vi "Rb_HSRL_v1.0.vi"() -> ()   [LabVIEW 2012]
uses:
  C:/Users/H2ODial/Desktop/Shared Telescope WV DIAL Code/Libraries and VIs/PowerMeterCommands.dll
  Shared Telescope WV DIAL Code/Libraries and VIs/PowerMeterCommands.dll
  <vilib>/DAQmx/write.llb/DAQmx Write (Digital 1D Bool NChan 1Samp 1Line).vi
  <vilib>/DAQmx/miscellaneous.llb/DAQmx Fill In Error Info.vi
  <vilib>/Analysis/baseanly.llb/Mean (DBL).vi
  NCAR_DIAL_Labview/AMCS_Data.vi
  Libraries and VIs/Scalar_Data.vi
  <vilib>/Analysis/NI_AALBase.lvlib
  Libraries and VIs/Scalar_Data_2.vi
  Libraries and VIs/Scalar_Data_4.vi
  Libraries and VIs/Scalar_Data_3.vi
  Shared Telescope WV DIAL Code/bristol/CLDevIFace.dll
panel:
  out "FileHour":i32
  out "L_Count":i32=1074
  out "sigma_off_total":dbl[](array[numeric])=[1.743240222676567e-29, 1.7305064234520192e-29, 1.7178428488017876e-29, 1.705249234754588e-29, 1.692725317927625e-29, 1.6802708355255098e-29, 1.6678855253392072e-29, 1.6555691257449675e-29, 1.643321375703259e-29, 1.631142014757713e-29, 1.619030783034076e-29, 1.6069874212391396e-29, 1.5950116706597008e-29, 1.5831032731615155e-29, 1.5712619711882448e-29, 1.5594875077604192e-29, 1.5477796264743928e-29, 1.536138071501325e-29, 1.5245625875861102e-29, 1.5130529200463784e-29, 1.5016088147714616e-29, 1.4902300182213635e-29, 1.4789162774257317e-29, 1.4676673399828526e-29, 1.4564829540586228e-29, 1.4453628683855395e-29, 1.4343068322617087e-29, 1.423314595549802e-29, 1.412385908676087e-29, 1.401520522629413e-29, 1.3907181889602167e-29, 1.3799786597795178e-29, 1.3693016877579533e-29, 1.3586870261247614e-29, 1.3481344286668248e-29, 1.3376436497276693e-29, 1.3272144442065002e-29, 1.3168465675572225e-29, 1.306539775787476e-29, 1.2962938254576631e-29, 1.2861084736799932e-29, 1.275983478117514e-29, 1.2659185969831725e-29, 1.255913589038839e-29, 1.2459682135943853e-29, 1.2360822305067216e-29, 1.226255400178859e-29, 1.2164874835589805e-29, 1.2067782421394965e-29, 1.1971274379561291e-29, 1.1875348335869746e-29, 1.178000192151585e-29, 1.1685232773100587e-29, 1.159103853262107e-29, 1.1497416847461672e-29, 1.1404365370384833e-29, 1.1311881759522077e-29, 1.1219963678364997e-29, 1.1128608795756442e-29, 1.1037814785881385e-29, 1.0947579328258326e-29, 1.0857900107730373e-29, 1.0768774814456401e-29, 1.0680201143902449e-29, 1.059217679683288e-29, 1.050469947930196e-29, 1.0417766902645026e-29, 1.0331376783470095e-29, 1.0245526843649219e-29, 1.0160214810310171e-29, 1.0075438415827858e-29, 9.991195397816067e-30, 9.907483499119049e-30, 9.824300467803266e-30, 9.741644057149123e-30, 9.659512025642775e-30, 9.577902136968061e-30, 9.496812159998168e-30, 9.416239868787793e-30, 9.336183042565099e-30, 9.256639465723581e-30, 9.177606927814325e-30, 9.099083223538087e-30, 9.021066152737376e-30, 8.94355352038878e-30, 8.866543136595263e-30, 8.790032816578293e-30, 8.714020380670432e-30, 8.638503654307654e-30, 8.563480468021747e-30, 8.488948657432945e-30, 8.414906063242409e-30, 8.34135053122489e-30, 8.268279912221336e-30, 8.195692062131722e-30, 8.123584841907613e-30, 8.051956117545193e-30, 7.980803760078008e-30, 7.910125645569903e-30, 7.839919655108038e-30, 7.77018367479582e-30, 7.700915595746074e-30, 7.632113314074101e-30, 7.563774730890895e-30, 7.49589775229633e-30, 7.42848028937248e-30, 7.361520258176989e-30, 7.295015579736328e-30, 7.228964180039413e-30, 7.163363990030974e-30, 7.098212945605153e-30, 7.03350898759913e-30, 6.969250061786685e-30, 6.905434118872086e-30, 6.84205911448366e-30, 6.779123009167796e-30, 6.716623768382682e-30, 6.654559362492305e-30, 6.592927766760486e-30, 6.531726961344797e-30, 6.470954931290802e-30, 6.410609666526129e-30, 6.350689161854694e-30, 6.291191416951005e-30, 6.232114436354457e-30, 6.173456229463735e-30, 6.1152148105312555e-30, 6.05738819865764e-30, 5.999974417786303e-30, 5.942971496698029e-30, 5.88637746900568e-30, 5.830190373148922e-30, 5.774408252388966e-30, 5.71902915480344e-30, 5.664051133281335e-30, 5.609472245517892e-30, 5.555290554009665e-30, 5.501504126049601e-30, 5.448111033722145e-30, 5.395109353898468e-30, 5.342497168231712e-30, 5.290272563152322e-30, 5.238433629863349e-30, 5.186978464335997e-30, 5.135905167305021e-30, 5.085211844264311e-30, 5.0348966054625156e-30, 4.984957565898723e-30, 4.935392845318121e-30, 4.886200568207903e-30, 4.837378863793033e-30, 4.788925866032188e-30, 4.74083971361372e-30, 4.693118549951716e-30, 4.6457605231820746e-30, 4.598763786158649e-30, 4.552126496449484e-30, 4.5058468163330804e-30, 4.45992291279475e-30, 4.4143529575229735e-30, 4.369135126905908e-30, 4.3242676020278865e-30, 4.279748568665977e-30, 4.2355762172866776e-30, 4.191748743042563e-30, 4.148264345769089e-30, 4.1051212299814194e-30, 4.0623176048712705e-30, 4.019851684303927e-30, 3.97772168681519e-30, 3.935925835608487e-30, 3.894462358551995e-30, 3.853329488175855e-30, 3.812525461669358e-30, 3.772048520878381e-30, 3.7318969123026464e-30, 3.692068887093256e-30, 3.6525627010501435e-30, 3.613376614619627e-30, 3.574508892892104e-30, 3.535957805599667e-30, 3.497721627113887e-30, 3.459798636443609e-30, 3.422187117232841e-30, 3.384885357758682e-30, 3.3478916509293096e-30, 3.311204294282027e-30, 3.274821589981408e-30, 3.2387418448174616e-30, 3.2029633702038674e-30, 3.16748448217627e-30, 3.1323035013906723e-30, 3.097418753121829e-30, 3.0628285672617353e-30, 3.028531278318176e-30, 2.994525225413349e-30, 2.9608087522825017e-30, 2.92738020727268e-30, 2.8942379433414807e-30, 2.861380318055985e-30, 2.8288056935915537e-30, 2.7965124367308904e-30, 2.7644989188630092e-30, 2.7327635159823654e-30, 2.7013046086879812e-30, 2.6701205821826584e-30, 2.6392098262722643e-30, 2.60857073536503e-30, 2.5782017084709586e-30, 2.5481011492012757e-30, 2.518267465767932e-30, 2.48869907098315e-30, 2.459394382259084e-30, 2.4303518216074538e-30, 2.4015698156393544e-30, 2.373046795564983e-30, 2.3447811971935587e-30, 2.3167714609331835e-30, 2.2890160317908673e-30, 2.261513359372517e-30, 2.2342618978830647e-30, 2.207260106126574e-30, 2.180506447506479e-30, 2.1539993900258164e-30, 2.1277374062875614e-30, 2.1017189734949946e-30, 2.075942573452137e-30, 2.050406692564209e-30, 2.0251098218382186e-30, 2.0000504568835075e-30, 1.97522709791245e-30, 1.9506382497411197e-30, 1.9262824217900777e-30, 1.90215812808518e-30, 1.8782638872584395e-30, 1.8545982225489656e-30, 1.8311596618039416e-30, 1.8079467374796337e-30, 1.7849579866425135e-30, 1.7621919509703503e-30, 1.7396471767534394e-30, 1.7173222148958272e-30, 1.695215620916613e-30, 1.6733259549512735e-30, 1.6516517817530943e-30, 1.6301916706945917e-30, 1.608944195769015e-30, 1.587907935591907e-30, 1.5670814734026938e-30, 1.5464633970663293e-30, 1.5260522990750085e-30, 1.5058467765498978e-30, 1.4858454312429449e-30, 1.466046869538705e-30, 1.4464497024562426e-30, 1.4270525456510766e-30, 1.4078540194171561e-30, 1.3888527486888854e-30, 1.3700473630432205e-30, 1.3514364967017896e-30, 1.3330187885330481e-30, 1.3147928820545087e-30, 1.2967574254349875e-30, 1.2789110714969318e-30, 1.2612524777187339e-30, 1.2437803062371468e-30, 1.2264932238497042e-30, 1.209389902017198e-30, 1.1924690168662101e-30, 1.1757292491916402e-30, 1.159169284459339e-30, 1.1427878128087242e-30, 1.1265835290554763e-30, 1.110555132694241e-30, 1.0947013279014056e-30, 1.0790208235378844e-30, 1.063512333151953e-30]
  out "sigma_on_total":dbl[](array[numeric])=[2.4340017477146767e-23, 2.4274412818663494e-23, 2.420732288097601e-23, 2.4138763171607075e-23, 2.4068749611971555e-23, 2.3997298524358964e-23, 2.3924426624079916e-23, 2.3850151008686397e-23, 2.3774489143132373e-23, 2.3697458852913156e-23, 2.36190783110143e-23, 2.3539366026312405e-23, 2.3458340830704462e-23, 2.3376021868838044e-23, 2.3292428585503507e-23, 2.3207580713450583e-23, 2.3121498259428018e-23, 2.3034201496227212e-23, 2.2945710944104806e-23, 2.2856047362675843e-23, 2.2765231738320447e-23, 2.2673285267646947e-23, 2.2580229349833727e-23, 2.248608556893553e-23, 2.2390875685659293e-23, 2.2294621622467176e-23, 2.2197345450376258e-23, 2.2099069377470227e-23, 2.1999815736348355e-23, 2.1899606971079585e-23, 2.1798465624791464e-23, 2.169641432790326e-23, 2.1593475784788012e-23, 2.14896727633276e-23, 2.1385028081251008e-23, 2.1279564594830037e-23, 2.1173305187714593e-23, 2.1066272759361542e-23, 2.0958490211415564e-23, 2.084998043979143e-23, 2.0740766320851033e-23, 2.0630870703286357e-23, 2.0520316394136837e-23, 2.0409126151062488e-23, 2.029732266933444e-23, 2.0184928575611705e-23, 2.0071966414278353e-23, 1.995845864002376e-23, 1.9844427607378718e-23, 1.9729895562122156e-23, 1.9614884633458083e-23, 1.949941682266462e-23, 1.9383513996314403e-23, 1.9267197878653387e-23, 1.9150490042628342e-23, 1.903341190278002e-23, 1.8915984707328566e-23, 1.8798229531581053e-23, 1.868016727054153e-23, 1.8561818633359694e-23, 1.844320413541846e-23, 1.83243440938274e-23, 1.8205258619529394e-23, 1.8085967614344843e-23, 1.796649076411767e-23, 1.7846847532669082e-23, 1.772705716009478e-23, 1.7607138654671335e-23, 1.748711079164774e-23, 1.736699210720163e-23, 1.724680089518985e-23, 1.712655520363638e-23, 1.7006272832450093e-23, 1.6885971328406567e-23, 1.676566798384533e-23, 1.6645379834582855e-23, 1.6525123654654852e-23, 1.64049159581075e-23, 1.6284772994189594e-23, 1.6164710746660405e-23, 1.6044744932804177e-23, 1.592489100169575e-23, 1.5805164132216785e-23, 1.568557923455707e-23, 1.556615094674276e-23, 1.544689363604575e-23, 1.5327821398683183e-23, 1.5208948058333225e-23, 1.5090287167129152e-23, 1.4971852006339355e-23, 1.4853655585856495e-23, 1.473571064476312e-23, 1.4618029653368368e-23, 1.4500624811408796e-23, 1.4383508052135306e-23, 1.4266691041242847e-23, 1.4150185179015395e-23, 1.4034001601711465e-23, 1.3918151181804494e-23, 1.380264453258343e-23, 1.3687492006081647e-23, 1.3572703697882705e-23, 1.3458289448210642e-23, 1.334425884233711e-23, 1.323062121559879e-23, 1.3117385653560717e-23, 1.3004560994740862e-23, 1.2892155833393701e-23, 1.2780178521172943e-23, 1.2668637170454652e-23, 1.2557539657303056e-23, 1.2446893622178752e-23, 1.233670647459471e-23, 1.2226985395093895e-23, 1.2117737338433009e-23, 1.2008969034936782e-23, 1.1900686995645521e-23, 1.1792897514105055e-23, 1.1685606668968417e-23, 1.1578820327003693e-23, 1.1472544147196505e-23, 1.1366783583055892e-23, 1.1261543884626321e-23, 1.1156830104040547e-23, 1.105264709614388e-23, 1.0948999523006647e-23, 1.0845891856006974e-23, 1.0743328380652776e-23, 1.0641313197997005e-23, 1.053985022811714e-23, 1.0438943213901274e-23, 1.0338595723501814e-23, 1.0238811153778875e-23, 1.0139592733083218e-23, 1.004094352498993e-23, 9.942866430738372e-24, 9.845364192310422e-24, 9.748439395492984e-24, 9.652094473529007e-24, 9.556331709814775e-24, 9.46115323999935e-24, 9.366561056469104e-24, 9.272557009807764e-24, 9.179142813204785e-24, 9.086320043893727e-24, 8.99409014719721e-24, 8.902454438513804e-24, 8.811414107270266e-24, 8.7209702177534e-24, 8.631123714110481e-24, 8.541875421413822e-24, 8.453226049192974e-24, 8.365176194357096e-24, 8.277726342238635e-24, 8.190876871321929e-24, 8.104628054224402e-24, 8.018980061019835e-24, 7.933932961475672e-24, 7.849486727271008e-24, 7.76564123493127e-24, 7.682396268209798e-24, 7.59975151947134e-24, 7.517706593480449e-24, 7.436261008471844e-24, 7.355414199356734e-24, 7.275165518527386e-24, 7.1955142399073e-24, 7.116459559687598e-24, 7.038000598677644e-24, 6.960136404824994e-24, 6.882865955014892e-24, 6.806188156632044e-24, 6.730101850609514e-24, 6.65460581162548e-24, 6.579698751718169e-24, 6.505379321481059e-24, 6.4316461112652594e-24, 6.358497654002827e-24, 6.285932426130069e-24, 6.213948849912267e-24, 6.142545294327772e-24, 6.071720077707449e-24, 6.001471468939084e-24, 5.9317976881000545e-24, 5.862696910102476e-24, 5.7941672637438124e-24, 5.726206835260677e-24, 5.658813668292153e-24, 5.591985766579753e-24, 5.525721094088758e-24, 5.460017577095787e-24, 5.394873105681451e-24, 5.330285534503123e-24, 5.266252684077375e-24, 5.202772342694521e-24, 5.139842266622448e-24, 5.077460182290799e-24, 5.0156237866223426e-24, 4.954330748813029e-24, 4.893578710949848e-24, 4.8333652890974455e-24, 4.773688074662277e-24, 4.714544635557992e-24, 4.655932516447053e-24, 4.597849240182404e-24, 4.540292309191013e-24, 4.483259205518585e-24, 4.42674739232282e-24, 4.370754314606057e-24, 4.315277399935558e-24, 4.2603140594233714e-24, 4.205861688673324e-24, 4.151917668300883e-24, 4.098479364843186e-24, 4.045544131381291e-24, 3.993109308279057e-24, 3.941172224403115e-24, 3.8897301970479374e-24, 3.838780532877164e-24, 3.788320529066769e-24, 3.738347472966815e-24, 3.6888586436966916e-24, 3.639851312259568e-24, 3.59132274213381e-24, 3.543270189847801e-24, 3.495690905760268e-24, 3.448582134258885e-24, 3.401941114510703e-24, 3.355765080859501e-24, 3.310051263532474e-24, 3.2647968887967694e-24, 3.219999179434413e-24, 3.175655355707198e-24, 3.1317626351721278e-24, 3.0883182332206364e-24, 3.045319363885891e-24, 3.002763239842466e-24, 2.9606470728961763e-24, 2.9189680744537877e-24, 2.8777234556990287e-24, 2.8369104281330918e-24, 2.7965262038221122e-24, 2.756567995816512e-24, 2.7170330182075216e-24, 2.677918486705564e-24, 2.6392216190184846e-24, 2.6009396347182876e-24, 2.5630697559473515e-24, 2.52560920743859e-24, 2.4885552169425194e-24, 2.451905015320653e-24, 2.415655836797415e-24, 2.3798049195052113e-24, 2.3443495052514497e-24, 2.3092868400499548e-24, 2.274614174185544e-24, 2.24032876263913e-24, 2.2064278649970267e-24, 2.1729087457232614e-24, 2.139768674486092e-24, 2.107004926331989e-24, 2.0746147815906223e-24, 2.0425955263802693e-24, 2.0109444525036206e-24, 1.9796588577379595e-24, 1.9487360460458536e-24, 1.9181733275318523e-24, 1.887968018650247e-24, 1.858117442578046e-24, 1.8286189289240917e-24, 1.799469814155742e-24, 1.7706674416008516e-24, 1.742209161621556e-24, 1.7140923316697854e-24, 1.6863143164506015e-24, 1.658872488023585e-24, 1.6317642257456694e-24]
  out "background start":u32=254
  in  "Tab Control 2":enum32{"WV ND narrow", "WV ND wide"}(tab)=enum."WV ND wide"
  out "Water Vapor Number Density":dbl[][](graph)=[[nan, nan, nan, nan, nan, nan, nan, nan, nan, nan, nan, nan, nan, nan, nan, nan, nan, nan, nan, nan, nan, nan, nan, nan, nan, nan, nan, nan, nan, nan, nan, nan, nan, nan, nan, nan, nan, nan, nan, nan, nan, nan, nan, nan, nan, nan, nan, nan, nan, nan, nan, nan, nan, nan, nan, nan, nan, nan, nan, nan, nan, nan, nan, nan, nan, nan, nan, nan, nan, nan, nan, nan, nan, nan, nan, nan, nan, nan, nan, nan, nan, nan, nan, nan, nan, nan, nan, nan, nan, nan, nan, nan, nan, nan, nan, nan, nan, nan, nan, nan, nan, nan, nan, nan, nan, nan, nan, nan, nan, nan, nan, nan, nan, nan, nan, nan, nan, nan, nan, nan, nan, nan, nan, nan, nan, nan, nan, nan, nan, nan, nan, nan, nan, nan, nan, nan, nan, nan, nan, nan, nan, nan, nan, nan, nan, nan, nan, nan, nan, nan, nan, nan, nan, nan, nan, nan, nan, nan, nan, nan, nan, nan, nan, nan, nan, nan, nan, nan, nan, nan, nan, nan, nan, nan, nan, nan, nan, nan, nan, nan, nan, nan, nan, nan, nan, nan, nan, nan, nan, nan, nan, nan, nan, nan, nan, nan, nan, nan, nan, nan, nan, nan, nan, nan, nan, nan, nan, nan, nan, nan, nan, nan, nan, nan, nan, nan, nan, nan, nan, nan, nan, nan, nan, nan, nan, nan, nan, nan, nan, nan, nan, nan, nan, nan, nan, nan, nan, nan, nan, nan, nan, nan, nan, nan, nan, nan, nan, nan, nan, nan, nan, nan, nan, nan, nan, nan, nan, nan, nan, nan, nan, nan, nan, nan, nan, nan, nan, nan, nan, nan, nan, nan, nan, nan, nan, nan, 0.0, 0.0, 0.0, 0.0]]
  out "Water Vapor Number Density 2":dbl[][](graph)=[[-4.895620784344141, -1.6968761345752499, -1.6565574205993407, -0.7910986719149671, 0.45141531234214655, 0.26569889383172274, 0.252782855220571, 0.5170092395121896, 0.6376366522322393, 0.5993479288564648, 0.6058560998386514, 0.684546234269247, 0.6235793613938562, 0.5332655312275792, 0.5321964157932958, 0.4070943470032037, 0.22619083292346856, 0.25267455894454416, 0.08444579003837588, -0.13682052767692168, -0.09862987130915078, -0.017768894386159955, 0.05643569551164931, -0.08094018405996439, -0.19480945286341145, -0.06075864848776602, 0.06572189033635885, 0.039671145716655434, -0.09019678979226083, -0.25137434776459894, -0.3103489478521125, -0.08024943893293456, 0.06423439301048192, 0.13797237185068356, 0.09652097666493928, -0.27218358000621307, -0.185543414642533, 0.1438017744018525, 0.08765450079199422, -0.03345732408225611, 0.00604196903795461, 0.08267162189631926, 0.08321350242218584, -0.012409724836985615, 0.09179545659027583, 0.6459182960375515, 2.2714138304504465, 4.472080283472494, 6.069123607220832, 6.990920567565342, 7.36854640140037, 7.533827768908647, 7.78681047271232, 8.16977657612961, 8.33947543641484, 8.20492227081218, 7.344734807648823, 5.975728267693901, 4.780051696796776, 3.7740123495138187, 2.9280932285169685, 2.0539593404341003, 1.0507395625011602, 0.24983625755292468, -0.03087360168049576, -0.09871712906759823, -0.5243136500273711, -1.1240686267268338, -1.2357380560289242, -1.4422719214455215, -2.433215702684351, -3.945832400189159, -5.949204291924275, -8.114157844867002, -9.494648146574068, -10.507339423422904, -10.700994135914522, -10.9541924360514, -11.159957626803134, -10.310413019639286, -8.273713586301556, -4.9233609203087365, -1.3825921417412714, 1.9712668900617927, 3.378743922387925, 4.088541358207288, 4.007098488107816, 4.103753213551659, 4.2340431790887845, 4.002951543204611, 3.686717068344896, 2.676317251371432, 1.8649247581896786, 1.0769258052139539, 0.994629537649367, 0.9943831824592358, 1.1926416452348065, 1.5853553556197177, 2.2148625502201704, 3.108204242971333, 4.52975221279031, 6.563140206581805, 9.134431370789654, 10.09902536825411, 7.280234451114133, 10.0523524768224, 11.397964614531503, -9.731550990663491, -17.06321734883455, -11.458184267120643, -9.0017850283161, -13.74567942179605, -16.166537362978502, -18.718196579771735, -9.35381042912264, -12.348971539301585, -12.154938420119997, 5.238619214813352, 9.192709199582309, 14.003999057719604, -0.06779931634937152, 35.617669964692475, 0.04457992374851296, -8.90741561387052, -3.9461882542526, 14.504294890545367, -0.8727026085664153, -0.35102394306834434, 3.597665203572956, -8.777831693534882, -2.954362505813555, -31.9195126702593, -3.8409008890464578, 5.435252259671796, 4.418087258470408, -20.27746959744448, -10.613666063696122, 1.8615584996987187, -7.892452743589819, -16.226094846188996, -2.383169027908074, 16.92726357878285, 5.456643076920959, 14.024204963031833, -11.157368068562498, 4.340391398015347, 3.9438279618064525, 21.09263715399934, 7.680640751435989, -20.993550633072697, -8.585857017075819, -23.52761555750025, -7.7605319523907905, -17.998320270316242, -16.180858157616544, -12.33853742715028, -14.667064184492856, -49.95610957313421, -49.44749566095738, 10.699739375836488, 23.683479637440108, 31.061894932072992, -21.207052348393276, 10.140128391398383, -19.895810174476523, -15.108621152086325, 4.704826625608483, 27.735652107472575, 39.49510870780125, 20.618532855965775, -1.6111370074131892, -12.831734806604826, 15.629932803094974, -14.611823636038348, 29.640524053991733, 5.015161743310881, -15.51797368973543, -40.44577289799667, -0.39722724524646463, -0.9239222044621952, -20.535732365469173, -65.2480323448027, 26.487995182823845, 19.394999803340337, 20.191997873478407, -2.0265210169772954, 24.853618849595346, 42.52208295164487, 12.786859480359054, 4.75017526225865, 17.835930493267455, 52.68824174794205, 34.72243662831497, 6.3260469161335555, -7.486867031209662, 10.759083285233261, -66.51368343207345, -9.431641653132534, -18.76468287635854, -15.650517009171523, -20.26681276234243, -28.565738365359984, -30.121388986694676, -11.448382080381739, -7.859271932595647, 39.94633068089728, 56.860646041958226, 4.524084628014805, 54.8901924570308, 16.546300340318517, 20.97522561665681, 0.05393176717682176, -15.507692065561, -1.4043208940216665, -28.371460993902787, -29.792326994117683, -15.657302207635121, 0.7422373766833459, -20.485527759325585, -8.147758064164341, 18.82463653057326, 28.412517069974978, 8.44635419576539, -41.650375728538094, -5.872699418390108, 1.8094667524442931, 1.5468215804437708, 41.021758843667016, -23.195386516298573, 112.29420310200375, -16.587822198800488, 2.3654789897656885, -23.460726710726124, 91.52185335985529, 22.81580178981554, 27.176228351401313, -5.556802132037837, -63.630574940001445, 17.09067007327093, -40.44093778205592, -14.862030911568922, -43.05400894140326, -66.35104817070908, -65.39879656619192, 1.787225500718848, -42.55071677898285, -1.0319246177540415, 25.14429634118871, -1.541432028680571, -11.550238337108132, 11.139244631605925, 40.46635926020925, 127.44307434312368, -10.216664862682935, 11.539137763811313, 53.24251481088911, 71.08979732730369, 9.04286335401417, -73.54684338479775, -128.0577139180142, -86.77985430271906, -75.66005818218412, -37.36514333604306, 5.847510175807278, 19.206208021208408, -129.3901968796948, -67.23722677793343, -51.592749749275896, 98.36383603903877, 82.4204245579684, 78.16287004109239, 71.76344715659785, -14.203962783305958, 19.040423726184862, -15.217180976533145, 88.48290659710524, 0.0, 0.0, 0.0, 0.0]] caption="Water Vapor Number Density"
  out "RingBuffer offline near":dbl[][](array[numeric])
  out "RingBuffer aerosol near":dbl[][](array[numeric])
  in  "?":T1(tab)=enum."Raw Counts combined"
  out "NRB":dbl[][](graph) caption="Water Vapor Number Density"
  out "NRB 2":dbl[][](graph)=[[0.0001380506377637834, 0.00037231338536795606, 0.0008267018556340546, 0.0016491182628392146, 0.0030984002727663757, 0.0054670319322802745, 0.008975049813494944, 0.013862611097666086, 0.020640714712243713, 0.030032261963369757, 0.041790885354449886, 0.05646823982524779, 0.07405765547049918, 0.09445230634842686, 0.11873844907566593, 0.14619202991112218, 0.176128716495472, 0.2065930967214025, 0.23772953608021488, 0.2712999788026663, 0.303183374769058, 0.33461849194542187, 0.36556675325880467, 0.3928286709332662, 0.4196893863731421, 0.4471637143514717, 0.47287194470451144, 0.4890446444671604, 0.5073163767400038, 0.527833117627229, 0.5384928838328282, 0.5504358197236068, 0.5590875545865447, 0.5635018660373124, 0.5701363166467346, 0.5747236095368302, 0.5814440483526132, 0.5919810946272498, 0.5989836077128905, 0.6020509020058386, 0.6120157766394789, 0.6121904103347232, 0.6014357977759414, 0.6025641696641967, 0.6063884095863453, 0.6028169859903434, 0.5986429081300412, 0.602926751521262, 0.6045234286166641, 0.6020772298885957, 0.6093012321904592, 0.6071420602133842, 0.6000004559925828, 0.6074015253593915, 0.6308874815821919, 1.447719815623411, 5.0092251256615326, 10.608207780798377, 12.51719597789648, 9.217607568444715, 8.012447829214926, 15.43698184887009, 26.6065389573323, 30.108057890606787, 25.881596466733146, 22.37376849180048, 20.71552585543168, 17.29780957584456, 13.067263761054791, 9.970369103635118, 8.373569316919895, 8.097534835118013, 8.865992103907578, 12.770957329400636, 18.09781429592472, 17.53337121539854, 10.90234029608704, 5.0392553254119274, 2.373505404868523, 1.0991203310287527, 0.45466930792063653, 0.28635282734262657, 0.2684584174682796, 0.27254175669170166, 0.2642432011850105, 0.27155612117614053, 0.3573074050799282, 0.5675591029962431, 0.9568718981502712, 1.8781004463984938, 3.832184351648157, 7.296157287404594, 12.992486225144889, 19.850044811959783, 23.876263508247536, 22.89971699362709, 18.57735815186402, 13.384467836450757, 9.941618607703871, 9.52963656189712, 9.878467461835443, 7.9906667301038645, 4.637172445889551, 2.3432986610499698, 1.878226967282488, 2.3880704072998435, 3.002081888496057, 3.3688062310053652, 3.1265041118362116, 2.369963919278849, 1.4049354414439597, 0.5981477861656775, 0.2201236171481549, 0.10053280018296205, 0.1049539926912024, 0.13605859526889652, 0.14285523134540867, 0.10850858158417578, 0.11616513852327509, 0.14725243241889766, 0.09034956192428265, 0.05961502498241574, 0.08744308907061056, 0.12774569879993047, 0.10342822758481597, 0.10781611837641128, 0.10691828988405683, 0.09844828534015804, 0.13126962561795, 0.10477355228922058, 0.08314270506167556, 0.11068192501635618, 0.1469623872315277, 0.08836483775676496, 0.10655458852918881, 0.15225529874509575, 0.08430787264863451, 0.07009979544767103, 0.08181048165478563, 0.06279693670038371, 0.09328596080458845, 0.09038165610259435, 0.08327020474676582, 0.025684897874086683, 0.0009707833337049407, 0.10225629353341592, 0.1005694755351202, 0.14729024890638545, 0.12365825337171389, 0.025079453252945572, 0.028677777816976682, 0.027515990565747148, 0.054454687532889845, 0.04453495073347162, 0.017382194343326905, -0.04252219295217604, -0.07058050401235756, -0.02456764397335006, -0.028497208807347345, 0.015346829492512202, 0.04298797788120953, 0.01623362898624638, 0.08563204153282877, 0.004064284667093428, -0.10133064618333942, 0.05253453070798904, 0.06514225667556629, 0.042499199608995515, 0.09968168750325075, 0.004918514915909139, -0.00032358694526253486, 0.06289222078475586, 0.059342770479511635, 0.13657348927840832, 0.1770073767458159, 0.07264829002326911, 0.08483375293471081, 0.21365900428087206, 0.04152199871116299, 0.0222051701557016, 0.15278405108610074, 0.1415202788910293, 0.14467720700616699, 0.1294668069955981, 0.09953241260822868, 0.05077385822206056, 0.11437335389791674, 0.0174792549892461, -0.12170754523984625, -0.024506540953794162, -0.006320084684789309, -0.03276198538429077, 0.004207338523473438, 0.013227107986545533, 0.06523808909079482, -0.024979323976464695, -0.04263554157486385, 0.07698508208616586, 0.0006951280918226639, -0.09660263950948868, -0.03937413525317987, 0.06805955659081427, 0.05222342809633812, -0.12035517959868296, -0.1708478846518318, 0.0023642220353940827, 0.14259926575817566, 0.08083030570322937, -0.127577324988055, -0.16119409412364716, 0.06364108456905275, 0.3386672374669003, 0.2622252302230505, 0.07857050698230215, 0.12340568076001972, 0.05734592250065322, 0.08977349820396631, 0.22616670263325436, 0.07953961680339071, -0.18706894477447125, -0.2018189311229299, -0.08047192233842872, 0.07250896970261306, 0.12342245188602205, 0.13225442113834784, 0.12368717459399005, 0.09676342875464072, 0.008847199978845019, -0.06111354456473662, 0.049880628408371486, 0.08951323251928896, 0.034320613803925794, -0.04514061816559589, -0.01470972019166381, 0.005184082507240442, 0.025418931716203685, 0.0733253763222838, 0.08853584410979902, 0.15903378151183248, 0.22466106785463236, 0.11627032735247014, 0.02672784970245174, 0.10243485082245009, 0.007292657881859975, -0.020133574716629028, 0.11652624886483087, 0.05810881426073248, 0.03511053047002674, 0.13003259048413732, 0.05118148463654222, 0.13814021686570216, 0.15620654066824666, -0.10085146919722136, -0.10903579404468894, 0.02347325591345995, 0.11868986701645191, 0.19775337697257164, 0.2786752450542533, 0.24564109985016588, 0.12565244407857296, 0.03303914164600584, 0.08306213435353355, -0.005384461142077131, 0.00853717219386779, 0.10239382246508076, -0.11215691172352353, -0.12932346222779006, -0.12686812690414423, -0.22859894560534677, -0.26090034021168024, -0.2817521949784425, -0.06575148455597245, 0.19185794565702205, 0.29998635760771497, 0.06048668116730433, -0.09822080237649826, -0.12528467918807926, 0.0, 0.0, 0.0]] caption="Water Vapor Number Density"
  out "raw counts":dbl[][](graph) caption="Water Vapor Number Density"
  out "raw counts near":dbl[][](graph)=[[155.92000000000002, 92.92, 94.92, 74.92, 108.92, 117.92, 192.92000000000002, 173.92000000000002, 224.92000000000002, 239.92000000000002, 293.92, 374.92, 383.92, 427.92, 461.92, 541.92, 520.92, 526.92, 632.92, 656.92, 621.92, 635.92, 638.92, 660.92, 601.92, 587.92, 584.92, 592.92, 532.92, 566.92, 510.92, 531.92, 507.92, 460.92, 445.92, 423.92, 421.92, 367.92, 395.92, 372.92, 322.92, 356.92, 319.92, 280.92, 302.92, 259.92, 269.92, 242.92000000000002, 283.92, 255.92000000000002, 230.92000000000002, 198.92000000000002, 184.92000000000002, 194.92000000000002, 212.92000000000002, 198.92000000000002, 351.92, 1825.92, 2550.92, 1728.92, 1368.92, 3407.92, 6903.92, 11887.92, 13882.92, 13623.92, 13034.92, 9068.92, 5196.92, 4147.92, 2973.92, 1874.92, 1142.92, 1749.92, 5473.92, 8307.92, 6691.92, 3420.92, 1268.92, 430.92, 101.92, 24.92, 25.92, 2.9200000000000017, 8.920000000000002, 12.920000000000002, 15.920000000000002, 68.92, 102.92, 98.92, 72.92, 61.92, 121.92, 223.92000000000002, 518.92, 774.92, 840.92, 877.92, 844.92, 591.92, 303.92, 266.92, 194.92000000000002, 165.92000000000002, 141.92000000000002, 111.92, 112.92, 124.92, 206.92000000000002, 202.92000000000002, 149.92000000000002, 24.92, 14.920000000000002, 15.920000000000002, 2.9200000000000017, -6.079999999999998, -13.079999999999998, 0.9200000000000017, -19.08, 11.920000000000002, -16.08, 10.920000000000002, -0.0799999999999983, 7.920000000000002, 10.920000000000002, 11.920000000000002, -4.079999999999998, 26.92, -6.079999999999998, 12.920000000000002, 13.920000000000002, -7.079999999999998, 7.920000000000002, 9.920000000000002, 15.920000000000002, -3.0799999999999983, 1.9200000000000017, -4.079999999999998, 14.920000000000002, 2.9200000000000017, -4.079999999999998, -7.079999999999998, 2.9200000000000017, 6.920000000000002, 7.920000000000002, 2.9200000000000017, -2.0799999999999983, 1.9200000000000017, 15.920000000000002, -3.0799999999999983, -9.079999999999998, 11.920000000000002, 7.920000000000002, -12.079999999999998, 5.920000000000002, 3.9200000000000017, -7.079999999999998, -0.0799999999999983, -24.08, -5.079999999999998, 4.920000000000002, -6.079999999999998, 3.9200000000000017, -14.079999999999998, -1.0799999999999983, -6.079999999999998, -7.079999999999998, 3.9200000000000017, 5.920000000000002, 6.920000000000002, 12.920000000000002, 15.920000000000002, -0.0799999999999983, -0.0799999999999983, -0.0799999999999983, -7.079999999999998, -0.0799999999999983, 2.9200000000000017, -22.08, -1.0799999999999983, 4.920000000000002, 1.9200000000000017, -10.079999999999998, -8.079999999999998, 7.920000000000002, 17.92, 1.9200000000000017, -2.0799999999999983, -1.0799999999999983, -7.079999999999998, 3.9200000000000017, -4.079999999999998, 0.9200000000000017, -2.0799999999999983, -10.079999999999998, 0.9200000000000017, 4.920000000000002, 9.920000000000002, -21.08, 19.92, -12.079999999999998, 1.9200000000000017, -8.079999999999998, -7.079999999999998, 29.92, -4.079999999999998, -2.0799999999999983, -0.0799999999999983, -6.079999999999998, -1.0799999999999983, -8.079999999999998, -4.079999999999998, -6.079999999999998, 1.9200000000000017, 6.920000000000002, 12.920000000000002, 2.9200000000000017, 8.920000000000002, -0.0799999999999983, 8.920000000000002, -12.079999999999998, -11.079999999999998, -1.0799999999999983, 4.920000000000002, -1.0799999999999983, 12.920000000000002, -3.0799999999999983, 17.92, -4.079999999999998, -12.079999999999998, 0.9200000000000017, -18.08, 4.920000000000002, 19.92, 11.920000000000002, -14.079999999999998, -3.0799999999999983, 2.9200000000000017, -4.079999999999998, 8.920000000000002, 12.920000000000002, -0.0799999999999983, -6.079999999999998, -15.079999999999998, -4.079999999999998, 3.9200000000000017, 8.920000000000002, -2.0799999999999983, -6.079999999999998, -6.079999999999998, -0.0799999999999983, -3.0799999999999983, 0.9200000000000017, 5.920000000000002, -17.08, 16.92, 8.920000000000002, -7.079999999999998, -17.08, -3.0799999999999983, -3.0799999999999983, 1.9200000000000017, -4.079999999999998, -12.079999999999998, -3.0799999999999983, -5.079999999999998, 7.920000000000002, 1.9200000000000017, 5.920000000000002, 10.920000000000002, 6.920000000000002, -2.0799999999999983, 9.920000000000002, -22.08, -3.0799999999999983, 12.920000000000002, -3.0799999999999983, 15.920000000000002, 1.9200000000000017, 0.0]] caption="Water Vapor Number Density"
  out "HSRL combined Smoothed":dbl[](array[numeric])=[122.52406779661018, 82.63423728813558, 81.54949152542372, 91.49864406779659, 110.00711864406779, 134.76983050847457, 162.51559322033893, 192.14271186440672, 225.99016949152536, 266.2613559322033, 306.11728813559307, 347.45627118644063, 388.1596610169492, 426.73593220338995, 467.17661016949165, 505.3969491525425, 539.2274576271188, 564.0664406779663, 582.4732203389833, 599.8376271186443, 607.9732203389831, 611.3800000000001, 611.1088135593222, 603.1342372881356, 593.8969491525424, 585.0749152542376, 573.7783050847459, 551.8630508474578, 533.7528813559325, 518.9901694915256, 495.9477966101696, 475.82915254237304, 454.5325423728815, 431.6427118644069, 412.18508474576277, 392.7952542372882, 376.24440677966106, 363.2020338983051, 348.93084745762707, 333.4393220338982, 322.6511864406778, 307.5918644067795, 288.3376271186439, 275.92237288135584, 265.4901694915253, 252.60033898305076, 240.31220338983042, 232.066440677966, 223.29525423728808, 213.60033898305082, 207.77830508474574, 199.1681355932203, 189.48169491525417, 184.78677966101685, 185.01559322033887, 408.8545762711863, 1355.8630508474578, 2744.3969491525413, 3120.5240677966085, 2236.863050847457, 1886.142711864407, 3475.625762711865, 5703.541016949153, 6228.642711864408, 5231.007118644069, 4413.651186440678, 3978.659661016948, 3243.346101694914, 2394.930847457627, 1783.6850847457629, 1459.659661016949, 1373.4901694915252, 1461.9477966101695, 2040.447796610169, 2798.8884745762707, 2643.8037288135592, 1613.964745762712, 731.8037288135594, 336.9986440677966, 152.3884745762711, 61.53254237288135, 37.8206779661017, 34.60881355932203, 34.30372881355932, 32.48169491525423, 32.60881355932203, 41.922372881355926, 65.07491525423728, 107.22745762711862, 205.6596610169491, 409.84610169491526, 761.4477966101695, 1321.3969491525422, 1966.5833898305082, 2309.9562711864405, 2171.820677966102, 1731.464745762712, 1226.7698305084746, 895.108813559322, 841.2783050847459, 854.8037288135595, 678.8461016949154, 387.1766101694916, 192.1850847457627, 151.16813559322026, 188.54101694915238, 232.5325423728812, 256.08338983050834, 233.3630508474575, 173.7698305084745, 101.21898305084744, 42.34610169491525, 15.3122033898305, 6.871525423728807, 7.049491525423722, 8.98169491525423, 9.26983050847457, 6.922372881355925, 7.286779661016943, 9.083389830508468, 5.48169491525423, 3.557966101694908, 5.134237288135585, 7.379999999999992, 5.879999999999992, 6.032542372881348, 5.888474576271179, 5.33762711864406, 7.0071186440677895, 5.5071186440677895, 4.303728813559315, 5.642711864406772, 7.379999999999992, 4.371525423728806, 5.193559322033892, 7.312203389830502, 3.9901694915254167, 3.269830508474569, 3.7613559322033825, 2.8461016949152467, 4.168135593220331, 3.98169491525423, 3.617288135593213, 1.10033898305084, 0.041016949152534954, 4.261355932203382, 4.134237288135585, 5.973220338983044, 4.947796610169485, 0.9901694915254163, 1.117288135593213, 1.0579661016949078, 2.0664406779660944, 1.6681355932203314, 0.6427118644067722, -1.5522033898305159, -2.5437288135593294, -0.8742372881356006, -1.0013559322033974, 0.5325423728813486, 1.4732203389830434, 0.5494915254237214, 2.8630508474576195, 0.13423728813558577, -3.3064406779661093, 1.693559322033891, 2.074915254237281, 1.3376271186440605, 3.10033898305084, 0.1511864406779586, -0.009830508474583777, 1.888474576271179, 1.7613559322033823, 4.0071186440677895, 5.134237288135585, 2.083389830508467, 2.4054237288135516, 5.990169491525416, 1.1511864406779586, 0.6088135593220265, 4.142711864406772, 3.7952542372881277, 3.8376271186440603, 3.3969491525423656, 2.5833898305084677, 1.303728813559315, 2.905423728813552, 0.43932203389829794, -3.0267796610169566, -0.6030508474576346, -0.1538983050847531, -0.7894915254237362, 0.10033898305084002, 0.31220338983050105, 1.5240677966101621, -0.5776271186440753, -0.975932203389838, 1.7444067796610097, 0.015593220338975589, -2.145423728813567, -0.8657627118644142, 1.4816949152542298, 1.1257627118643994, -2.5691525423728887, -3.6115254237288212, 0.04949152542372137, 2.9562711864406706, 1.659661016949145, -2.5945762711864484, -3.2471186440678044, 1.269830508474569, 6.693559322033892, 5.134237288135586, 1.524067796610162, 2.371525423728806, 1.0918644067796537, 1.693559322033891, 4.227457627118637, 1.4732203389830434, -3.433559322033906, -3.670847457627126, -1.4505084745762786, 1.2952542372881282, 2.1850847457627043, 2.3206779661016874, 2.1511864406779586, 1.6681355932203317, 0.15118644067795883, -1.035254237288143, 0.8376271186440604, 1.4901694915254162, 0.5664406779660943, -0.7386440677966176, -0.23864406779661762, 0.08338983050846716, 0.40542372881355193, 1.159661016949145, 1.388474576271179, 2.4732203389830434, 3.464745762711857, 1.778305084745755, 0.4054237288135519, 1.541016949152535, 0.10881355932202652, -0.29796610169492266, 1.7105084745762638, 0.8461016949152468, 0.5071186440677892, 1.8630508474576197, 0.7274576271186366, 1.9477966101694841, 2.1850847457627047, -1.39966101694916, -1.5013559322033971, 0.3206779661016875, 1.6088135593220265, 2.659661016949145, 3.7189830508474504, 3.252881355932196, 1.6511864406779586, 0.4308474576271112, 1.0749152542372808, -0.0691525423728887, 0.10881355932202652, 1.2952542372881282, -1.4081355932203465, -1.611525423728821, -1.5691525423728887, -2.8064406779661093, -3.1793220338983126, -3.4081355932203463, -0.7894915254237364, 2.2867796610169417, 3.549491525423721, 0.7105084745762635, -1.145423728813567, -1.4505084745762789]
  out "HSRL combined":dbl[](array[numeric])=[119.4261281337048, 78.36345403899722, 76.88852367688021, 84.97626740947078, 99.26874651810589, 120.4929805013928, 145.6754317548747, 173.4052367688022, 205.19910863509745, 240.32306406685228, 275.8216713091921, 311.40941504178255, 347.9275208913647, 384.22835654596076, 420.13782729804996, 452.82724233983276, 483.6238997214483, 508.8954874651808, 525.5751532033423, 540.406629526462, 549.05844011142, 552.4135933147627, 551.1127576601666, 545.0152646239549, 537.4498050139271, 527.0709749303617, 514.3425626740944, 497.5375487465179, 481.84534818941484, 466.1030083565458, 447.07236768802215, 428.8453481894149, 409.98880222841206, 392.01526462395526, 374.77431754874635, 358.59465181058476, 342.9748746518104, 325.6447910863508, 309.66568245125325, 296.1141504178271, 283.4860167130918, 271.5946518105849, 260.49437325905285, 249.32445682451242, 239.1183286908077, 228.75481894150408, 217.58072423398323, 209.111364902507, 200.30077994428973, 192.29242339832865, 191.79799442896933, 212.02779944289688, 329.6336490250693, 665.0988300835652, 1321.1266852367696, 2589.597437325907, 4572.029192200557, 6343.986016713094, 6717.097437325907, 5722.538941504177, 4317.65454038997, 3405.1211142061265, 3110.9122005571026, 3012.2005013927574, 2982.5528690807814, 2950.566796657383, 2719.9442339832876, 2279.3954874651827, 1801.5250139275772, 1446.0890807799442, 1301.6099721448472, 1291.0194428969364, 1265.1628969359335, 1249.6433983286913, 1205.8105292479113, 969.1475766016715, 595.8704178272978, 291.88852367687997, 131.91637883008357, 62.34116991643454, 37.90941504178271, 33.119721448467956, 31.722785515320325, 30.622506963788283, 31.557047353760417, 34.85231197771584, 39.364846796657346, 47.45676880222838, 65.65036211699166, 120.88016713091926, 295.68378830083566, 716.1030083565456, 1338.9498050139273, 1910.671253481894, 2205.417771587743, 2176.7297493036212, 1962.703286908078, 1754.2548189415038, 1632.6656824512534, 1575.9108077994429, 1543.0486908077992, 1459.7032869080774, 1281.72557103064, 1063.7896378830078, 856.0445125348186, 663.7269637883005, 505.5208356545959, 389.2659610027854, 286.6447910863509, 181.88295264623946, 91.19075208913647, 34.18796657381618, 10.810529247910864, 3.3857381615598845, 1.1684679665738122, 2.0041225626740906, 3.5570473537604412, 2.150362116991639, 1.8940947075208867, 2.3801671309192156, 3.1030083565459567, 3.3550974930362076, 3.3954874651810543, 4.8049582172701895, 3.1698607242339785, 2.068189415041778, 2.5319777158774324, 2.336991643454035, 1.7743175487465142, 0.5236211699164305, 2.4191643454038956, 2.9665181058495773, 2.118328690807795, 1.314707520891361, 1.4372701949860678, 1.534763231197767, 1.0960445682451214, 2.196323119777155, 1.9818384401114166, 1.4052367688022245, 1.8453481894150376, 2.3328133704735334, 0.9804456824512497, 0.6977158774373221, 1.526406685236765, 0.6628969359331439, -0.7535376044568286, 1.2687465181058455, 3.428913649025066, 2.2645682451253446, 0.7784958217270156, -1.069693593314767, -1.6811142061281377, -1.4527019498607283, -0.622618384401118, -0.059944289693596886, -0.4457381615598923, 2.394094707520887, 2.497158774373255, 0.9177715877437286, 0.16846796657381213, -0.6992200557103102, 0.4637325905292442, 0.2199999999999962, 0.01387186629526077, 0.09465181058495437, 0.23810584958216896, 1.410807799442893, 0.06261838440111012, -1.6407242339832906, -0.04323119777159168, -0.24100278551532428, 1.068189415041779, 2.583509749303617, 1.5305849582172661, 1.3564902506963752, 2.39270194986072, 3.626685236768798, 0.5751532033426143, -0.8064623955431796, -0.10729805013927951, 0.19632311977715505, -0.10033426183844385, -0.03626740947075591, 1.2882451253481855, 0.7353203342618347, 0.5960445682451216, 0.005515320334258111, -2.018161559888583, -2.7521448467966607, -0.2953203342618421, -0.14490250696379203, -1.027910863509753, 0.4456267409470713, 0.6350417827298012, 0.49437325905292095, -0.5696935933147671, -1.1031197771587782, -0.45409470752089515, -1.633760445682455, -2.3830640668523713, -1.231253481894154, 0.002729805013923614, -0.4527019498607281, -0.7437883008356583, 0.21164345403899346, 0.39130919220055344, 0.19214484679665364, -0.3844568245125387, -1.100334261838444, -0.49727019498607616, 1.4080222841225587, 0.814707520891361, 0.2743175487465143, 1.7631754874651773, 1.1141504178272943, -0.6852924791086389, 0.558440111420609, 1.2757103064066815, -0.3538161559888617, -0.2591086350974969, -0.3273537604456863, 0.14061281337046944, 0.6823955431754833, -0.9387743732590567, 0.6141504178272943, 2.398272980501389, -0.6922562674094745, -1.5181615598885834, 0.04033426183843612, 0.24506963788300454, 1.4456267409470716, 0.311922005571027, -1.749359331476327, -1.1825069637883048, 0.655933147632308, 1.343955431754871, 0.8606685236768763, 0.47487465181058125, -0.49587743732590894, -0.9373816155988897, -1.5223398328690845, -0.707576601671313, 0.8286350974930324, 1.7784958217270157, 0.7812813370473501, -0.28417827298050513, -0.22428969359331863, 0.07236768802228039, 0.5236211699164306, 1.313314763231194, 1.5180501392757622, -0.4638440111420651, -2.3955988857938757, -2.4763788300835694, -0.6866852367688063, 1.654540389972141, 2.40245125348189, 1.8161002785515277, 0.46651810584957815, -1.0543732590529287, -1.3524233983286944, -1.6685793871866332, -0.8468523676880263, 0.21442896935932743, 0.2812813370473497, -0.19782729805014335, 0.29520891364902135, 0.8578830083565422, 0.9595543175487425, 0.39270194986071993, -0.1574373259052966, 0.44701949860723855, 0.5417270194986035, 0.7868523676880181, 1.3411699164345363, 0.07793871866294888]
  out "Off-Line Bin Readings 2":dbl[](array[numeric])=[240.0, 177.0, 179.0, 159.0, 193.0, 202.0, 277.0, 258.0, 309.0, 324.0, 378.0, 459.0, 468.0, 512.0, 546.0, 626.0, 605.0, 611.0, 717.0, 741.0, 706.0, 720.0, 723.0, 745.0, 686.0, 672.0, 669.0, 677.0, 617.0, 651.0, 595.0, 616.0, 592.0, 545.0, 530.0, 508.0, 506.0, 452.0, 480.0, 457.0, 407.0, 441.0, 404.0, 365.0, 387.0, 344.0, 354.0, 327.0, 368.0, 340.0, 315.0, 283.0, 269.0, 279.0, 297.0, 283.0, 436.0, 1910.0, 2635.0, 1813.0, 1453.0, 3492.0, 6988.0, 11972.0, 13967.0, 13708.0, 13119.0, 9153.0, 5281.0, 4232.0, 3058.0, 1959.0, 1227.0, 1834.0, 5558.0, 8392.0, 6776.0, 3505.0, 1353.0, 515.0, 186.0, 109.0, 110.0, 87.0, 93.0, 97.0, 100.0, 153.0, 187.0, 183.0, 157.0, 146.0, 206.0, 308.0, 603.0, 859.0, 925.0, 962.0, 929.0, 676.0, 388.0, 351.0, 279.0, 250.0, 226.0, 196.0, 197.0, 209.0, 291.0, 287.0, 234.0, 109.0, 99.0, 100.0, 87.0, 78.0, 71.0, 85.0, 65.0, 96.0, 68.0, 95.0, 84.0, 92.0, 95.0, 96.0, 80.0, 111.0, 78.0, 97.0, 98.0, 77.0, 92.0, 94.0, 100.0, 81.0, 86.0, 80.0, 99.0, 87.0, 80.0, 77.0, 87.0, 91.0, 92.0, 87.0, 82.0, 86.0, 100.0, 81.0, 75.0, 96.0, 92.0, 72.0, 90.0, 88.0, 77.0, 84.0, 60.0, 79.0, 89.0, 78.0, 88.0, 70.0, 83.0, 78.0, 77.0, 88.0, 90.0, 91.0, 97.0, 100.0, 84.0, 84.0, 84.0, 77.0, 84.0, 87.0, 62.0, 83.0, 89.0, 86.0, 74.0, 76.0, 92.0, 102.0, 86.0, 82.0, 83.0, 77.0, 88.0, 80.0, 85.0, 82.0, 74.0, 85.0, 89.0, 94.0, 63.0, 104.0, 72.0, 86.0, 76.0, 77.0, 114.0, 80.0, 82.0, 84.0, 78.0, 83.0, 76.0, 80.0, 78.0, 86.0, 91.0, 97.0, 87.0, 93.0, 84.0, 93.0, 72.0, 73.0, 83.0, 89.0, 83.0, 97.0, 81.0, 102.0, 80.0, 72.0, 85.0, 66.0, 89.0, 104.0, 96.0, 70.0, 81.0, 87.0, 80.0, 93.0, 97.0, 84.0, 78.0, 69.0, 80.0, 88.0, 93.0, 82.0, 78.0, 78.0, 84.0, 81.0, 85.0, 90.0, 67.0, 101.0, 93.0, 77.0, 67.0, 81.0, 81.0, 86.0, 80.0, 72.0, 81.0, 79.0, 92.0, 86.0, 90.0, 95.0, 91.0, 82.0, 94.0, 62.0, 81.0, 97.0, 81.0, 100.0, 86.0]
  out "HSRL molecular Smoothed":dbl[](array[numeric])=[78.46596100278555, 68.14005571030643, 72.21108635097495, 83.59827298050143, 105.12612813370474, 125.53420612813368, 149.33086350974924, 177.23894150417823, 206.57598885793874, 236.7319777158774, 265.3475766016713, 293.978495821727, 320.6762674094707, 345.6330919220055, 370.6303064066852, 392.4144289693593, 411.0899164345402, 428.6929805013925, 439.8057938718661, 447.37682451253454, 456.7849025069634, 461.61916434540353, 461.58852367687984, 455.98963788300796, 448.4325348189412, 443.3754317548744, 434.7960445682449, 420.23754874651786, 405.5523119777157, 392.6511977715877, 378.5230640668523, 367.26122562674084, 354.22779944289687, 337.4840668523676, 322.4589972144846, 305.99103064066844, 293.2737604456824, 282.7236211699163, 267.93532033426175, 254.76679665738158, 243.93532033426175, 234.15816155988847, 226.48545961002782, 215.28908077994424, 203.44506963788297, 194.70272980501392, 185.77097493036212, 177.0021727019498, 168.97013927576592, 166.00774373259043, 160.57320334261829, 151.0829526462395, 147.1720891364902, 155.58852367688016, 192.09688022284118, 289.0467409470752, 459.51610027855133, 603.4576044568242, 593.0592757660164, 463.82250696378804, 324.29743732590515, 228.1233426183843, 170.14284122562668, 130.47571030640668, 114.35454038997219, 115.76540389972146, 121.30440111420614, 121.80857938718667, 117.01749303621173, 106.97013927576603, 96.46456824512538, 87.49938718662958, 79.13169916434543, 73.25286908077996, 64.88378830083568, 56.12334261838441, 49.80300835654596, 42.01192200557104, 37.28350974930362, 33.74729805013928, 28.73058495821728, 29.472924791086356, 27.439498607242346, 26.48128133704736, 26.453426183844016, 25.649805013927587, 25.40328690807801, 23.46874651810586, 27.059275766016732, 42.58713091922009, 103.71108635097495, 248.80161559888575, 461.3698607242338, 644.4186072423395, 702.5439554317545, 646.2528690807795, 552.2459052924787, 478.4102506963784, 446.46178272980455, 439.5453481894146, 435.98963788300796, 408.8712534818939, 342.1985515320334, 257.24311977715877, 173.15676880222838, 105.39075208913647, 57.76122562674095, 29.06763231197772, 13.050919220055716, 7.009136490250704, 6.075988857938726, 1.34061281337048, 0.31554317548747146, 4.5035654596100345, 5.063454038997222, 2.511922005571037, 2.1191643454039064, 2.0244568245125416, 1.7403342618384467, 2.936713091922012, 1.2417270194986136, -1.3850139275765954, 1.0355988857938785, 2.5355988857938785, 2.5355988857938794, 0.24033426183844742, -1.5061838440111353, 0.006350974930369013, 1.4562116991643521, 2.3461838440111498, 1.7751532033426258, -0.12456824512534104, -0.7332033426183768, -0.6914206128133635, -0.605069637883002, 0.7222284122562738, 0.9534261838440174, -1.0340389972144783, -2.7359888579387124, -2.361337047353754, -0.6955988857938656, 2.1888022284122632, 1.5996657381615669, 0.29325905292479737, 2.009136490250704, 3.004958217270203, 0.9200000000000066, -0.06746518105848953, 2.195766016713099, -0.5646796657381548, -1.3111977715877372, 0.5634540389972211, 1.5342061281337116, 0.0453481894150487, 0.2876880222841294, 2.8615041782729875, 1.4436768802228475, 2.7807242339832943, 4.174874651810592, 2.1915877437325966, 1.8155431754874714, 1.7013370473537677, 2.411643454039005, 2.946462395543182, 1.9757103064066914, 1.138662952646246, 0.06206128133705363, -0.06607242339832242, -1.0772144846796596, -1.4198328690807738, -3.3223398328690745, -2.9783286908077935, -3.447688022284117, -1.901727019498601, 2.8893593314763297, 1.8085793871866358, -0.9072980501392696, -0.8752646239554256, 1.800222841225633, 3.0258495821727083, 0.35732590529248554, -1.2373816155988793, -1.2387743732590466, 1.1303064066852442, 2.634484679665746, 1.1553760445682517, 1.68044568245126, 0.4840668523676943, 0.7194428969359394, 2.089916434540397, 0.18880222841226346, 1.0077437325905363, 1.4757103064066928, 0.35454038997215204, -0.4713649025069573, -0.5437883008356478, 0.38378830083566146, -1.1022841225626678, 0.01331476323120484, 0.7723676880222912, -2.666350974930355, -3.035431754874645, 0.42139275766017326, 0.7319777158774434, -2.1705292479108573, -0.7053481894150346, 1.1581615598885866, 1.4074651810585024, 0.13866295264624595, -1.3557660167130854, -1.0382172701949794, 0.27793871866295894, 2.1177715877437397, 0.3350417827298129, 0.16373259052925482, -1.1914206128133635, 0.5063509749303694, 3.1525905292479175, 1.2667966573816218, -0.4588300835654533, -2.4713649025069575, -0.4267966573816093, 0.8044011142061347, -0.8223398328690735, 0.3712534818941574, 1.0718105849582236, 0.736155988857945, 0.7667966573816218, 1.018885793871873, 0.42557103064067525, -2.502005571030634, -1.781949860724227, 1.4158217270195053, -0.31119777158773765, -1.6259610027855091, -0.006183844011135781, -1.0047910863509686, -0.837660167130913, 0.9408913649025132, -0.0702506963788232, -2.5047910863509677, -0.5382172701949788, 3.0634540389972216, 2.37961002785516, 1.1219498607242417, -0.06607242339832148, -0.3864066852367626, 1.15119777158775, 1.683231197771594, 1.1985515320334326, 3.1038440111420678, 3.19019498607243, 1.8851810584958286, 2.683231197771595, 1.9172144846796726, -0.1329247910863447, 1.6177715877437393, 2.752869080779951, -0.42958217270194365, 1.3336490250696444, 1.541169916434547, -0.47832869080779306, -0.5967130919219993, -0.6705292479108562, -1.4936490250696297, -3.013147632311971, -2.5396100278551472, -3.1524233983286845, -0.8028412256267345, 2.268189415041789, -0.3627298050139214, -2.3891922005570967, 1.314150417827304, 2.0843454038997278, 0.40885793871866927, 1.5049582172702012, -0.11342618384400482]
  out "On-Line Bin Readings 2":dbl[](array[numeric])=[236.0, 223.0, 194.0, 231.0, 273.0, 260.0, 270.0, 320.0, 326.0, 336.0, 403.0, 441.0, 422.0, 441.0, 475.0, 485.0, 513.0, 546.0, 536.0, 507.0, 605.0, 555.0, 555.0, 572.0, 572.0, 570.0, 504.0, 562.0, 515.0, 508.0, 483.0, 464.0, 449.0, 459.0, 481.0, 410.0, 433.0, 395.0, 414.0, 408.0, 404.0, 398.0, 349.0, 368.0, 315.0, 355.0, 356.0, 311.0, 324.0, 340.0, 310.0, 265.0, 314.0, 284.0, 295.0, 285.0, 283.0, 303.0, 300.0, 242.0, 269.0, 318.0, 312.0, 417.0, 345.0, 378.0, 324.0, 276.0, 258.0, 250.0, 219.0, 198.0, 179.0, 220.0, 274.0, 278.0, 219.0, 225.0, 191.0, 160.0, 195.0, 163.0, 159.0, 157.0, 170.0, 187.0, 164.0, 171.0, 184.0, 168.0, 164.0, 171.0, 180.0, 186.0, 196.0, 173.0, 196.0, 155.0, 179.0, 154.0, 166.0, 190.0, 178.0, 145.0, 177.0, 186.0, 177.0, 168.0, 168.0, 168.0, 165.0, 146.0, 164.0, 170.0, 162.0, 150.0, 150.0, 185.0, 173.0, 164.0, 183.0, 179.0, 165.0, 175.0, 181.0, 168.0, 162.0, 173.0, 156.0, 155.0, 172.0, 160.0, 159.0, 175.0, 142.0, 181.0, 171.0, 182.0, 177.0, 162.0, 177.0, 169.0, 170.0, 190.0, 155.0, 160.0, 158.0, 167.0, 174.0, 173.0, 172.0, 168.0, 155.0, 151.0, 170.0, 169.0, 176.0, 180.0, 170.0, 180.0, 158.0, 153.0, 190.0, 180.0, 167.0, 170.0, 151.0, 161.0, 164.0, 163.0, 166.0, 155.0, 163.0, 186.0, 163.0, 172.0, 170.0, 180.0, 173.0, 155.0, 155.0, 164.0, 179.0, 178.0, 161.0, 149.0, 169.0, 159.0, 146.0, 143.0, 185.0, 166.0, 186.0, 165.0, 176.0, 146.0, 178.0, 161.0, 189.0, 168.0, 152.0, 158.0, 166.0, 189.0, 157.0, 160.0, 170.0, 159.0, 157.0, 178.0, 159.0, 154.0, 172.0, 162.0, 165.0, 161.0, 154.0, 168.0, 175.0, 181.0, 169.0, 162.0, 156.0, 180.0, 161.0, 169.0, 178.0, 150.0, 165.0, 157.0, 161.0, 159.0, 155.0, 157.0, 172.0, 171.0, 158.0, 189.0, 176.0, 184.0, 186.0, 181.0, 174.0, 158.0, 164.0, 166.0, 160.0, 163.0, 162.0, 160.0, 190.0, 180.0, 187.0, 177.0, 176.0, 183.0, 134.0, 187.0, 185.0, 174.0, 146.0, 166.0, 164.0, 165.0, 154.0, 181.0, 168.0, 188.0, 155.0, 185.0, 156.0, 185.0, 145.0, 170.0, 156.0, 177.0, 168.0, 173.0, 148.0]
  in  "stop":bool
  in  "Reset Average":bool=TRUE
  in  "Save Data?":bool=TRUE
  in  "Collect Data?":bool=TRUE
  in  "ILX Address":i32=6 min=0 step=1
  in  "Lambda On DBR Current":dbl=171.13999999999868
  in  "Lambda Off DBR Current":dbl=172.9499999999997
  in  "Tab Control":T2(tab)=enum."NRB"
  out "Water Vapor Number Density  2":cluster{"Y":dbl[], "Y":dbl[]}[](graph)=[{"Y"=[nan, nan, nan, nan, nan, nan, nan, nan, nan, nan, nan, nan, nan, nan, nan, nan, nan, nan, nan, nan, nan, nan, nan, nan, nan, nan, nan, nan, nan, nan, nan, nan, nan, nan, nan, nan, nan, nan, nan, nan, nan, nan, nan, nan, nan, nan, nan, nan, nan, nan, nan, nan, nan, nan, nan, nan, nan, nan, nan, nan, nan, nan, nan, nan, nan, nan, nan, nan, nan, nan, nan, nan, nan, nan, nan, nan, nan, nan, nan, nan, nan, nan, nan, nan, nan, nan, nan, nan, nan, nan, nan, nan, nan, nan, nan, nan, nan, nan, nan, nan, nan, nan, nan, nan, nan, nan, nan, nan, nan, nan, nan, nan, nan, nan, nan, nan, nan, nan, nan, nan, nan, nan, nan, nan, nan, nan, nan, nan, nan, nan, nan, nan, nan, nan, nan, nan, nan, nan, nan, nan, nan, nan, nan, nan, nan, nan, nan, nan, nan, nan, nan, nan, nan, nan, nan, nan, nan, nan, nan, nan, nan, nan, nan, nan, nan, nan, nan, nan, nan, nan, nan, nan, nan, nan, nan, nan, nan, nan, nan, nan, nan, nan, nan, nan, nan, nan, nan, nan, nan, nan, nan, nan, nan, nan, nan, nan, nan, nan, nan, nan, nan, nan, nan, nan, nan, nan, nan, nan, nan, nan, nan, nan, nan, nan, nan, nan, nan, nan, nan, nan, nan, nan, nan, nan, nan, nan, nan, nan, nan, nan, nan, nan, nan, nan, nan, nan, nan, nan, nan, nan, nan, nan, nan, nan, nan, nan, nan, nan, nan, nan, nan, nan, nan, nan, nan, nan, nan, nan, nan, nan, nan, nan, nan, nan, nan, nan, nan, nan, nan, nan, nan, nan, nan, nan, nan, nan], "Y"=[0.075, 0.15, 0.22499999999999998, 0.3, 0.375, 0.45, 0.5249999999999999, 0.6, 0.6749999999999999, 0.7499999999999999, 0.825, 0.8999999999999999, 0.9749999999999999, 1.05, 1.125, 1.2, 1.275, 1.3499999999999999, 1.4249999999999998, 1.5, 1.575, 1.65, 1.7249999999999999, 1.7999999999999998, 1.8749999999999998, 1.95, 2.025, 2.1, 2.1750000000000003, 2.25, 2.325, 2.4, 2.475, 2.5500000000000003, 2.625, 2.7, 2.775, 2.85, 2.9250000000000003, 3.0, 3.075, 3.15, 3.225, 3.3000000000000003, 3.375, 3.45, 3.525, 3.6, 3.675, 3.75, 3.825, 3.9, 3.975, 4.05, 4.125, 4.2, 4.275, 4.35, 4.425, 4.5, 4.575, 4.65, 4.725, 4.8, 4.875, 4.95, 5.025, 5.1, 5.175, 5.25, 5.325, 5.4, 5.475, 5.55, 5.625, 5.7, 5.775, 5.85, 5.925, 6.0, 6.075, 6.15, 6.225, 6.3, 6.375, 6.45, 6.525, 6.6, 6.675, 6.75, 6.825, 6.9, 6.975, 7.05, 7.125, 7.2, 7.2749999999999995, 7.35, 7.425, 7.5, 7.575, 7.6499999999999995, 7.725, 7.8, 7.875, 7.95, 8.024999999999999, 8.1, 8.174999999999999, 8.249999999999998, 8.325, 8.399999999999999, 8.475, 8.549999999999999, 8.624999999999998, 8.7, 8.774999999999999, 8.85, 8.924999999999999, 8.999999999999998, 9.075, 9.149999999999999, 9.225, 9.299999999999999, 9.374999999999998, 9.45, 9.524999999999999, 9.6, 9.674999999999999, 9.749999999999998, 9.825, 9.899999999999999, 9.975, 10.049999999999999, 10.124999999999998, 10.2, 10.274999999999999, 10.35, 10.424999999999999, 10.499999999999998, 10.575, 10.649999999999999, 10.725, 10.799999999999999, 10.874999999999998, 10.95, 11.024999999999999, 11.1, 11.174999999999999, 11.249999999999998, 11.325, 11.399999999999999, 11.475, 11.549999999999999, 11.624999999999998, 11.7, 11.774999999999999, 11.85, 11.924999999999999, 11.999999999999998, 12.075, 12.149999999999999, 12.225, 12.299999999999999, 12.374999999999998, 12.45, 12.524999999999999, 12.6, 12.674999999999999, 12.749999999999998, 12.825, 12.899999999999999, 12.975, 13.049999999999999, 13.124999999999998, 13.2, 13.274999999999999, 13.35, 13.424999999999999, 13.499999999999998, 13.575, 13.649999999999999, 13.725, 13.799999999999999, 13.874999999999998, 13.95, 14.024999999999999, 14.1, 14.174999999999999, 14.249999999999998, 14.325, 14.399999999999999, 14.474999999999998, 14.549999999999999, 14.624999999999998, 14.7, 14.774999999999999, 14.849999999999998, 14.924999999999999, 14.999999999999998, 15.075, 15.149999999999999, 15.224999999999998, 15.299999999999999, 15.374999999999998, 15.45, 15.524999999999999, 15.599999999999998, 15.674999999999999, 15.749999999999998, 15.825, 15.899999999999999, 15.974999999999998, 16.05, 16.125, 16.2, 16.275, 16.349999999999998, 16.424999999999997, 16.5, 16.575, 16.65, 16.724999999999998, 16.799999999999997, 16.875, 16.95, 17.025, 17.099999999999998, 17.174999999999997, 17.25, 17.325, 17.4, 17.474999999999998, 17.549999999999997, 17.625, 17.7, 17.775, 17.849999999999998, 17.924999999999997, 18.0, 18.075, 18.15, 18.224999999999998, 18.299999999999997, 18.375, 18.45, 18.525, 18.599999999999998, 18.674999999999997, 18.75, 18.825, 18.9, 18.974999999999998, 19.049999999999997, 19.125, 19.2, 19.275, 19.349999999999998, 19.424999999999997, 19.5, 19.575, 19.65, 19.724999999999998, 19.799999999999997, 19.875, 19.95, 20.025, 20.099999999999998, 20.174999999999997, 20.25, 20.325, 20.4, 20.474999999999998, 20.549999999999997, 20.625, 20.7, 20.775, 20.849999999999998, 20.924999999999997, 21.0]}, ...(2 in all)]
  out "Absolute Humidity":cluster{"Y":dbl[], "Y":dbl[]}[](graph)=[{"Y"=[nan, nan, nan, nan, nan, nan, nan, nan, nan, nan, nan, nan, nan, nan, nan, nan, nan, nan, nan, nan, nan, nan, nan, nan, nan, nan, nan, nan, nan, nan, nan, nan, nan, nan, nan, nan, nan, nan, nan, nan, nan, nan, nan, nan, nan, nan, nan, nan, nan, nan, nan, nan, nan, nan, nan, nan, nan, nan, nan, nan, nan, nan, nan, nan, nan, nan, nan, nan, nan, nan, nan, nan, nan, nan, nan, nan, nan, nan, nan, nan, nan, nan, nan, nan, nan, nan, nan, nan, nan, nan, nan, nan, nan, nan, nan, nan, nan, nan, nan, nan, nan, nan, nan, nan, nan, nan, nan, nan, nan, nan, nan, nan, nan, nan, nan, nan, nan, nan, nan, nan, nan, nan, nan, nan, nan, nan, nan, nan, nan, nan, nan, nan, nan, nan, nan, nan, nan, nan, nan, nan, nan, nan, nan, nan, nan, nan, nan, nan, nan, nan, nan, nan, nan, nan, nan, nan, nan, nan, nan, nan, nan, nan, nan, nan, nan, nan, nan, nan, nan, nan, nan, nan, nan, nan, nan, nan, nan, nan, nan, nan, nan, nan, nan, nan, nan, nan, nan, nan, nan, nan, nan, nan, nan, nan, nan, nan, nan, nan, nan, nan, nan, nan, nan, nan, nan, nan, nan, nan, nan, nan, nan, nan, nan, nan, nan, nan, nan, nan, nan, nan, nan, nan, nan, nan, nan, nan, nan, nan, nan, nan, nan, nan, nan, nan, nan, nan, nan, nan, nan, nan, nan, nan, nan, nan, nan, nan, nan, nan, nan, nan, nan, nan, nan, nan, nan, nan, nan, nan, nan, nan, nan, nan, nan, nan, nan, nan, nan, nan, nan, nan, nan, nan, nan, nan, nan, nan], "Y"=[0.075, 0.15, 0.22499999999999998, 0.3, 0.375, 0.45, 0.5249999999999999, 0.6, 0.6749999999999999, 0.7499999999999999, 0.825, 0.8999999999999999, 0.9749999999999999, 1.05, 1.125, 1.2, 1.275, 1.3499999999999999, 1.4249999999999998, 1.5, 1.575, 1.65, 1.7249999999999999, 1.7999999999999998, 1.8749999999999998, 1.95, 2.025, 2.1, 2.1750000000000003, 2.25, 2.325, 2.4, 2.475, 2.5500000000000003, 2.625, 2.7, 2.775, 2.85, 2.9250000000000003, 3.0, 3.075, 3.15, 3.225, 3.3000000000000003, 3.375, 3.45, 3.525, 3.6, 3.675, 3.75, 3.825, 3.9, 3.975, 4.05, 4.125, 4.2, 4.275, 4.35, 4.425, 4.5, 4.575, 4.65, 4.725, 4.8, 4.875, 4.95, 5.025, 5.1, 5.175, 5.25, 5.325, 5.4, 5.475, 5.55, 5.625, 5.7, 5.775, 5.85, 5.925, 6.0, 6.075, 6.15, 6.225, 6.3, 6.375, 6.45, 6.525, 6.6, 6.675, 6.75, 6.825, 6.9, 6.975, 7.05, 7.125, 7.2, 7.2749999999999995, 7.35, 7.425, 7.5, 7.575, 7.6499999999999995, 7.725, 7.8, 7.875, 7.95, 8.024999999999999, 8.1, 8.174999999999999, 8.249999999999998, 8.325, 8.399999999999999, 8.475, 8.549999999999999, 8.624999999999998, 8.7, 8.774999999999999, 8.85, 8.924999999999999, 8.999999999999998, 9.075, 9.149999999999999, 9.225, 9.299999999999999, 9.374999999999998, 9.45, 9.524999999999999, 9.6, 9.674999999999999, 9.749999999999998, 9.825, 9.899999999999999, 9.975, 10.049999999999999, 10.124999999999998, 10.2, 10.274999999999999, 10.35, 10.424999999999999, 10.499999999999998, 10.575, 10.649999999999999, 10.725, 10.799999999999999, 10.874999999999998, 10.95, 11.024999999999999, 11.1, 11.174999999999999, 11.249999999999998, 11.325, 11.399999999999999, 11.475, 11.549999999999999, 11.624999999999998, 11.7, 11.774999999999999, 11.85, 11.924999999999999, 11.999999999999998, 12.075, 12.149999999999999, 12.225, 12.299999999999999, 12.374999999999998, 12.45, 12.524999999999999, 12.6, 12.674999999999999, 12.749999999999998, 12.825, 12.899999999999999, 12.975, 13.049999999999999, 13.124999999999998, 13.2, 13.274999999999999, 13.35, 13.424999999999999, 13.499999999999998, 13.575, 13.649999999999999, 13.725, 13.799999999999999, 13.874999999999998, 13.95, 14.024999999999999, 14.1, 14.174999999999999, 14.249999999999998, 14.325, 14.399999999999999, 14.474999999999998, 14.549999999999999, 14.624999999999998, 14.7, 14.774999999999999, 14.849999999999998, 14.924999999999999, 14.999999999999998, 15.075, 15.149999999999999, 15.224999999999998, 15.299999999999999, 15.374999999999998, 15.45, 15.524999999999999, 15.599999999999998, 15.674999999999999, 15.749999999999998, 15.825, 15.899999999999999, 15.974999999999998, 16.05, 16.125, 16.2, 16.275, 16.349999999999998, 16.424999999999997, 16.5, 16.575, 16.65, 16.724999999999998, 16.799999999999997, 16.875, 16.95, 17.025, 17.099999999999998, 17.174999999999997, 17.25, 17.325, 17.4, 17.474999999999998, 17.549999999999997, 17.625, 17.7, 17.775, 17.849999999999998, 17.924999999999997, 18.0, 18.075, 18.15, 18.224999999999998, 18.299999999999997, 18.375, 18.45, 18.525, 18.599999999999998, 18.674999999999997, 18.75, 18.825, 18.9, 18.974999999999998, 19.049999999999997, 19.125, 19.2, 19.275, 19.349999999999998, 19.424999999999997, 19.5, 19.575, 19.65, 19.724999999999998, 19.799999999999997, 19.875, 19.95, 20.025, 20.099999999999998, 20.174999999999997, 20.25, 20.325, 20.4, 20.474999999999998, 20.549999999999997, 20.625, 20.7, 20.775, 20.849999999999998, 20.924999999999997, 21.0]}, ...(2 in all)]
  out "NRB plot":cluster{"Y":dbl[], "Y":dbl[]}[](graph)=[{"Y"=[0.0, 0.0, 0.0, 0.0, 0.0, 0.0, 0.0, 0.0, 0.0, 0.0, 0.0, 0.0, 0.0, 0.0, 0.0, 0.0, 0.0, 0.0, 0.0, 0.0, 0.0, 0.0, 0.0, 0.0, 0.0, 0.0, 0.0, 0.0, 0.0, 0.0, 0.0, 0.0, 0.0, 0.0, 0.0, 0.0, 0.0, 0.0, 0.0, 0.0, 0.0, 0.0, 0.0, 0.0, 0.0, 0.0, 0.0, 0.0, 0.0, 0.0, 0.0, 0.0, 0.0, 0.0, 0.0, 0.0, 0.0, 0.0, 0.0, 0.0, 0.0, 0.0, 0.0, 0.0, 0.0, 0.0, 0.0, 0.0, 0.0, 0.0, 0.0, 0.0, 0.0, 0.0, 0.0, 0.0, 0.0, 0.0, 0.0, 0.0, 0.0, 0.0, 0.0, 0.0, 0.0, 0.0, 0.0, 0.0, 0.0, 0.0, 0.0, 0.0, 0.0, 0.0, 0.0, 0.0, 0.0, 0.0, 0.0, 0.0, 0.0, 0.0, 0.0, 0.0, 0.0, 0.0, 0.0, 0.0, 0.0, 0.0, 0.0, 0.0, 0.0, 0.0, 0.0, 0.0, 0.0, 0.0, 0.0, 0.0, 0.0, 0.0, 0.0, 0.0, 0.0, 0.0, 0.0, 0.0, 0.0, 0.0, 0.0, 0.0, 0.0, 0.0, 0.0, 0.0, 0.0, 0.0, 0.0, 0.0, 0.0, 0.0, 0.0, 0.0, 0.0, 0.0, 0.0, 0.0, 0.0, 0.0, 0.0, 0.0, 0.0, 0.0, 0.0, 0.0, 0.0, 0.0, 0.0, 0.0, 0.0, 0.0, 0.0, 0.0, 0.0, 0.0, 0.0, 0.0, 0.0, 0.0, 0.0, 0.0, 0.0, 0.0, 0.0, 0.0, 0.0, 0.0, 0.0, 0.0, 0.0, 0.0, 0.0, 0.0, 0.0, 0.0, 0.0, 0.0, 0.0, 0.0, 0.0, 0.0, 0.0, 0.0, 0.0, 0.0, 0.0, 0.0, 0.0, 0.0, 0.0, 0.0, 0.0, 0.0, 0.0, 0.0, 0.0, 0.0, 0.0, 0.0, 0.0, 0.0, 0.0, 0.0, 0.0, 0.0, 0.0, 0.0, 0.0, 0.0, 0.0, 0.0, 0.0, 0.0, 0.0, 0.0, 0.0, 0.0, 0.0, 0.0, 0.0, 0.0, 0.0, 0.0, 0.0, 0.0, 0.0, 0.0, 0.0, 0.0, 0.0, 0.0, 0.0, 0.0, 0.0, 0.0, 0.0, 0.0, 0.0, 0.0, 0.0, 0.0, 0.0, 0.0, 0.0, 0.0, 0.0, 0.0, 0.0, 0.0, 0.0, 0.0, 0.0, 0.0, 0.0, 0.0, 0.0, 0.0, 0.0, 0.0, 0.0, 0.0, 0.0, 0.0, 0.0, 0.0, 0.0], "Y"=[0.075, 0.15, 0.22499999999999998, 0.3, 0.375, 0.45, 0.5249999999999999, 0.6, 0.6749999999999999, 0.7499999999999999, 0.825, 0.8999999999999999, 0.9749999999999999, 1.05, 1.125, 1.2, 1.275, 1.3499999999999999, 1.4249999999999998, 1.5, 1.575, 1.65, 1.7249999999999999, 1.7999999999999998, 1.8749999999999998, 1.95, 2.025, 2.1, 2.1750000000000003, 2.25, 2.325, 2.4, 2.475, 2.5500000000000003, 2.625, 2.7, 2.775, 2.85, 2.9250000000000003, 3.0, 3.075, 3.15, 3.225, 3.3000000000000003, 3.375, 3.45, 3.525, 3.6, 3.675, 3.75, 3.825, 3.9, 3.975, 4.05, 4.125, 4.2, 4.275, 4.35, 4.425, 4.5, 4.575, 4.65, 4.725, 4.8, 4.875, 4.95, 5.025, 5.1, 5.175, 5.25, 5.325, 5.4, 5.475, 5.55, 5.625, 5.7, 5.775, 5.85, 5.925, 6.0, 6.075, 6.15, 6.225, 6.3, 6.375, 6.45, 6.525, 6.6, 6.675, 6.75, 6.825, 6.9, 6.975, 7.05, 7.125, 7.2, 7.2749999999999995, 7.35, 7.425, 7.5, 7.575, 7.6499999999999995, 7.725, 7.8, 7.875, 7.95, 8.024999999999999, 8.1, 8.174999999999999, 8.249999999999998, 8.325, 8.399999999999999, 8.475, 8.549999999999999, 8.624999999999998, 8.7, 8.774999999999999, 8.85, 8.924999999999999, 8.999999999999998, 9.075, 9.149999999999999, 9.225, 9.299999999999999, 9.374999999999998, 9.45, 9.524999999999999, 9.6, 9.674999999999999, 9.749999999999998, 9.825, 9.899999999999999, 9.975, 10.049999999999999, 10.124999999999998, 10.2, 10.274999999999999, 10.35, 10.424999999999999, 10.499999999999998, 10.575, 10.649999999999999, 10.725, 10.799999999999999, 10.874999999999998, 10.95, 11.024999999999999, 11.1, 11.174999999999999, 11.249999999999998, 11.325, 11.399999999999999, 11.475, 11.549999999999999, 11.624999999999998, 11.7, 11.774999999999999, 11.85, 11.924999999999999, 11.999999999999998, 12.075, 12.149999999999999, 12.225, 12.299999999999999, 12.374999999999998, 12.45, 12.524999999999999, 12.6, 12.674999999999999, 12.749999999999998, 12.825, 12.899999999999999, 12.975, 13.049999999999999, 13.124999999999998, 13.2, 13.274999999999999, 13.35, 13.424999999999999, 13.499999999999998, 13.575, 13.649999999999999, 13.725, 13.799999999999999, 13.874999999999998, 13.95, 14.024999999999999, 14.1, 14.174999999999999, 14.249999999999998, 14.325, 14.399999999999999, 14.474999999999998, 14.549999999999999, 14.624999999999998, 14.7, 14.774999999999999, 14.849999999999998, 14.924999999999999, 14.999999999999998, 15.075, 15.149999999999999, 15.224999999999998, 15.299999999999999, 15.374999999999998, 15.45, 15.524999999999999, 15.599999999999998, 15.674999999999999, 15.749999999999998, 15.825, 15.899999999999999, 15.974999999999998, 16.05, 16.125, 16.2, 16.275, 16.349999999999998, 16.424999999999997, 16.5, 16.575, 16.65, 16.724999999999998, 16.799999999999997, 16.875, 16.95, 17.025, 17.099999999999998, 17.174999999999997, 17.25, 17.325, 17.4, 17.474999999999998, 17.549999999999997, 17.625, 17.7, 17.775, 17.849999999999998, 17.924999999999997, 18.0, 18.075, 18.15, 18.224999999999998, 18.299999999999997, 18.375, 18.45, 18.525, 18.599999999999998, 18.674999999999997, 18.75, 18.825, 18.9, 18.974999999999998, 19.049999999999997, 19.125, 19.2, 19.275, 19.349999999999998, 19.424999999999997, 19.5, 19.575, 19.65, 19.724999999999998, 19.799999999999997, 19.875, 19.95, 20.025, 20.099999999999998, 20.174999999999997, 20.25, 20.325, 20.4, 20.474999999999998, 20.549999999999997, 20.625, 20.7, 20.775, 20.849999999999998, 20.924999999999997, 21.0]}, ...(2 in all)]
  in  "background length":i32=25
  out "Correction":cluster{"Y":dbl[], "Y":dbl[]}[](graph)=[{"Y"=[1.0, 1.0, 1.0, 1.0, 1.0, 1.0, 1.0, 1.0, 1.0, 1.0, 1.0, 1.0, 1.0, 1.0, 1.0, 1.0, 1.0, 1.0, 1.0, 1.0, 1.0, 1.0, 1.0, 1.0, 1.0, 1.0, 1.0, 1.0, 1.0, 1.0, 1.0, 1.0, 1.0, 1.0, 1.0, 1.0, 1.0, 1.0, 1.0, 1.0, 1.0, 1.0, 1.0, 1.0, 1.0, 1.0, 1.0, 1.0, 1.0, 1.0, 1.0, 1.0, 1.0, 1.0, 1.0, 1.0, 1.0, 1.0, 1.0, 1.0, 1.0, 1.0, 1.0, 1.0, 1.0, 1.0, 1.0, 1.0, 1.0, 1.0, 1.0, 1.0, 1.0, 1.0, 1.0, 1.0, 1.0, 1.0, 1.0, 1.0, 1.0, 1.0, 1.0, 1.0, 1.0, 1.0, 1.0, 1.0, 1.0, 1.0, 1.0, 1.0, 1.0, 1.0, 1.0, 1.0, 1.0, 1.0, 1.0, 1.0, 1.0, 1.0, 1.0, 1.0, 1.0, 1.0, 1.0, 1.0, 1.0, 1.0, 1.0, 1.0, 1.0, 1.0, 1.0, 1.0, 1.0, 1.0, 1.0, 1.0, 1.0, 1.0, 1.0, 1.0, 1.0, 1.0, 1.0, 1.0, 1.0, 1.0, 1.0, 1.0, 1.0, 1.0, 1.0, 1.0, 1.0, 1.0, 1.0, 1.0, 1.0, 1.0, 1.0, 1.0, 1.0, 1.0, 1.0, 1.0, 1.0, 1.0, 1.0, 1.0, 1.0, 1.0, 1.0, 1.0, 1.0, 1.0, 1.0, 1.0, 1.0, 1.0, 1.0, 1.0, 1.0, 1.0, 1.0, 1.0, 1.0, 1.0, 1.0, 1.0, 1.0, 1.0, 1.0, 1.0, 1.0, 1.0, 1.0, 1.0, 1.0, 1.0, 1.0, 1.0, 1.0, 1.0, 1.0, 1.0, 1.0, 1.0, 1.0, 1.0, 1.0, 1.0, 1.0, 1.0, 1.0, 1.0, 1.0, 1.0, 1.0, 1.0, 1.0, 1.0, 1.0, 1.0, 1.0, 1.0, 1.0, 1.0, 1.0, 1.0, 1.0, 1.0, 1.0, 1.0, 1.0, 1.0, 1.0, 1.0, 1.0, 1.0, 1.0, 1.0, 1.0, 1.0, 1.0, 1.0, 1.0, 1.0, 1.0, 1.0, 1.0, 1.0, 1.0, 1.0, 1.0, 1.0, 1.0, 1.0, 1.0, 1.0, 1.0, 1.0, 1.0, 1.0, 1.0, 1.0, 1.0, 1.0, 1.0, 1.0, 1.0, 1.0, 1.0, 1.0, 1.0, 1.0, 1.0, 1.0, 1.0, 1.0, 1.0, 1.0, 1.0, 1.0, 1.0, 1.0, 1.0, 1.0, 1.0, 1.0, 1.0, 1.0, 1.0, 1.0, 1.0], "Y"=[0.075, 0.15, 0.22499999999999998, 0.3, 0.375, 0.45, 0.5249999999999999, 0.6, 0.6749999999999999, 0.7499999999999999, 0.825, 0.8999999999999999, 0.9749999999999999, 1.05, 1.125, 1.2, 1.275, 1.3499999999999999, 1.4249999999999998, 1.5, 1.575, 1.65, 1.7249999999999999, 1.7999999999999998, 1.8749999999999998, 1.95, 2.025, 2.1, 2.1750000000000003, 2.25, 2.325, 2.4, 2.475, 2.5500000000000003, 2.625, 2.7, 2.775, 2.85, 2.9250000000000003, 3.0, 3.075, 3.15, 3.225, 3.3000000000000003, 3.375, 3.45, 3.525, 3.6, 3.675, 3.75, 3.825, 3.9, 3.975, 4.05, 4.125, 4.2, 4.275, 4.35, 4.425, 4.5, 4.575, 4.65, 4.725, 4.8, 4.875, 4.95, 5.025, 5.1, 5.175, 5.25, 5.325, 5.4, 5.475, 5.55, 5.625, 5.7, 5.775, 5.85, 5.925, 6.0, 6.075, 6.15, 6.225, 6.3, 6.375, 6.45, 6.525, 6.6, 6.675, 6.75, 6.825, 6.9, 6.975, 7.05, 7.125, 7.2, 7.2749999999999995, 7.35, 7.425, 7.5, 7.575, 7.6499999999999995, 7.725, 7.8, 7.875, 7.95, 8.024999999999999, 8.1, 8.174999999999999, 8.249999999999998, 8.325, 8.399999999999999, 8.475, 8.549999999999999, 8.624999999999998, 8.7, 8.774999999999999, 8.85, 8.924999999999999, 8.999999999999998, 9.075, 9.149999999999999, 9.225, 9.299999999999999, 9.374999999999998, 9.45, 9.524999999999999, 9.6, 9.674999999999999, 9.749999999999998, 9.825, 9.899999999999999, 9.975, 10.049999999999999, 10.124999999999998, 10.2, 10.274999999999999, 10.35, 10.424999999999999, 10.499999999999998, 10.575, 10.649999999999999, 10.725, 10.799999999999999, 10.874999999999998, 10.95, 11.024999999999999, 11.1, 11.174999999999999, 11.249999999999998, 11.325, 11.399999999999999, 11.475, 11.549999999999999, 11.624999999999998, 11.7, 11.774999999999999, 11.85, 11.924999999999999, 11.999999999999998, 12.075, 12.149999999999999, 12.225, 12.299999999999999, 12.374999999999998, 12.45, 12.524999999999999, 12.6, 12.674999999999999, 12.749999999999998, 12.825, 12.899999999999999, 12.975, 13.049999999999999, 13.124999999999998, 13.2, 13.274999999999999, 13.35, 13.424999999999999, 13.499999999999998, 13.575, 13.649999999999999, 13.725, 13.799999999999999, 13.874999999999998, 13.95, 14.024999999999999, 14.1, 14.174999999999999, 14.249999999999998, 14.325, 14.399999999999999, 14.474999999999998, 14.549999999999999, 14.624999999999998, 14.7, 14.774999999999999, 14.849999999999998, 14.924999999999999, 14.999999999999998, 15.075, 15.149999999999999, 15.224999999999998, 15.299999999999999, 15.374999999999998, 15.45, 15.524999999999999, 15.599999999999998, 15.674999999999999, 15.749999999999998, 15.825, 15.899999999999999, 15.974999999999998, 16.05, 16.125, 16.2, 16.275, 16.349999999999998, 16.424999999999997, 16.5, 16.575, 16.65, 16.724999999999998, 16.799999999999997, 16.875, 16.95, 17.025, 17.099999999999998, 17.174999999999997, 17.25, 17.325, 17.4, 17.474999999999998, 17.549999999999997, 17.625, 17.7, 17.775, 17.849999999999998, 17.924999999999997, 18.0, 18.075, 18.15, 18.224999999999998, 18.299999999999997, 18.375, 18.45, 18.525, 18.599999999999998, 18.674999999999997, 18.75, 18.825, 18.9, 18.974999999999998, 19.049999999999997, 19.125, 19.2, 19.275, 19.349999999999998, 19.424999999999997, 19.5, 19.575, 19.65, 19.724999999999998, 19.799999999999997, 19.875, 19.95, 20.025, 20.099999999999998, 20.174999999999997, 20.25, 20.325, 20.4, 20.474999999999998, 20.549999999999997, 20.625, 20.7, 20.775, 20.849999999999998, 20.924999999999997, 21.0]}, ...(2 in all)]
  in  "dead time":dbl=3.7e-08
  out "Optical Depth":cluster{"Y":dbl[], "Y":dbl[]}[](graph)=[{"Y"=[nan, nan, nan, nan, nan, nan, nan, nan, nan, nan, nan, nan, nan, nan, nan, nan, nan, nan, nan, nan, nan, nan, nan, nan, nan, nan, nan, nan, nan, nan, nan, nan, nan, nan, nan, nan, nan, nan, nan, nan, nan, nan, nan, nan, nan, nan, nan, nan, nan, nan, nan, nan, nan, nan, nan, nan, nan, nan, nan, nan, nan, nan, nan, nan, nan, nan, nan, nan, nan, nan, nan, nan, nan, nan, nan, nan, nan, nan, nan, nan, nan, nan, nan, nan, nan, nan, nan, nan, nan, nan, nan, nan, nan, nan, nan, nan, nan, nan, nan, nan, nan, nan, nan, nan, nan, nan, nan, nan, nan, nan, nan, nan, nan, nan, nan, nan, nan, nan, nan, nan, nan, nan, nan, nan, nan, nan, nan, nan, nan, nan, nan, nan, nan, nan, nan, nan, nan, nan, nan, nan, nan, nan, nan, nan, nan, nan, nan, nan, nan, nan, nan, nan, nan, nan, nan, nan, nan, nan, nan, nan, nan, nan, nan, nan, nan, nan, nan, nan, nan, nan, nan, nan, nan, nan, nan, nan, nan, nan, nan, nan, nan, nan, nan, nan, nan, nan, nan, nan, nan, nan, nan, nan, nan, nan, nan, nan, nan, nan, nan, nan, nan, nan, nan, nan, nan, nan, nan, nan, nan, nan, nan, nan, nan, nan, nan, nan, nan, nan, nan, nan, nan, nan, nan, nan, nan, nan, nan, nan, nan, nan, nan, nan, nan, nan, nan, nan, nan, nan, nan, nan, nan, nan, nan, nan, nan, nan, nan, nan, nan, nan, nan, nan, nan, nan, nan, nan, nan, nan, nan, nan, nan, nan, nan, nan, nan, nan, nan, nan, nan, nan, nan, nan, nan, nan, nan, nan, nan], "Y"=[0.075, 0.15, 0.22499999999999998, 0.3, 0.375, 0.45, 0.5249999999999999, 0.6, 0.6749999999999999, 0.7499999999999999, 0.825, 0.8999999999999999, 0.9749999999999999, 1.05, 1.125, 1.2, 1.275, 1.3499999999999999, 1.4249999999999998, 1.5, 1.575, 1.65, 1.7249999999999999, 1.7999999999999998, 1.8749999999999998, 1.95, 2.025, 2.1, 2.1750000000000003, 2.25, 2.325, 2.4, 2.475, 2.5500000000000003, 2.625, 2.7, 2.775, 2.85, 2.9250000000000003, 3.0, 3.075, 3.15, 3.225, 3.3000000000000003, 3.375, 3.45, 3.525, 3.6, 3.675, 3.75, 3.825, 3.9, 3.975, 4.05, 4.125, 4.2, 4.275, 4.35, 4.425, 4.5, 4.575, 4.65, 4.725, 4.8, 4.875, 4.95, 5.025, 5.1, 5.175, 5.25, 5.325, 5.4, 5.475, 5.55, 5.625, 5.7, 5.775, 5.85, 5.925, 6.0, 6.075, 6.15, 6.225, 6.3, 6.375, 6.45, 6.525, 6.6, 6.675, 6.75, 6.825, 6.9, 6.975, 7.05, 7.125, 7.2, 7.2749999999999995, 7.35, 7.425, 7.5, 7.575, 7.6499999999999995, 7.725, 7.8, 7.875, 7.95, 8.024999999999999, 8.1, 8.174999999999999, 8.249999999999998, 8.325, 8.399999999999999, 8.475, 8.549999999999999, 8.624999999999998, 8.7, 8.774999999999999, 8.85, 8.924999999999999, 8.999999999999998, 9.075, 9.149999999999999, 9.225, 9.299999999999999, 9.374999999999998, 9.45, 9.524999999999999, 9.6, 9.674999999999999, 9.749999999999998, 9.825, 9.899999999999999, 9.975, 10.049999999999999, 10.124999999999998, 10.2, 10.274999999999999, 10.35, 10.424999999999999, 10.499999999999998, 10.575, 10.649999999999999, 10.725, 10.799999999999999, 10.874999999999998, 10.95, 11.024999999999999, 11.1, 11.174999999999999, 11.249999999999998, 11.325, 11.399999999999999, 11.475, 11.549999999999999, 11.624999999999998, 11.7, 11.774999999999999, 11.85, 11.924999999999999, 11.999999999999998, 12.075, 12.149999999999999, 12.225, 12.299999999999999, 12.374999999999998, 12.45, 12.524999999999999, 12.6, 12.674999999999999, 12.749999999999998, 12.825, 12.899999999999999, 12.975, 13.049999999999999, 13.124999999999998, 13.2, 13.274999999999999, 13.35, 13.424999999999999, 13.499999999999998, 13.575, 13.649999999999999, 13.725, 13.799999999999999, 13.874999999999998, 13.95, 14.024999999999999, 14.1, 14.174999999999999, 14.249999999999998, 14.325, 14.399999999999999, 14.474999999999998, 14.549999999999999, 14.624999999999998, 14.7, 14.774999999999999, 14.849999999999998, 14.924999999999999, 14.999999999999998, 15.075, 15.149999999999999, 15.224999999999998, 15.299999999999999, 15.374999999999998, 15.45, 15.524999999999999, 15.599999999999998, 15.674999999999999, 15.749999999999998, 15.825, 15.899999999999999, 15.974999999999998, 16.05, 16.125, 16.2, 16.275, 16.349999999999998, 16.424999999999997, 16.5, 16.575, 16.65, 16.724999999999998, 16.799999999999997, 16.875, 16.95, 17.025, 17.099999999999998, 17.174999999999997, 17.25, 17.325, 17.4, 17.474999999999998, 17.549999999999997, 17.625, 17.7, 17.775, 17.849999999999998, 17.924999999999997, 18.0, 18.075, 18.15, 18.224999999999998, 18.299999999999997, 18.375, 18.45, 18.525, 18.599999999999998, 18.674999999999997, 18.75, 18.825, 18.9, 18.974999999999998, 19.049999999999997, 19.125, 19.2, 19.275, 19.349999999999998, 19.424999999999997, 19.5, 19.575, 19.65, 19.724999999999998, 19.799999999999997, 19.875, 19.95, 20.025, 20.099999999999998, 20.174999999999997, 20.25, 20.325, 20.4, 20.474999999999998, 20.549999999999997, 20.625, 20.7, 20.775, 20.849999999999998, 20.924999999999997, 21.0]}] caption="XY Graph"
  out "RingBuffer offline far":dbl[][](array[numeric])
  out "RingBuffer aerosol far":dbl[][](array[numeric])
  in  "Weather":T3(tab)=enum."Pulse Energy (Micro Joule)"
  out "Temperature (C)":dbl(graph)=17.615079365079367
  out "Pressure (mb)":dbl(graph)=834.8901098901099
  out "Relative Humdity (%)":dbl(graph)=11.878815628815628
  out "Pulse Energy (Micro Joule)":T4(graph)={"Online Pulse Energy"=0.01106949857142857, "Pulse Energy Offline"=0.011023625714285713}
  out "?":cluster{"mean":dbl, "mean":dbl}(graph)={"mean"=0.0, "mean"=16816.0}
  out "Index":i32=1075
  out "Aerosol Smoothed":dbl[](array[numeric])
  out "Off-Line  Bin Readings":dbl[](array[numeric])
  out "Off-Line Smoothed":dbl[](array[numeric])
  out "On-Line  Smoothed":dbl[](array[numeric])
  out "On-Line Bin Readings":dbl[](array[numeric])
  out "Range Corrected Altitude Array":dbl[](array[numeric])=[5625.0, 22500.0, 50625.0, 90000.0, 140625.0, 202500.0, 275625.0, 360000.0, 455625.0, 562500.0, 680625.0, 810000.0, 950625.0, 1102500.0, 1265625.0, 1440000.0, 1625625.0, 1822500.0, 2030625.0, 2250000.0, 2480625.0, 2722500.0, 2975625.0, 3240000.0, 3515625.0, 3802500.0, 4100625.0, 4410000.0, 4730625.0, 5062500.0, 5405625.0, 5760000.0, 6125625.0, 6502500.0, 6890625.0, 7290000.0, 7700625.0, 8122500.0, 8555625.0, 9000000.0, 9455625.0, 9922500.0, 10400625.0, 10890000.0, 11390625.0, 11902500.0, 12425625.0, 12960000.0, 13505625.0, 14062500.0, 14630625.0, 15210000.0, 15800625.0, 16402500.0, 17015625.0, 17640000.0, 18275625.0, 18922500.0, 19580625.0, 20250000.0, 20930625.0, 21622500.0, 22325625.0, 23040000.0, 23765625.0, 24502500.0, 25250625.0, 26010000.0, 26780625.0, 27562500.0, 28355625.0, 29160000.0, 29975625.0, 30802500.0, 31640625.0, 32490000.0, 33350625.0, 34222500.0, 35105625.0, 36000000.0, 36905625.0, 37822500.0, 38750625.0, 39690000.0, 40640625.0, 41602500.0, 42575625.0, 43560000.0, 44555625.0, 45562500.0, 46580625.0, 47610000.0, 48650625.0, 49702500.0, 50765625.0, 51840000.0, 52925625.0, 54022500.0, 55130625.0, 56250000.0, 57380625.0, 58522500.0, 59675625.0, 60840000.0, 62015625.0, 63202500.0, 64400625.0, 65610000.0, 66830625.0, 68062500.0, 69305625.0, 70560000.0, 71825625.0, 73102500.0, 74390625.0, 75690000.0, 77000625.0, 78322500.0, 79655625.0, 81000000.0, 82355625.0, 83722500.0, 85100625.0, 86490000.0, 87890625.0, 89302500.0, 90725625.0, 92160000.0, 93605625.0, 95062500.0, 96530625.0, 98010000.0, 99500625.0, 101002500.0, 102515625.0, 104040000.0, 105575625.0, 107122500.0, 108680625.0, 110250000.0, 111830625.0, 113422500.0, 115025625.0, 116640000.0, 118265625.0, 119902500.0, 121550625.0, 123210000.0, 124880625.0, 126562500.0, 128255625.0, 129960000.0, 131675625.0, 133402500.0, 135140625.0, 136890000.0, 138650625.0, 140422500.0, 142205625.0, 144000000.0, 145805625.0, 147622500.0, 149450625.0, 151290000.0, 153140625.0, 155002500.0, 156875625.0, 158760000.0, 160655625.0, 162562500.0, 164480625.0, 166410000.0, 168350625.0, 170302500.0, 172265625.0, 174240000.0, 176225625.0, 178222500.0, 180230625.0, 182250000.0, 184280625.0, 186322500.0, 188375625.0, 190440000.0, 192515625.0, 194602500.0, 196700625.0, 198810000.0, 200930625.0, 203062500.0, 205205625.0, 207360000.0, 209525625.0, 211702500.0, 213890625.0, 216090000.0, 218300625.0, 220522500.0, 222755625.0, 225000000.0, 227255625.0, 229522500.0, 231800625.0, 234090000.0, 236390625.0, 238702500.0, 241025625.0, 243360000.0, 245705625.0, 248062500.0, 250430625.0, 252810000.0, 255200625.0, 257602500.0, 260015625.0, 262440000.0, 264875625.0, 267322500.0, 269780625.0, 272250000.0, 274730625.0, 277222500.0, 279725625.0, 282240000.0, 284765625.0, 287302500.0, 289850625.0, 292410000.0, 294980625.0, 297562500.0, 300155625.0, 302760000.0, 305375625.0, 308002500.0, 310640625.0, 313290000.0, 315950625.0, 318622500.0, 321305625.0, 324000000.0, 326705625.0, 329422500.0, 332150625.0, 334890000.0, 337640625.0, 340402500.0, 343175625.0, 345960000.0, 348755625.0, 351562500.0, 354380625.0, 357210000.0, 360050625.0, 362902500.0, 365765625.0, 368640000.0, 371525625.0, 374422500.0, 377330625.0, 380250000.0, 383180625.0, 386122500.0, 389075625.0, 392040000.0, 395015625.0, 398002500.0, 401000625.0, 404010000.0, 407030625.0, 410062500.0, 413105625.0, 416160000.0, 419225625.0, 422302500.0, 425390625.0, 428490000.0, 431600625.0, 434722500.0, 437855625.0, 441000000.0]
  out "Altitude Array (km)":dbl[](array[numeric])=[0.075, 0.15, 0.22499999999999998, 0.3, 0.375, 0.45, 0.5249999999999999, 0.6, 0.6749999999999999, 0.7499999999999999, 0.825, 0.8999999999999999, 0.9749999999999999, 1.05, 1.125, 1.2, 1.275, 1.3499999999999999, 1.4249999999999998, 1.5, 1.575, 1.65, 1.7249999999999999, 1.7999999999999998, 1.8749999999999998, 1.95, 2.025, 2.1, 2.1750000000000003, 2.25, 2.325, 2.4, 2.475, 2.5500000000000003, 2.625, 2.7, 2.775, 2.85, 2.9250000000000003, 3.0, 3.075, 3.15, 3.225, 3.3000000000000003, 3.375, 3.45, 3.525, 3.6, 3.675, 3.75, 3.825, 3.9, 3.975, 4.05, 4.125, 4.2, 4.275, 4.35, 4.425, 4.5, 4.575, 4.65, 4.725, 4.8, 4.875, 4.95, 5.025, 5.1, 5.175, 5.25, 5.325, 5.4, 5.475, 5.55, 5.625, 5.7, 5.775, 5.85, 5.925, 6.0, 6.075, 6.15, 6.225, 6.3, 6.375, 6.45, 6.525, 6.6, 6.675, 6.75, 6.825, 6.9, 6.975, 7.05, 7.125, 7.2, 7.2749999999999995, 7.35, 7.425, 7.5, 7.575, 7.6499999999999995, 7.725, 7.8, 7.875, 7.95, 8.024999999999999, 8.1, 8.174999999999999, 8.249999999999998, 8.325, 8.399999999999999, 8.475, 8.549999999999999, 8.624999999999998, 8.7, 8.774999999999999, 8.85, 8.924999999999999, 8.999999999999998, 9.075, 9.149999999999999, 9.225, 9.299999999999999, 9.374999999999998, 9.45, 9.524999999999999, 9.6, 9.674999999999999, 9.749999999999998, 9.825, 9.899999999999999, 9.975, 10.049999999999999, 10.124999999999998, 10.2, 10.274999999999999, 10.35, 10.424999999999999, 10.499999999999998, 10.575, 10.649999999999999, 10.725, 10.799999999999999, 10.874999999999998, 10.95, 11.024999999999999, 11.1, 11.174999999999999, 11.249999999999998, 11.325, 11.399999999999999, 11.475, 11.549999999999999, 11.624999999999998, 11.7, 11.774999999999999, 11.85, 11.924999999999999, 11.999999999999998, 12.075, 12.149999999999999, 12.225, 12.299999999999999, 12.374999999999998, 12.45, 12.524999999999999, 12.6, 12.674999999999999, 12.749999999999998, 12.825, 12.899999999999999, 12.975, 13.049999999999999, 13.124999999999998, 13.2, 13.274999999999999, 13.35, 13.424999999999999, 13.499999999999998, 13.575, 13.649999999999999, 13.725, 13.799999999999999, 13.874999999999998, 13.95, 14.024999999999999, 14.1, 14.174999999999999, 14.249999999999998, 14.325, 14.399999999999999, 14.474999999999998, 14.549999999999999, 14.624999999999998, 14.7, 14.774999999999999, 14.849999999999998, 14.924999999999999, 14.999999999999998, 15.075, 15.149999999999999, 15.224999999999998, 15.299999999999999, 15.374999999999998, 15.45, 15.524999999999999, 15.599999999999998, 15.674999999999999, 15.749999999999998, 15.825, 15.899999999999999, 15.974999999999998, 16.05, 16.125, 16.2, 16.275, 16.349999999999998, 16.424999999999997, 16.5, 16.575, 16.65, 16.724999999999998, 16.799999999999997, 16.875, 16.95, 17.025, 17.099999999999998, 17.174999999999997, 17.25, 17.325, 17.4, 17.474999999999998, 17.549999999999997, 17.625, 17.7, 17.775, 17.849999999999998, 17.924999999999997, 18.0, 18.075, 18.15, 18.224999999999998, 18.299999999999997, 18.375, 18.45, 18.525, 18.599999999999998, 18.674999999999997, 18.75, 18.825, 18.9, 18.974999999999998, 19.049999999999997, 19.125, 19.2, 19.275, 19.349999999999998, 19.424999999999997, 19.5, 19.575, 19.65, 19.724999999999998, 19.799999999999997, 19.875, 19.95, 20.025, 20.099999999999998, 20.174999999999997, 20.25, 20.325, 20.4, 20.474999999999998, 20.549999999999997, 20.625, 20.7, 20.775, 20.849999999999998, 20.924999999999997, 21.0]
  out "Offline Pulse Energy":dbl=0.011085018571428573
  out "Online Pulse Energy":dbl=0.01106949857142857
  in  "Instrument Control":T5(tab)=enum."Wavemeter"
  out "Readings":T6={"OnLineTEC"=14.1882877, "OnLineLD"=0.1605625, "OffLineTEC"=22.7611942, "OffLineLD"=0.00014843751, "EtalonTEC"=28.849308, "TSOA-TEC"=19.0036869, "Pro8000"=TRUE, "OnLine TEC"=TRUE, "OnLine LD"=TRUE, "OffLine TEC"=FALSE, "OffLine LD"=FALSE, "Etalon TEC"=TRUE, "TSOA TEC"=TRUE} {"OffLineLD" format="%.4g"; "OnLineLD" format="%.4g"; "TSOA-TEC" format="%.3g"; "EtalonTEC" format="%.3g"; "OffLineTEC" format="%.3g"; "OnLineTEC" format="%.3g"}
  in  "Settings":T7={"Module"=enum."On Line TEC", "OnLineTEC"=14.186249999999566, "OnLineLD"=0.16, "OffLineTEC"=29.780200000000985, "OffLineLD"=0.173, "EtalonTEC"=28.8, "TSOA-TEC"=19.0} {"OffLineLD" min=0.0 max=0.175 step=0.001 format="%.3p"; "OnLineLD" min=0.0 max=0.175 step=0.001 format="%.3p"; "TSOA-TEC" format="%.2g"; "EtalonTEC" format="%.2g"; "OffLineTEC" min=0.0 max=30.0 step=0.1 format="%.3g"; "OnLineTEC" min=0.0 max=30.0 step=0.1 format="%.3g"}
  in  "Device In":refnum<visa-resource-name>="Pro8000"
  in  "Pulse B Polarity":enum32{"Low", "High"}(ring)=enum."High"
  in  "Pulse A Delay(ns)":u32=1040 min=80 max=327600
  in  "Pulse B Delay(ns)":u32=170000 min=80 max=327600 step=1
  in  "Accumulation Delay(ns)":u32=10 min=10 max=1270 step=1
  in  "Sync Pulse Polarity":enum32{"Low", "High"}(ring)=enum."High"
  in  "Pulse A Polarity":enum32{"Low", "High"}(ring)=enum."High"
  in  "Number of Bins":u32=280 min=2 max=4095 step=1
  in  "Number of Accumulates":u32=10000 min=1 max=32767 step=1
  in  "Time Resolution Per Bin(ns)":u32=500 min=5 max=1063 step=1
  out "AMCS_Profile":i32=8
  in  "Lambda On Set (nm)":dbl=780.24612 format="%.5f"
  out "Lambda On Read (nm)":dbl=780.2461242779644 format="%.5f"
  out "Lambda Off Read (nm)":dbl=780.2461341945711 format="%.5f"
  in  "Lambda Off Set (nm)":dbl=780.24612 format="%#.5f"
  in  "Bristol In":i32=5
  out "Bristol Out":i32
  out "WL_Difference":dbl=4.27796442181716e-06 format="%#_3e"
  out "WL Difference off":dbl=1.4194571122061461e-05 format="%#_3e"
  out "Wavelength Lock Online":bool=TRUE
  out "Wavelength Lock Offline":bool=TRUE
  in  "calculate absorption cross sections":bool
  in  "Online_Tol":dbl=5e-05 format="%#_15g"
  in  "Cancel online":bool
  in  "Offline_Tol":dbl=0.001 format="%#_15g"
  in  "Cancel Offline":bool
  in  "y":dbl=0.00025 format="%#_6p"
  in  "Smoothing Range":dbl=150.0
  in  "Total DIAL Integration Time (Minutes)":i32=3
  in  "Data Reads (number of loops)":i32=1
  in  "Total Aerosol Integration Time (Minutes)":dbl=0.5
  in  "Scalar Wait Time":u32
  out "Smoothed Bins":dbl=2.0
  in  "NewportIn":string
  in  "logging":bool
  out "Newport Device Key":string="1918-R 15120"
  in  "SampleSize":i32=2
  out "NewportRef":refnum<k24>
  in  "Switch Comm Port":refnum<visa-resource-name>="COM3"
  out "FF_On_Ref":refnum<file>
  out "FF_On_Ptr":i64=2459600 format="%.2p"
  out "FF_Off_Ref":refnum<file>
  out "FF_Off_Ptr":i64=2459600 format="%.2p"
  out "NF_On_Ref":refnum<file>
  out "NF_On_Ptr":i64=2459600 format="%.2p"
  out "NF_Off_Ref":refnum<file>
  out "NF_Off_Ptr":i64=2459600 format="%.2p"
  out "DataOpen":bool=TRUE
  out "File Path_Far Field (out)":string="C:\\Users\\H2ODial\\Desktop\\SharedTeleWVData\\170222FF\\00"
  out "File Path_Near Field (out)":string="C:\\Users\\H2ODial\\Desktop\\SharedTeleWVData\\170222NF\\00"
  in  "Data File DIR (in)":string="C:\\Users\\H2ODial\\Desktop\\SharedTeleWVData\\"
  out "TRHP":T8={"Temp C"=17.615079365079367, "RelH %"=11.878815628815628, "Press hPa"=834.8901098901099, "AbH g/m^3"=1.2820512820512822}
  in  "WS visa":refnum<visa-resource-name>="LuftWS"
  in  "WS_On/Off":bool=TRUE
  in  "bins":u32=280 min=2 max=4095 step=1
  out "y offset":u32=10
  in  "ns scale":u32=500
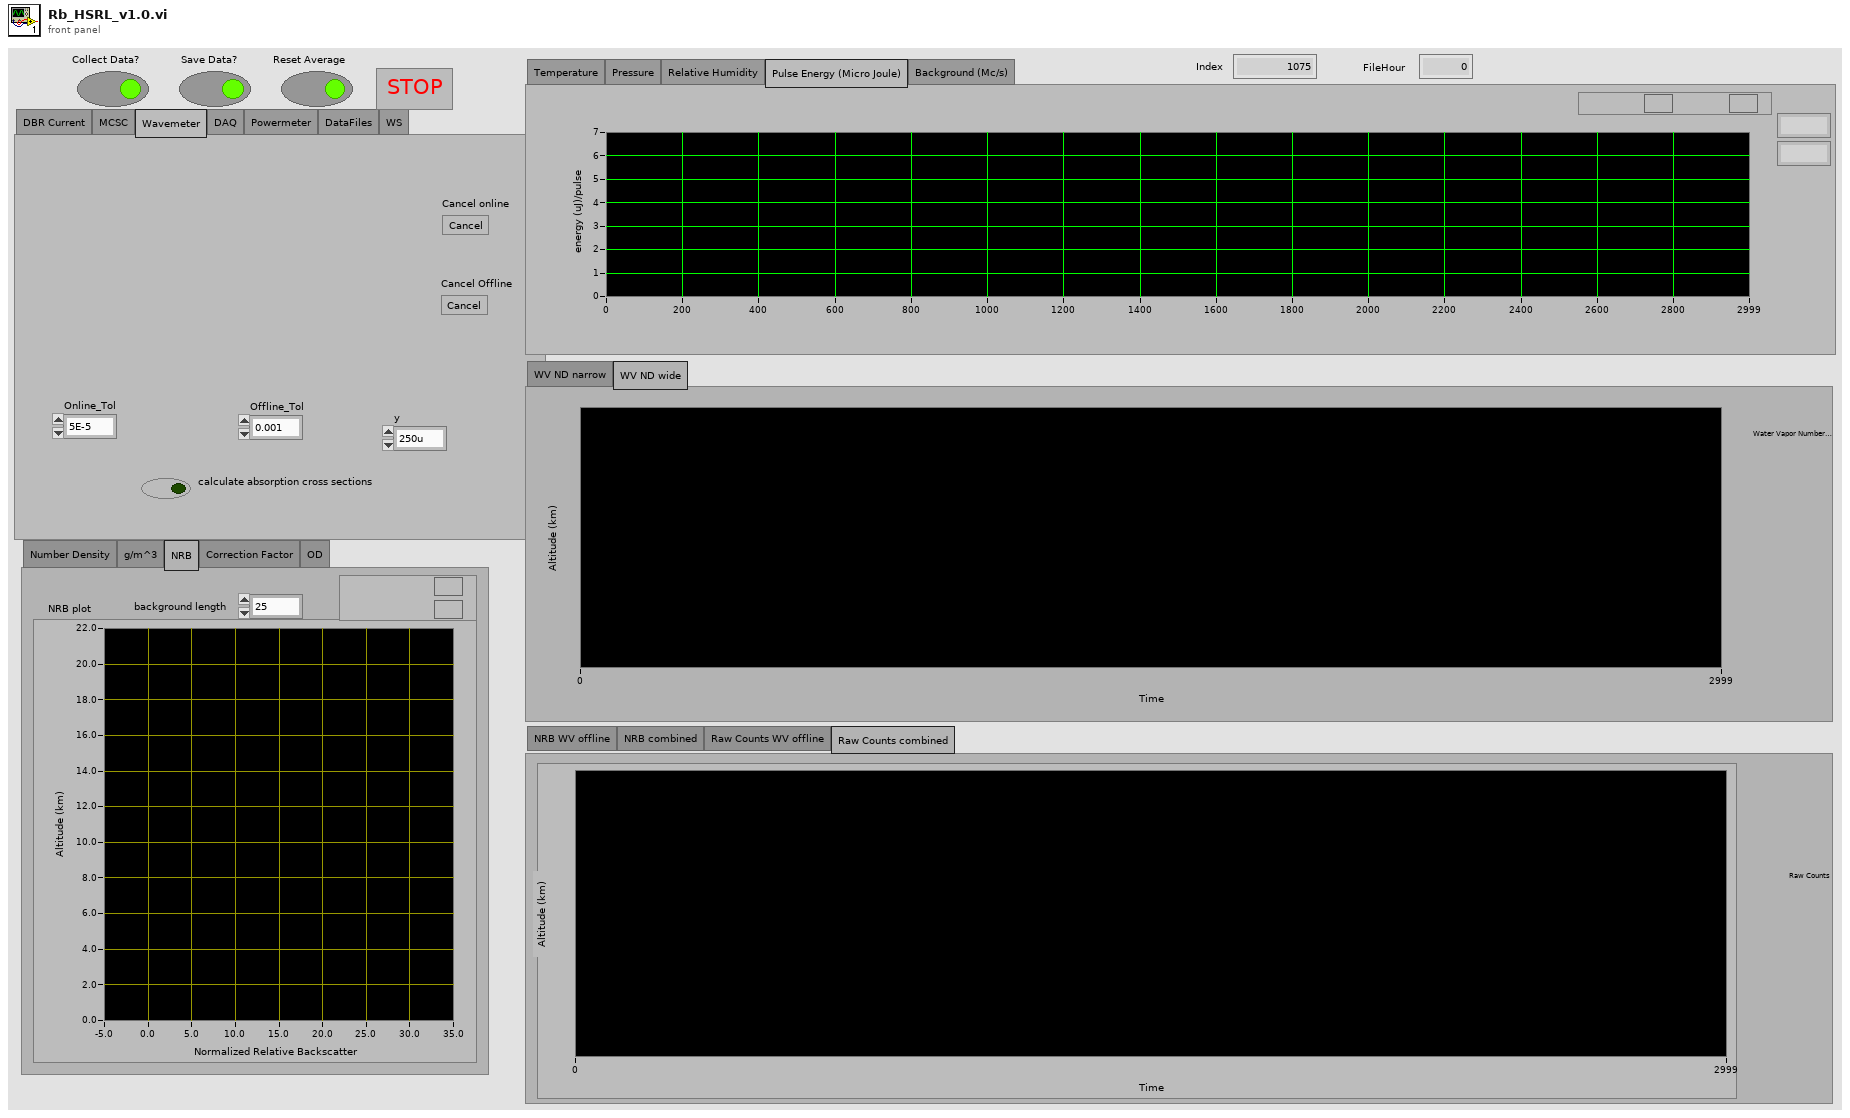
[diagram p1: front panel]
types:
  T1 = enum32{"NRB WV offline", "NRB combined", "Raw Counts WV offline", "Raw Counts combined"}
  T2 = enum32{"Number Density", "g/m^3", "NRB", "Correction Factor", "OD"}
  T3 = enum32{"Temperature", "Pressure", "Relative Humidity", "Pulse Energy (Micro Joule)", "Background (Mc/s)"}
  T4 = cluster{"Online Pulse Energy":dbl, "Pulse Energy Offline":dbl}
  T5 = enum32{"DBR Current", "MCSC", "Wavemeter", "DAQ", "Powermeter", "DataFiles", "WS"}
  T6 = cluster{"OnLineTEC":dbl, "OnLineLD":dbl, "OffLineTEC":dbl, "OffLineLD":dbl, "EtalonTEC":dbl, "TSOA-TEC":dbl, "Pro8000":bool, "OnLine TEC":bool, "OnLine LD":bool, "OffLine TEC":bool, "OffLine LD":bool, "Etalon TEC":bool, "TSOA TEC":bool}
  T7 = cluster{"Module":enum16{"On Line TEC", "On Line LD", "Off Line TEC", "Off Line LD", "Etalon TEC", "TSOA TEC"}, "OnLineTEC":dbl, "OnLineLD":dbl, "OffLineTEC":dbl, "OffLineLD":dbl, "EtalonTEC":dbl, "TSOA-TEC":dbl}
  T8 = cluster{"Temp C":dbl, "RelH %":dbl, "Press hPa":dbl, "AbH g/m^3":dbl}
  T9 = enum16{"Open_TL", "Close_TL", "Verify_ID", "TEC_Sensor", "SET", "READ", "ON", "OFF", "Set_Limits", "Read_Limits", "Enable_Status", "Read_Status"}
  T10 = enum16{"Initialize ILX", "Set ON T", "Set Off T", "Set ON I", "Set Off I", "Set On Lim", "Set Off Lim", "Read ILX", "TEC ON/OFF", "LASER ON/OFF", "Status?", "ILX OFF"}
  T11 = enum16{"open", "replace", "create", "open or create", "replace or create", "replace or create with confirmation"}
  T12 = enum16{"On Line TEC", "On Line LD", "Off Line TEC", "Off Line LD", "Etalon TEC", "TSOA TEC"}
  T13 = cluster{"Temp":dbl, "RelH":dbl, "Press":dbl, "AbH":dbl}
  T14 = typedef "LVDateTimeRec.ctl" = cluster{"fractional second":dbl, "second":i32, "minute":i32, "hour":i32, "day of month":i32, "month":i32, "year":i32, "day of week":i32, "day of year":i32, "DST":i32}
  T15 = cluster{"Online Pulse Energy":dbl, "Offline Pulse Energy":dbl}
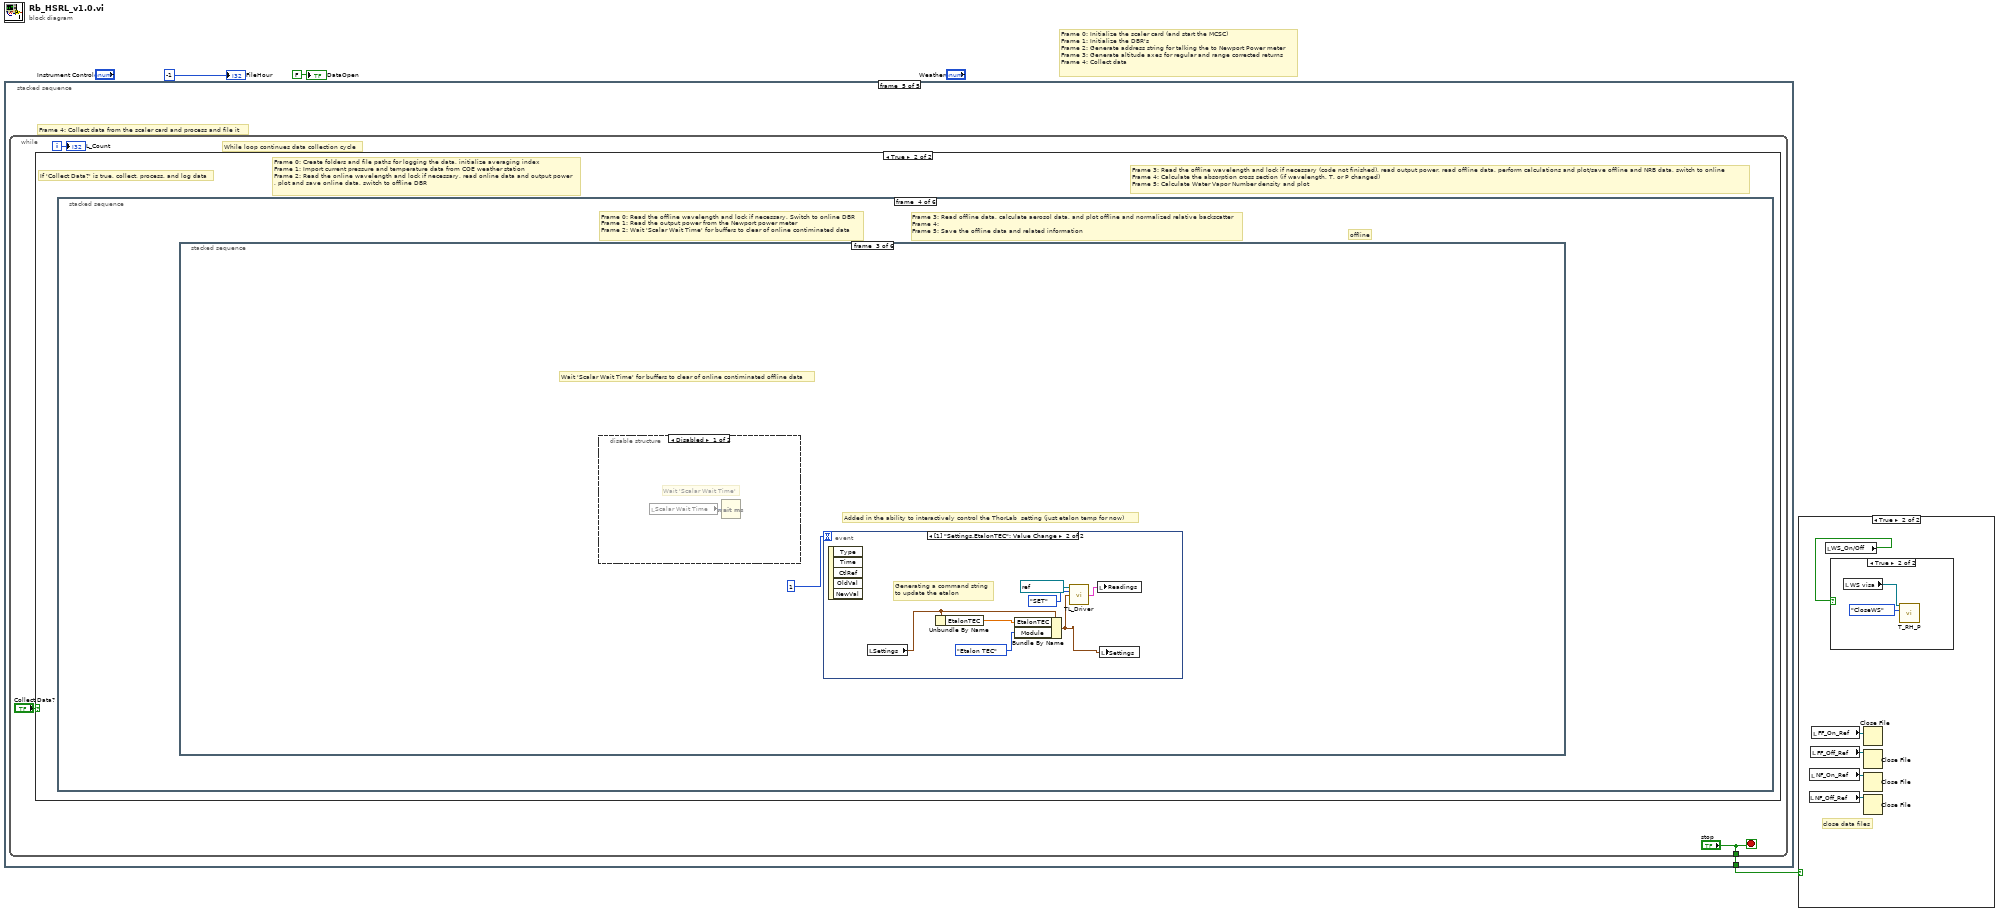
[diagram p0: block diagram]
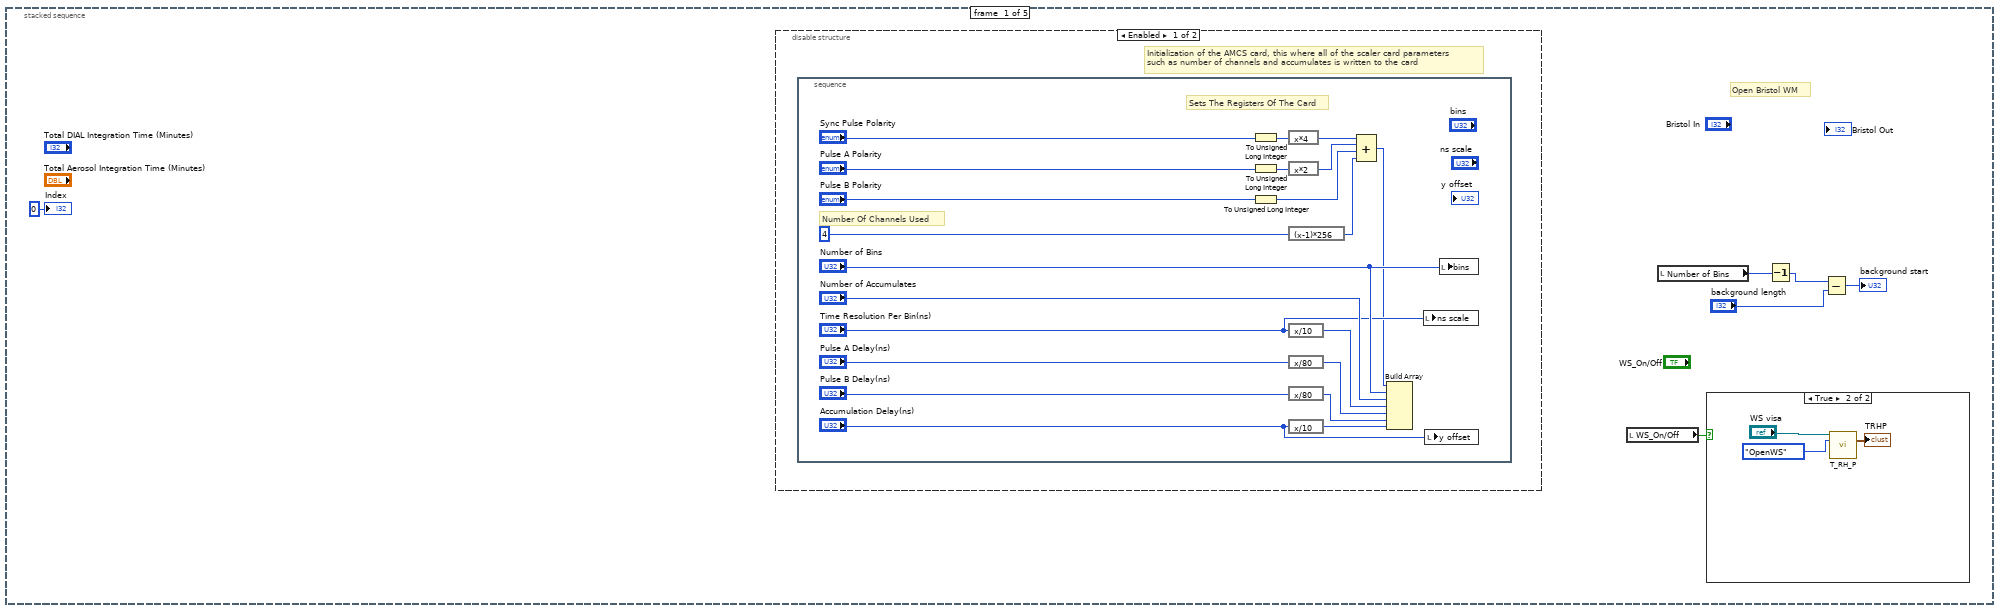
[diagram p4: hidden frame]
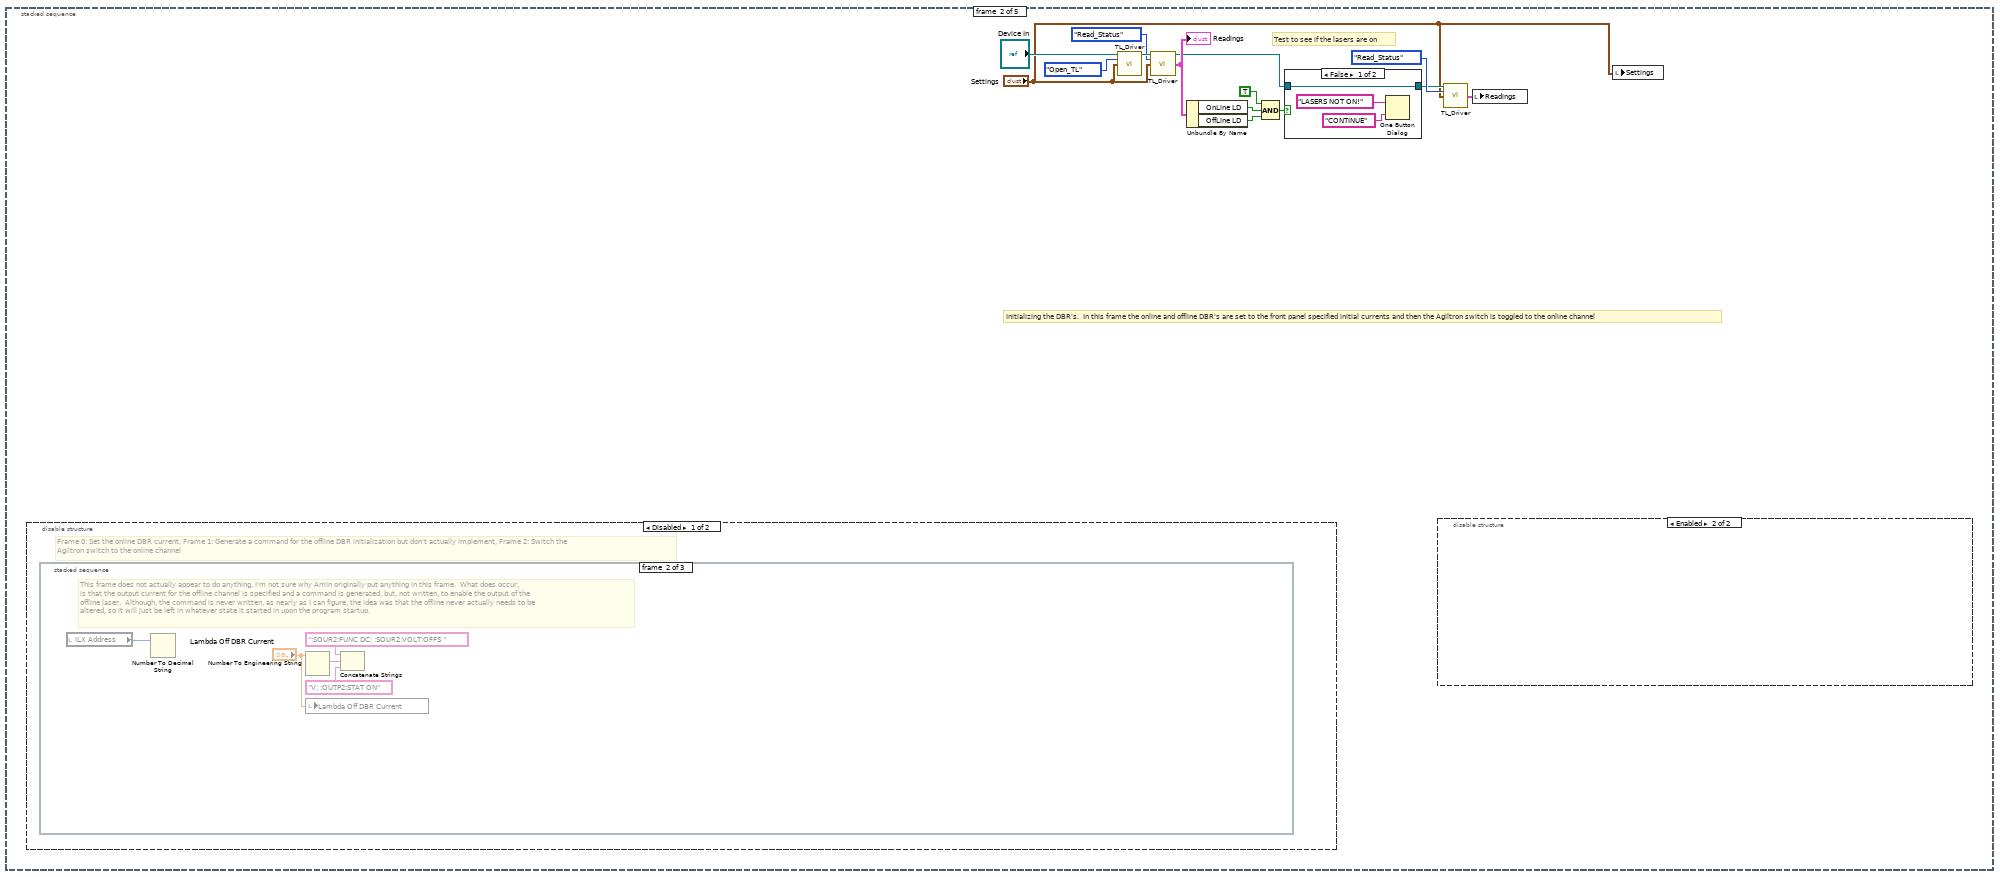
[diagram p7: hidden frame]
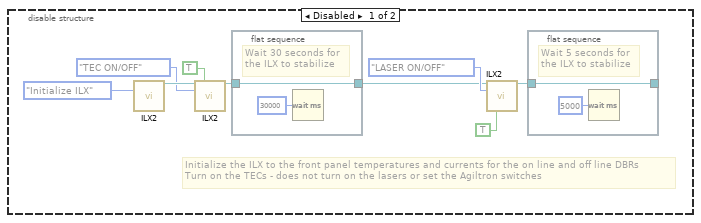
[diagram p9: hidden frame]
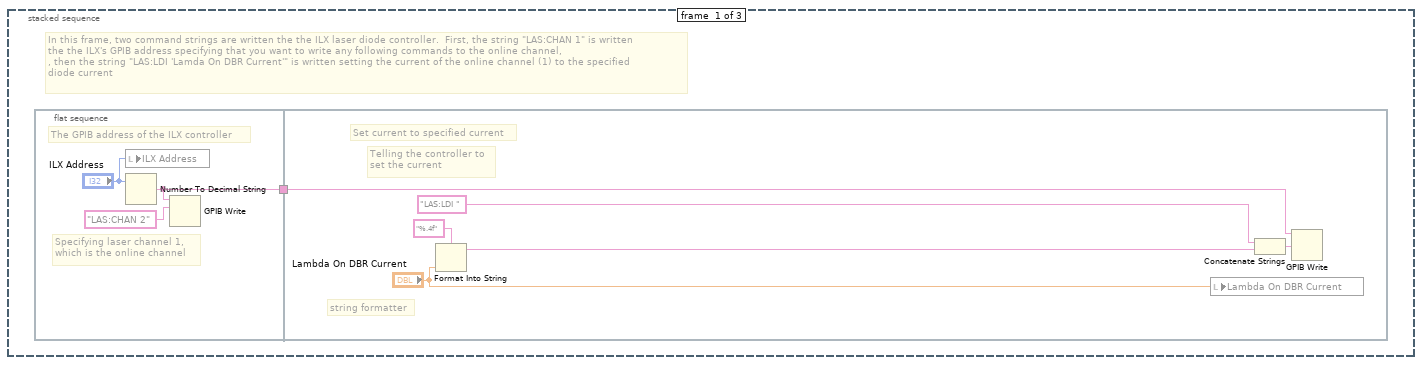
[diagram p10: hidden frame]
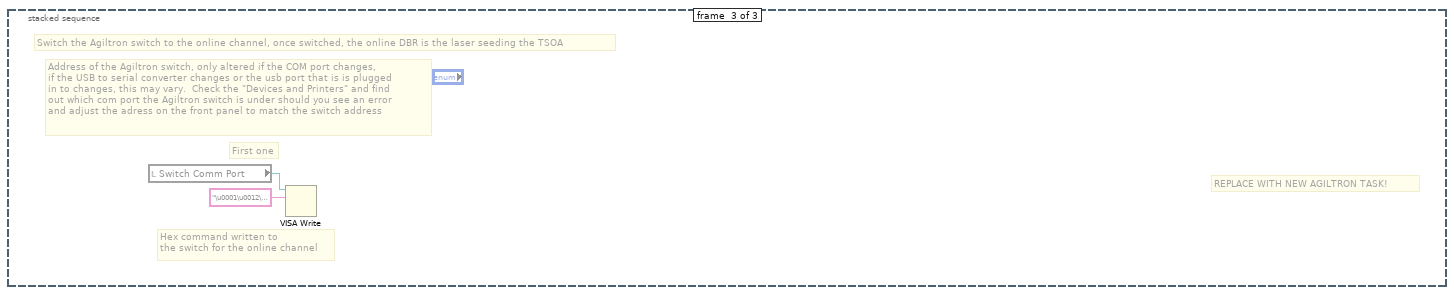
[diagram p11: hidden frame]
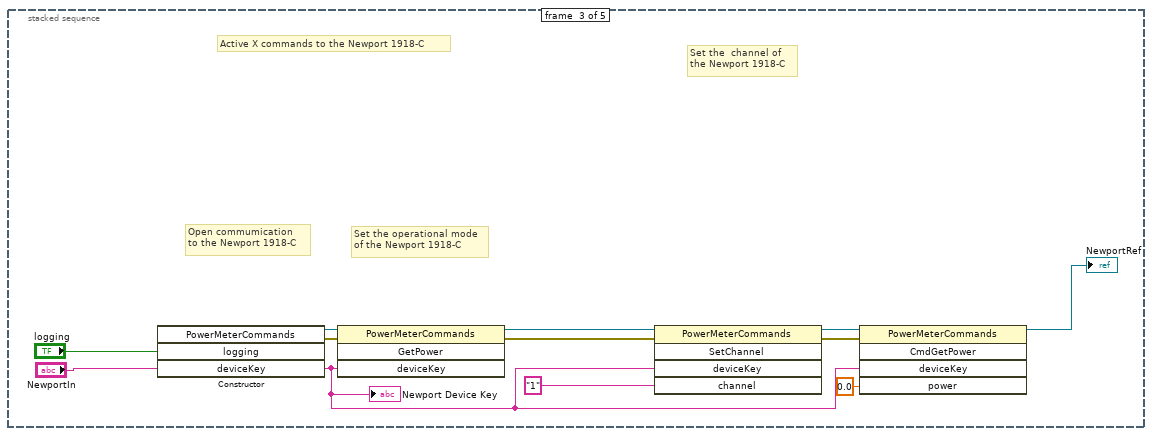
[diagram p13: hidden frame]
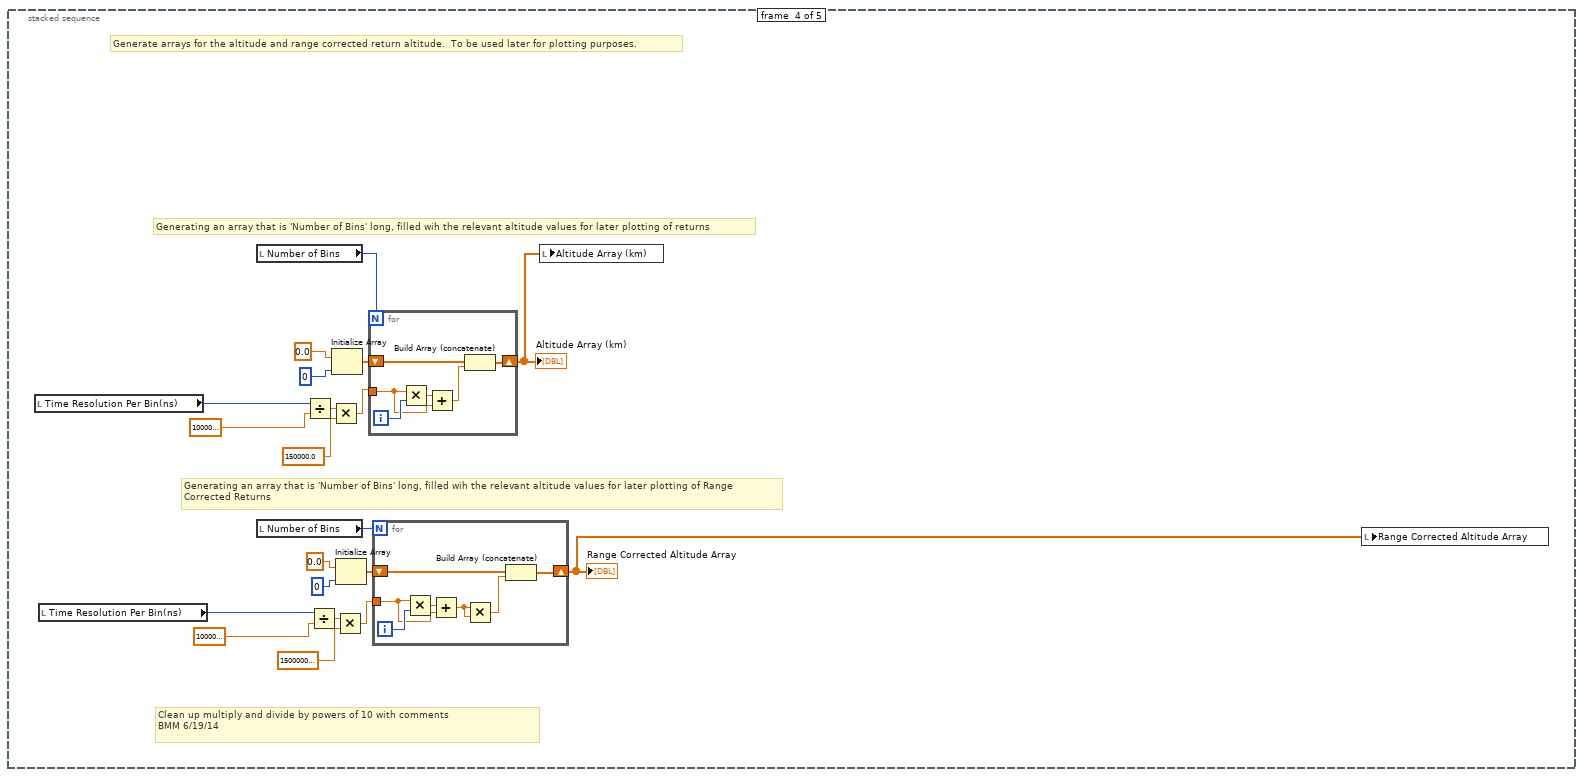
[diagram p14: hidden frame]
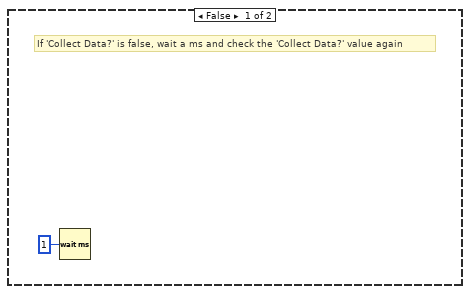
[diagram p15: hidden frame]
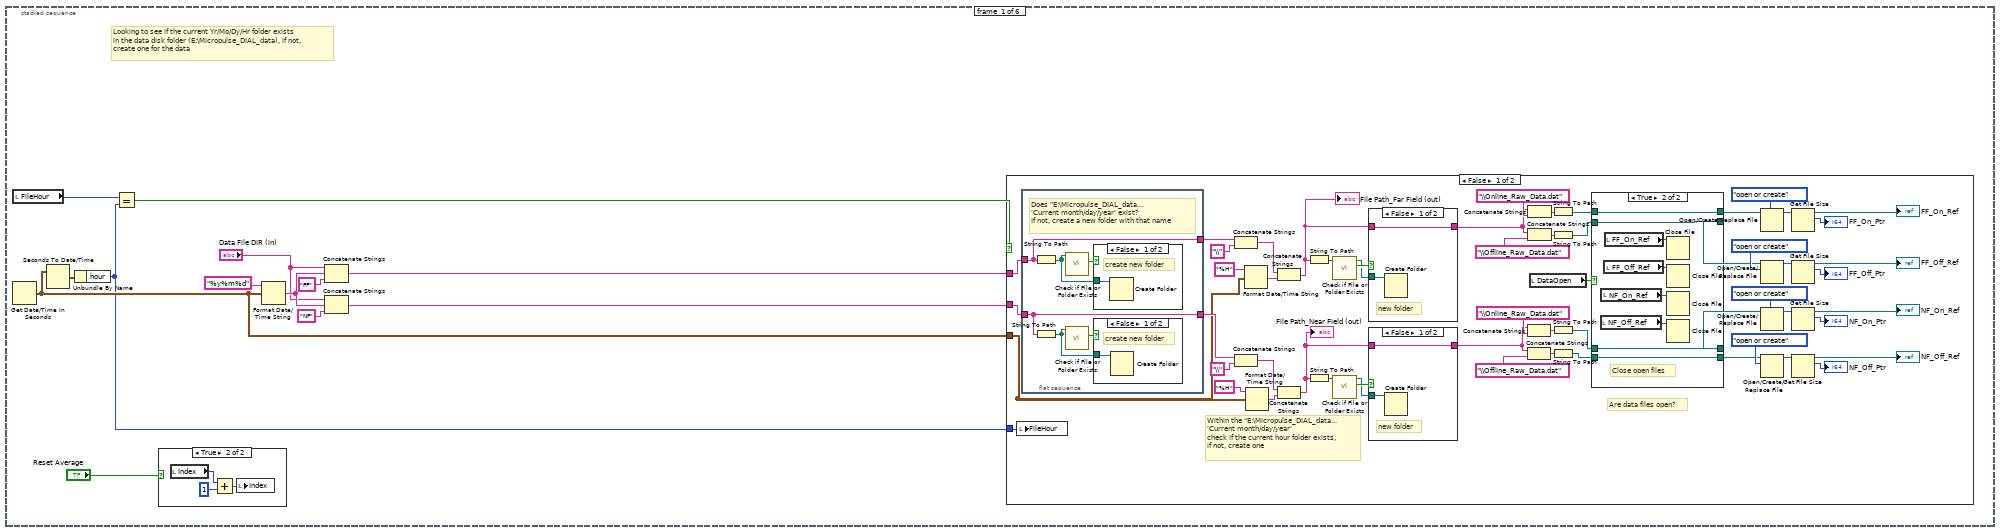
[diagram p16: hidden frame]
diagram:
  # "Frame 0: Initialize the scaler card (and start the MCSC)\nFrame 1: Initialize the DBR's\nFrame 2: Generate address string for talking the to Newport Power meter\nFrame 3: Generate altitude axes for regular and range corrected returns\nFrame 4: Collect data"
  n1 = stacked-sequence {
    tunnel: [_ _ _ _ w127] -> w3
    frame #0 {
      # "Open Bristol WM"
      n2 = disable-structure shown="Enabled" {
        frame Enabled {
          # "Initialization of the AMCS card, this where all of the scaler card parameters\nsuch as number of channels and accumulates is written to the card"
          n3 = stacked-sequence {
            frame #0 {
              # "Sets The Registers Of The Card"
              # "Number Of Channels Used"
              n4 = To Unsigned Long Integer(number="Sync Pulse Polarity") -> (unsigned 32bit integer=w13:u32)
              n5 = To Unsigned Long Integer(number="Pulse A Polarity") -> (unsigned 32bit integer=w17:u32)
              n6 = To Unsigned Long Integer(number="Pulse B Polarity") -> (unsigned 32bit integer=w15:u32)
              n7 = expression code="x*4"(w13) -> (w22:u32)
              n8 = expression code="x*2"(w17) -> (w21:u32)
              n9 = expression code="(x-1)*256"(u32 4 ("Number of Channels Used")) -> (w20:u32)
              n10 = expression code="x/10"("Time Resolution Per Bin(ns)") -> (w24:u32)
              n11 = expression code="x/80"("Pulse A Delay(ns)") -> (w31:u32)
              n12 = expression code="x/80"("Pulse B Delay(ns)") -> (w33:u32)
              n13 = expression code="x/10"("Accumulation Delay(ns)") -> (w32:u32)
              n14 = Compound Arithmetic op=ADD(w22, w21, w15, w20) -> (w19:u32)
              n15 = Build Array(w19, "Number of Bins", "Number of Accumulates", w24, w31, w33, w32) -> ()  [unwired: 1 out]
              n16 = local write "ns scale"("Time Resolution Per Bin(ns)") -> ()
              n17 = local write "y offset"("Accumulation Delay(ns)") -> ()
              n18 = local write "bins"("Number of Bins") -> ()
            }
          }
        }
        frame Disabled {
        }
      }
      n19 = local read "WS_On/Off"() -> (w4:bool)
      n20 = local read "Number of Bins"() -> (w8:u32)
      n21 = case shown="True" w4 {
        frame False {
        }
        frame True {
          n22 = call "T_RH_P.vi"("VISA in"="WS visa", "WS_Commands"=enum16{"OpenWS", "ReadTRHP", "CloseWS"}."OpenWS") -> ("TRHP"=→"TRHP":T13)  [unwired: 11 in, 2 out]
        }
      }
      n23 = Decrement(x=w8) -> (x-1=w7:u32)
      n24 = Subtract(x=w7, y="background length") -> (x-y=→"background start":u32)
      "Index" <- 0 ("Index")
    }
    frame #1 {
      # "Test to see if the lasers are on"
      # "Initializing the DBR's.  In this frame the online and offline DBR's are set to the front panel specified initial currents and then the Agiltron switch is toggled to the online channel"
      n25 = disable-structure shown="Disabled" {
        frame Disabled {
          # "Frame 0: Set the online DBR current, Frame 1: Generate a command for the offline DBR initialization but don't actually implement, Frame 2: Switch the \nAgiltron switch to the online channel"
          n26 = stacked-sequence {
            frame #0 {
              # "In this frame, two command strings are written the the ILX laser diode controller.  First, the string \"LAS:CHAN 1\" is written\nthe the ILX's GPIB address specifying that you want to write any following commands to the online channel,\n, then the string \"LAS:LDI 'Lamda On DBR Current'\" is written setting the current of the online channel (1) to the specified \ndiode current"
              n27 = flat-sequence {
                tunnel: [w67] -> w65
                tunnel: w65 -> [w69]
                frame #0 {
                  # "The GPIB address of the ILX controller"
                  # "Specifying laser channel 1,\nwhich is the online channel"
                  n28 = local write "ILX Address"("ILX Address") -> ()
                  n29 = Number To Decimal String(number="ILX Address") -> (decimal integer string=w67:string)  [unwired: 1 in]
                  n30 = GPIB Write(0:w67, 1:"LAS:CHAN 2") -> ()  [unwired: 3 in, 2 out]
                }
                frame #1 {
                  # "Telling the controller to\nset the current"
                  # "string formatter"
                  # "Set current to specified current"
                  n31 = Format Into String(format string="%.4f" ("Format String"), "Lambda On DBR Current") -> (resulting string=w72:string)  [unwired: 2 in, 1 out]
                  n32 = local write "Lambda On DBR Current"("Lambda On DBR Current") -> ()
                  n33 = Concatenate Strings("LAS:LDI ", w72) -> (w73:string)
                  n34 = GPIB Write(0:w69, 1:w73) -> ()  [unwired: 3 in, 2 out]
                }
              }
            }
            frame #1 {
              # "This frame does not actually appear to do anything, I'm not sure why Amin originally put anything in this frame.  What does occur, \nis that the output current for the offline channel is specified and a command is generated, but, not written, to enable the output of the\noffline laser.  Although, the command is never written, as nearly as I can figure, the idea was that the offline never actually needs to be \naltered, so it will just be left in whatever state it started in upon the program startup."
              n35 = local read "ILX Address"() -> (w75:i32)
              n36 = Number To Decimal String(number=w75) -> ()  [unwired: 1 in, 1 out]
              n37 = Number To Engineering String(4:"Lambda Off DBR Current") -> (0:w79:string)  [unwired: 3 in]
              n38 = local write "Lambda Off DBR Current"("Lambda Off DBR Current") -> ()
              n39 = Concatenate Strings(":SOUR2:FUNC DC; :SOUR2:VOLT:OFFS ", w79, "V; :OUTP2:STAT ON") -> ()  [unwired: 1 out]
            }
            frame #2 {
              # "REPLACE WITH NEW AGILTRON TASK!"
              # "First one"
              # "Address of the Agiltron switch, only altered if the COM port changes,\nif the USB to serial converter changes or the usb port that is is plugged\nin to changes, this may vary.  Check the \"Devices and Printers\" and find \nout which com port the Agiltron switch is under should you see an error \nand adjust the adress on the front panel to match the switch address"
              # "Hex command written to \nthe switch for the online channel"
              # "Switch the Agiltron switch to the online channel, once switched, the online DBR is the laser seeding the TSOA"
              n40 = local read "Switch Comm Port"() -> (w80:refnum<visa-resource-name>)
              n41 = VISA Write(VISA resource name=w80, write buffer="\u0001\u0012\u0000\u0002") -> ()  [unwired: 1 in, 3 out]
            }
          }
        }
        frame Enabled {
        }
      }
      n42 = call "TL_Driver.vi"("Device In"="Device In", "Commands"=T9."Open_TL", "Settings"="Settings") -> ("Device Out"=w45:refnum<visa-resource-name>)  [unwired: 9 in, 3 out]
      n43 = call "TL_Driver.vi"("Device In"=w45, "Commands"=T9."Read_Status", "Settings"="Settings") -> ("Device Out"=w42:refnum<visa-resource-name>, "Readings"=w43:T6)  [unwired: 9 in, 2 out]
      "Readings" <- w43
      n44 = Unbundle By Name(w43) -> ("OnLine LD"=w37:bool, "OffLine LD"=w38:bool)
      n45 = Compound Arithmetic op=AND(TRUE, w37, w38) -> (w36:bool)
      n46 = case shown="False" w36 {
        tunnel: w42 -> [w48 w51]
        tunnel: [w48 w51] -> w40
        frame False {
          n47 = One Button Dialog(message="LASERS NOT ON!", button name ("OK")="CONTINUE") -> ()  [unwired: 1 out]
        }
        frame True {
        }
      }
      n48 = disable-structure shown="Enabled" {
        frame Disabled {
          # "Initialize the ILX to the front panel temperatures and currents for the on line and off line DBRs\nTurn on the TECs - does not turn on the lasers or set the Agiltron switches"
          n49 = call "ILX2.vi"("ILX Command"=T10."Initialize ILX") -> ("Device Out"=w59:refnum<visa-resource-name>)  [unwired: 10 in, 4 out]
          n50 = call "ILX2.vi"("Device In"=w59, "TEC Control"=TRUE, "ILX Command"=T10."TEC ON/OFF") -> ("Device Out"=w56:refnum<visa-resource-name>)  [unwired: 8 in, 4 out]
          n51 = flat-sequence {
            tunnel: w56 -> [w63]
            tunnel: [w63] -> w53
            frame #0 {
              # "Wait 30 seconds for\nthe ILX to stabilize"
              n52 = Wait (ms)(milliseconds to wait=u32 30000) -> ()  [unwired: 1 out]
            }
          }
          n53 = call "ILX2.vi"("Device In"=w53, "ILX Command"=T10."LASER ON/OFF", "Laser Control"=TRUE ("TEC Control")) -> ("Device Out"=w52:refnum<visa-resource-name>)  [unwired: 8 in, 4 out]
          n54 = flat-sequence {
            tunnel: w52 -> [w61]
            tunnel: [w61] -> _
            frame #0 {
              # "Wait 5 seconds for\nthe ILX to stabilize"
              n55 = Wait (ms)(milliseconds to wait=u32 5000) -> ()  [unwired: 1 out]
            }
          }
        }
        frame Enabled {
        }
      }
      n56 = call "TL_Driver.vi"("Device In"=w40, "Commands"=T9."Read_Status", "Settings"="Settings") -> ("Readings"=w34:T6)  [unwired: 9 in, 3 out]
      n57 = local write "Readings"(w34) -> ()
      n58 = local write "Settings"("Settings") -> ()
    }
    frame #2 {
      # "Active X commands to the Newport 1918-C"
      # "Set the  channel of\nthe Newport 1918-C"
      # "Set the operational mode\nof the Newport 1918-C"
      # "Open commumication\nto the Newport 1918-C"
      n59 = constructor class="PowerMeterCommands"("logging"="logging", "deviceKey"="NewportIn") -> (reference out=w93:refnum<k24>, error out=w90:errorcluster, "deviceKey"=w85:string)  [unwired: 3 in, 2 out]
      "Newport Device Key" <- w85
      n60 = invoke class="PowerMeterCommands" method="GetPower"(reference=w93, error in=w90, "deviceKey"=w85) -> (reference out=w92:refnum<k24>, error out=w89:errorcluster)  [unwired: 1 in, 2 out]
      n61 = invoke class="PowerMeterCommands" method="SetChannel"(reference=w92, error in=w89, "deviceKey"=w85, "channel"="1") -> (reference out=w86:refnum<k24>, error out=w88:errorcluster)  [unwired: 1 in, 3 out]
      n62 = invoke class="PowerMeterCommands" method="CmdGetPower"(reference=w86, error in=w88, "deviceKey"=w85, "power"=sgl 0.0) -> (reference out=→"NewportRef":refnum<k24>)  [unwired: 1 in, 4 out]
    }
    frame #3 {
      # "Clean up multiply and divide by powers of 10 with comments\nBMM 6/19/14"
      # "Generating an array that is 'Number of Bins' long, filled wih the relevant altitude values for later plotting of Range \nCorrected Returns"
      # "Generating an array that is 'Number of Bins' long, filled wih the relevant altitude values for later plotting of returns"
      # "Generate arrays for the altitude and range corrected return altitude.  To be used later for plotting purposes."
      n63 = local read "Time Resolution Per Bin(ns)"() -> (w106:u32)
      n64 = local read "Time Resolution Per Bin(ns)"() -> (w96:u32)
      n65 = local read "Number of Bins"() -> (w109:u32)
      n66 = local read "Number of Bins"() -> (w99:u32)
      n67 = Divide(x=w106, y=1000000000.0) -> (x/y=w104:dbl)
      n68 = Divide(x=w96, y=1000000000.0) -> (x/y=w94:dbl)
      n69 = Multiply(x=w104, y=150000.0) -> (x*y=w107:dbl)
      n70 = Initialize Array(0.0, 0) -> (w112:dbl[])
      n71 = Multiply(x=w94, y=150000000.0) -> (x*y=w97:dbl)
      n72 = Initialize Array(0.0, 0) -> (w102:dbl[])
      n73 = for {
        N: w109 -> [_]
        shift-right: [w125] -> w110
        shift-left: w112 -> [w126]
        tunnel: w107 -> [w122]
        i -> [w124]
        n74 = Multiply(x=w122, y=w124) -> (x*y=w123:dbl)
        n75 = Add(x=w123, y=w122) -> (x+y=w121:dbl)
        n76 = Build Array (concatenate)(w126, w121) -> (w125:dbl[])
      }
      "Altitude Array (km)" <- w110
      n77 = for {
        N: w99 -> [_]
        shift-right: [w119] -> w100
        shift-left: w102 -> [w120]
        tunnel: w97 -> [w115]
        i -> [w118]
        n78 = Multiply(x=w115, y=w118) -> (x*y=w116:dbl)
        n79 = Add(x=w116, y=w115) -> (x+y=w114:dbl)
        n80 = Multiply(x=w114, y=w114) -> (x*y=w117:dbl)
        n81 = Build Array (concatenate)(w120, w117) -> (w119:dbl[])
      }
      "Range Corrected Altitude Array" <- w100
      n82 = local write "Altitude Array (km)"(w110) -> ()
      n83 = local write "Range Corrected Altitude Array"(w100) -> ()
    }
    frame #4 {
      # "Frame 4: Collect data from the scaler card and process and file it"
      n84 = while {
        tunnel: ["stop"] -> w127
        i -> [w128]
        stop <- "stop" stop-if-true
        # "While loop continues data collection cycle"
        n85 = case shown="True" "Collect Data?" {
          frame False {
            # "If 'Collect Data?' is false, wait a ms and check the 'Collect Data?' value again"
            n86 = Wait (ms)(milliseconds to wait=u32 1) -> ()  [unwired: 1 out]
          }
          frame True {
            # "Frame 3: Read the offline wavelength and lock if necessary (code not finished), read output power, read offline data, perform calculations and plot/save offline and NRB data, switch to online\nFrame 4: Calculate the absorption cross section (if wavelength, T, or P changed)\nFrame 5: Calculate Water Vapor Number density and plot"
            # "Frame 0: Create folders and file paths for logging the data, initialize averaging index\nFrame 1: Import current pressure and temperature data from COE weather station\nFrame 2: Read the online wavelength and lock if necessary, read online data and output power\n, plot and save online data, switch to offline DBR"
            # "If 'Collect Data?' is true, collect, process, and log data"
            n87 = stacked-sequence {
              frame #0 {
                # "Looking to see if the current Yr/Mo/Dy/Hr folder exists\nin the data disk folder (E:\\Micropulse_DIAL_data), if not,\ncreate one for the data"
                n88 = local read "FileHour"() -> (w141:i32)
                n89 = Get Date/Time In Seconds() -> (seconds since 1Jan1904=w133:timestamp)
                n90 = Seconds To Date/Time(time stamp (now)=w133) -> (date time rec=w143:T14)  [unwired: 1 in]
                n91 = Unbundle By Name(w143) -> ("hour"=w132:i32)
                n92 = Equal?(x=w141, y=w132) -> (x = y?=w142:bool)
                n93 = case shown="True" "Reset Average" {
                  frame False {
                    n94 = local write "Index"(0 ("Index")) -> ()
                  }
                  frame True {
                    n95 = local read "Index"() -> (w231:i32)
                    n96 = Add(x=w231, y=1) -> (x+y=w230:i32)
                    n97 = local write "Index"(w230) -> ()
                  }
                }
                n98 = Format Date/Time String(time format string (%c)="%y%m%d", seconds (now)=w133) -> (date/time string=w137:string)  [unwired: 1 in]
                n99 = Concatenate Strings("Data File DIR (in)", w137, "FF" ("string")) -> (w139:string)
                n100 = Concatenate Strings("Data File DIR (in)", w137, "NF" ("string")) -> (w134:string)
                n101 = case shown="False" w142 {
                  tunnel: w139 -> [w201 _]
                  tunnel: w134 -> [w200 _]
                  tunnel: w133 -> [w187 _]
                  tunnel: w132 -> [w163 _]
                  frame False {
                    # "Are data files open?"
                    # "Within the \"E:\\Micropulse_DIAL_data...\n'Current month/day/year' \ncheck if the current hour folder exists,\nif not, create one"
                    n102 = local write "FileHour"(w163) -> ()
                    n103 = flat-sequence {
                      tunnel: [w221] -> w188
                      tunnel: w201 -> [w220]
                      tunnel: w200 -> [w221]
                      tunnel: [w220] -> w189
                      frame #0 {
                        # "Does \"E:\\Micropulse_DIAL_data...\n'Current month/day/year' exist?\nIf not, create a new folder with that name"
                        n104 = String To Path(string=w220) -> (path=w225:path)
                        n105 = String To Path(string=w221) -> (path=w223:path)
                        n106 = call <vilib>:"Check if File or Folder Exists.vi"("path"=w225) -> ("file or folder exists?"=w224:bool)  [unwired: 8 in, 2 out]
                        n107 = call <vilib>:"Check if File or Folder Exists.vi"("path"=w223) -> ("file or folder exists?"=w222:bool)  [unwired: 8 in, 2 out]
                        n108 = case shown="False" w224 {
                          tunnel: w225 -> [w227 _]
                          frame False {
                            # "create new folder"
                            n109 = Create Folder(path (use dialog)=w227) -> ()  [unwired: 2 in, 3 out]
                          }
                          frame True {
                            # "Folder exists\ndo nothing"
                          }
                        }
                        n110 = case shown="False" w222 {
                          tunnel: w223 -> [w226 _]
                          frame False {
                            # "create new folder"
                            n111 = Create Folder(path (use dialog)=w226) -> ()  [unwired: 2 in, 3 out]
                          }
                          frame True {
                            # "Folder exists\ndo nothing"
                          }
                        }
                      }
                    }
                    n112 = Concatenate Strings(w189, "\\" ("string")) -> (w196:string)
                    n113 = Concatenate Strings(w188, "\\" ("string")) -> (w191:string)
                    n114 = Format Date/Time String(time format string (%c)="%H", seconds (now)=w187) -> (date/time string=w199:string)  [unwired: 1 in]
                    n115 = Format Date/Time String(time format string (%c)="%H", seconds (now)=w187) -> (date/time string=w194:string)  [unwired: 1 in]
                    n116 = Concatenate Strings(w196, w199) -> (w159:string)
                    "File Path_Far Field (out)" <- w159
                    n117 = Concatenate Strings(w191, w194) -> (w160:string)
                    "File Path_Near Field (out)" <- w160
                    n118 = String To Path(string=w159) -> (path=w197:path)
                    n119 = String To Path(string=w160) -> (path=w192:path)
                    n120 = call <vilib>:"Check if File or Folder Exists.vi"("path"=w197) -> ("file or folder exists?"=w186:bool, "dup path"=w184:path)  [unwired: 8 in, 1 out]
                    n121 = call <vilib>:"Check if File or Folder Exists.vi"("path"=w192) -> ("file or folder exists?"=w185:bool, "dup path"=w183:path)  [unwired: 8 in, 1 out]
                    n122 = case shown="False" w186 {
                      tunnel: w184 -> [w218 _]
                      tunnel: w159 -> [w217 w219]
                      tunnel: [w217 w219] -> w157
                      frame False {
                        # "new folder"
                        n123 = Create Folder(path (use dialog)=w218) -> ()  [unwired: 2 in, 3 out]
                      }
                      frame True {
                        # "Folder exists\ndo nothing"
                      }
                    }
                    n124 = case shown="False" w185 {
                      tunnel: w183 -> [w215 _]
                      tunnel: w160 -> [w214 w216]
                      tunnel: [w214 w216] -> w158
                      frame False {
                        # "new folder"
                        n125 = Create Folder(path (use dialog)=w215) -> ()  [unwired: 2 in, 3 out]
                      }
                      frame True {
                        # "Folder exists\ndo nothing"
                      }
                    }
                    n126 = Concatenate Strings(w158, "\\Online_Raw_Data.dat" ("string")) -> (w177:string)
                    n127 = Concatenate Strings(w158, "\\Offline_Raw_Data.dat" ("string")) -> (w176:string)
                    n128 = Concatenate Strings(w157, "\\Online_Raw_Data.dat" ("string")) -> (w182:string)
                    n129 = Concatenate Strings(w157, "\\Offline_Raw_Data.dat" ("string")) -> (w181:string)
                    n130 = local read "DataOpen"() -> (w174:bool)
                    n131 = String To Path(string=w182) -> (path=w173:path)
                    n132 = String To Path(string=w181) -> (path=w172:path)
                    n133 = String To Path(string=w177) -> (path=w171:path)
                    n134 = String To Path(string=w176) -> (path=w170:path)
                    n135 = case shown="True" w174 {
                      tunnel: w173 -> [w205 w209]
                      tunnel: [w205 w209] -> w167
                      tunnel: w172 -> [w204 w208]
                      tunnel: [w204 w208] -> w166
                      tunnel: w171 -> [w203 w207]
                      tunnel: [w203 w207] -> w165
                      tunnel: [w202 w206] -> w164
                      tunnel: w170 -> [w202 w206]
                      frame False {
                        # "No files open\ndo nothing"
                      }
                      frame True {
                        # "Close open files"
                        n136 = local read "NF_Off_Ref"() -> (w211:refnum<file>)
                        n137 = local read "NF_On_Ref"() -> (w210:refnum<file>)
                        n138 = local read "FF_Off_Ref"() -> (w213:refnum<file>)
                        n139 = local read "FF_On_Ref"() -> (w212:refnum<file>)
                        n140 = Close File(refnum=w212) -> ()  [unwired: 1 in, 2 out]
                        n141 = Close File(refnum=w213) -> ()  [unwired: 1 in, 2 out]
                        n142 = Close File(refnum=w210) -> ()  [unwired: 1 in, 2 out]
                        n143 = Close File(refnum=w211) -> ()  [unwired: 1 in, 2 out]
                      }
                    }
                    n144 = Open/Create/Replace File(file path (use dialog)=w167, operation (0:open)=T11."open or create") -> (refnum out=w153:refnum<file>)  [unwired: 4 in, 2 out]
                    n145 = Open/Create/Replace File(file path (use dialog)=w166, operation (0:open)=T11."open or create") -> (refnum out=w154:refnum<file>)  [unwired: 4 in, 2 out]
                    n146 = Open/Create/Replace File(file path (use dialog)=w165, operation (0:open)=T11."open or create") -> (refnum out=w155:refnum<file>)  [unwired: 4 in, 2 out]
                    n147 = Open/Create/Replace File(file path (use dialog)=w164, operation (0:open)=T11."open or create") -> (refnum out=w156:refnum<file>)  [unwired: 4 in, 2 out]
                    n148 = Get File Size(file=w153) -> (refnum out=→"FF_On_Ref":refnum<file>, size (in bytes)=→"FF_On_Ptr":i64)  [unwired: 1 in, 1 out]
                    n149 = Get File Size(file=w154) -> (refnum out=→"FF_Off_Ref":refnum<file>, size (in bytes)=→"FF_Off_Ptr":i64)  [unwired: 1 in, 1 out]
                    n150 = Get File Size(file=w155) -> (refnum out=→"NF_On_Ref":refnum<file>, size (in bytes)=→"NF_On_Ptr":i64)  [unwired: 1 in, 1 out]
                    n151 = Get File Size(file=w156) -> (refnum out=→"NF_Off_Ref":refnum<file>, size (in bytes)=→"NF_Off_Ptr":i64)  [unwired: 1 in, 1 out]
                  }
                  frame True {
                    # "Don't need to do anything!"
                  }
                }
              }
              frame #1 {
                # "Writing and plotting retrieved\nweather parameters"
                # "Matlab script goes online and retrieves most recent press, temp, and relative humidity data \nfrom the weather station on the roof of Cobleigh"
                # "Importing the current weather conditions from the COE weather station"
                n152 = disable-structure shown="Disabled" {
                  frame Disabled {
                    n153 = script code="%try\n%s=urlread('http://www.coe.montana.edu/ee/weather/mostCurrentCSV.php');\n%amin=textscan(s,'%s %s %s %s %s %s %s %s %s %s %s %s %s');\n%data=amin{1}{2};\n%[test remain]=strtok(data,',');\n%remain=str2num(remain);\n%press=remain(3)./1000;\n%temp=remain(5);\n%RH=remain(7);\n%catch\npress=.850;\ntemp=20;\nRH=40;\n%end"() -> ()  [unwired: 1 in, 4 out]
                  }
                  frame Enabled {
                  }
                }
                n154 = local read "WS_On/Off"() -> (w232:bool)
                n155 = case shown="True" w232 {
                  frame False {
                  }
                  frame True {
                    n156 = local read "WS visa"() -> (w237:refnum<visa-resource-name>)
                    n157 = call "T_RH_P.vi"("VISA in"=w237, "WS_Commands"=enum16{"OpenWS", "ReadTRHP", "CloseWS"}."ReadTRHP") -> ("TRHP"=w233:T13)  [unwired: 11 in, 2 out]
                    n158 = local write "TRHP"(w233) -> ()
                    n159 = Unbundle By Name(w233) -> ("Temp"=→"Temperature (C)":dbl, "RelH"=→"Relative Humdity (%)":dbl, "Press"=→"Pressure (mb)":dbl)
                  }
                }
              }
              frame #2 {
                # "Frame 3: Read, process, and plot online data\nFrame 4:\nFrame 5: Write the data to the folders from Frame 0 of outter sequence"
                # "Frame 0: Read the online wavelength and adjust to locking tolerance if out of range, Switch to offline DBR\nFrame 1: Read the output power from the Newport meter, calculate and plot the output pulse energy\nFrame 2: Wait 'Scalar Wait Time' for buffer to clear other wavelength data"
                # "Online"
                n160 = stacked-sequence {
                  frame #0 {
                    # "Read the online wavelength and continue adjusting the online DBR if outside the wavelength tolerance\nuntil it is within tolerance"
                    n161 = while {
                      i -> [w242]
                      stop <- w239 stop-if-true
                      # "Frame 2: Decrement DBR current if above tolerance\nFrame 3: Increment DBR current if below tolerance"
                      # "Frame 0: Read the current wavelength from the wavemeter\nFrame 1: Calculate the difference between desired and actual wavelength"
                      # "Continue reading and adjusting online DBR current until within locking tolerance"
                      n162 = stacked-sequence {
                        tunnel: w242 -> [w244 _ _ _ _]
                        tunnel: [_ _ w258 _ _] -> w240
                        frame #0 {
                          n163 = Equal To 0?(x=w244) -> (x = 0?=w243:bool)
                          n164 = case shown="True" w243 {
                            frame False {
                            }
                            frame True {
                              # "Set the TSOA switch to\namplify the ABSORBING\nwavelength"
                              n165 = Build Array(FALSE ("Boolean")) -> (w245:bool[])
                              n166 = call-poly <vilib>:"DAQmx Write.vi"("task/channels in"=refnum<k21> "BristolWM", "data"=w245) -> ()  [unwired: 11 in, 3 out]
                            }
                          }
                        }
                        frame #1 {
                          # "Reading the wavelength from the wavemeter"
                          n167 = flat-sequence {
                            tunnel: [w250] -> w249
                            tunnel: w249 -> [w253]
                            tunnel: [w252] -> w248
                            tunnel: w248 -> [w256]
                            frame #0 {
                              n168 = local read "Bristol In"() -> (w251:i32)
                              n169 = dll-call lib="C:/Users/H2ODial/Desktop/Shared Telescope WV DIAL Code/bristol/CLDevIface.dll" fn="CLOpenUSBSerialDevice"("commPort"=w251) -> ("return type"=w250:i32)  [unwired: 4 in, 2 out]
                            }
                            frame #1 {
                              n170 = dll-call lib="C:/Users/H2ODial/Desktop/Shared Telescope WV DIAL Code/bristol/CLDevIface.dll" fn="CLGetLambdaReading"("devHandle"=w253) -> ("return type"=→"Lambda On Read (nm)":dbl, "devHandle"=w252:i32)  [unwired: 3 in, 2 out]
                            }
                            frame #2 {
                              n171 = dll-call lib="C:/Users/H2ODial/Desktop/Shared Telescope WV DIAL Code/bristol/CLDevIface.dll" fn="CLCloseDevice"("commPort"=w256) -> ("return type"=w255:i32)  [unwired: 4 in, 2 out]
                              n172 = local write "Bristol Out"(w255) -> ()
                            }
                          }
                        }
                        frame #2 {
                          # "If WL difference is within tolerance, stop looping, and illuminate 'Wavelength Lock Online' indicator"
                          # "Calculating the difference between the actual and desired online wavelength"
                          n173 = local read "Lambda On Read (nm)"() -> (w257:dbl)
                          n174 = local read "Online_Tol"() -> (w263:dbl)
                          n175 = Multiply(x=-1.0, y=w263) -> (x*y=w264:dbl)
                          n176 = Subtract(x=w257, y="Lambda On Set (nm)") -> (x-y=w259:dbl)
                          "WL_Difference" <- w259
                          n177 = Greater?(x=w259, y=w264) -> (0:w260:bool)
                          n178 = Less?(x=w259, y=w263) -> (x < y?=w261:bool)
                          n179 = And(x=w260, y=w261) -> (x .and. y?=w258:bool)
                          "Wavelength Lock Online" <- w258
                        }
                        frame #3 {
                          # "If the wavelength difference is greater that 0.0002 nm, decrement the \nDBR current by 0.01 mA"
                          n180 = local read "WL_Difference"() -> (w268:dbl)
                          n181 = Greater Or Equal?(x=w268, y="Online_Tol") -> (x >= y?=w267:bool)
                          n182 = case shown="True" w267 {
                            frame False {
                              # "Wavelength difference is not greater than 0.0002 nm, do nothing"
                            }
                            frame True {
                              # "Generating a command string\nto decrement the current"
                              # "WL difference is greater than 0.0002 nm,\ndecrement the DBR current by 0.01 mA"
                              n183 = local read "Settings"() -> (w275:T7)
                              n184 = local read "y"() -> (w269:dbl)
                              n185 = Unbundle By Name(w275) -> ("OnLineTEC"=w273:dbl)
                              n186 = local read "Device In"() -> (w270:refnum<visa-resource-name>)
                              n187 = Subtract(x=w273, y=w269) -> (x-y=w272:dbl)
                              n188 = Bundle By Name(cluster=w275, "OnLineTEC"=w272, "Module"=T12."On Line TEC") -> (w277:T7)
                              n189 = call "TL_Driver.vi"("Device In"=w270, "Commands"=T9."SET", "Settings"=w277) -> ("Readings"=w276:T6)  [unwired: 9 in, 3 out]
                              n190 = local write "Settings"(w277) -> ()
                              n191 = local write "Readings"(w276) -> ()
                            }
                          }
                        }
                        frame #4 {
                          # "If WL difference is < 0.0002 nm, increment the DBR current"
                          n192 = local read "Online_Tol"() -> (w279:dbl)
                          n193 = local read "WL_Difference"() -> (w282:dbl)
                          n194 = Multiply(x=-1.0, y=w279) -> (x*y=w278:dbl)
                          n195 = Less Or Equal?(x=w282, y=w278) -> (x <= y?=w281:bool)
                          n196 = case shown="True" w281 {
                            frame False {
                              # "WL difference is no <= to -0.0002 nm, do nothing"
                            }
                            frame True {
                              # "WL difference is < -0.0002,\nincrement the DBR current by 0.01 mA"
                              # "Generating a command string\nto decrement the current"
                              n197 = local read "Settings"() -> (w291:T7)
                              n198 = Unbundle By Name(w291) -> ("OnLineTEC"=w287:dbl)
                              n199 = local read "y"() -> (w283:dbl)
                              n200 = local read "Device In"() -> (w284:refnum<visa-resource-name>)
                              n201 = Add(x=w287, y=w283) -> (x+y=w286:dbl)
                              n202 = Bundle By Name(cluster=w291, "OnLineTEC"=w286, "Module"=T12."On Line TEC") -> (w290:T7)
                              n203 = call "TL_Driver.vi"("Device In"=w284, "Commands"=T9."SET", "Settings"=w290) -> ("Readings"=w289:T6)  [unwired: 9 in, 3 out]
                              n204 = local write "Settings"(w290) -> ()
                              n205 = local write "Readings"(w289) -> ()
                            }
                          }
                        }
                      }
                      n206 = Or(x=w240, y="Cancel online") -> (x .or. y?=w239:bool)
                    }
                  }
                  frame #1 {
                    # "Converting to pulse energy, assumes 5 percent pickoff"
                    # "Reading the Newport Power meter"
                    # "Reading the output power of the laser transmitter from the Newport power meter, once read, convert to corresponding pulse energy and plot"
                    n207 = local read "Newport Device Key"() -> (w296:string)
                    n208 = local read "NewportRef"() -> (w292:refnum<k24>)
                    n209 = disable-structure shown="Disabled" {
                      frame Disabled {
                        # "Plotting the online and offling pulse energies"
                        n210 = local read "Online Pulse Energy"() -> (w307:dbl)
                        n211 = local read "Offline Pulse Energy"() -> (w306:dbl)
                        n212 = Bundle("Online Pulse Energy"=w307, "Offline Pulse Energy"=w306) -> (→"Pulse Energy (Micro Joule)":T15)  [unwired: 1 in]
                      }
                      frame Enabled {
                      }
                    }
                    n213 = Number To Decimal String(number="SampleSize") -> (decimal integer string=w294:string)  [unwired: 1 in]
                    n214 = invoke class="PowerMeterCommands" method="PerformDAQ"(reference=w292, "deviceKey"=w296, "interval"="1", "sampleSize"=w294) -> ("PerformDAQ"=w297:dbl[])  [unwired: 2 in, 5 out]
                    n215 = call-poly <vilib>:"Mean.vi"("X"=w297) -> ("mean"=w295:dbl)  [unwired: 1 out]
                    n216 = Multiply(x=w295, y=1000.0) -> (x*y=w303:dbl)
                    n217 = Divide(x=w303, y=0.05) -> (x/y=w301:dbl)
                    n218 = Divide(x=w301, y=7.0) -> (x/y=→"Online Pulse Energy":dbl)
                  }
                  frame #2 {
                    # "Wait 'Scalar Wait Time' for the next available batch of scalar card data"
                    n219 = local read "AMCS_Profile"() -> (w308:i32)
                    n220 = disable-structure shown="Disabled" {
                      frame Disabled {
                        # "Waiting 'Scalar Wait Time'"
                        n221 = Wait (ms)(milliseconds to wait="Scalar Wait Time") -> ()  [unwired: 1 out]
                      }
                      frame Enabled {
                      }
                    }
                    n222 = while {
                      tunnel: [w315] -> w309
                      tunnel: [w311] -> _
                      tunnel: w308 -> [w311]
                      stop <- w313 stop-if-true
                      n223 = global read "AMCS_Data.vi" "AMCS_Profile"() -> (w315:i32)
                      n224 = Wait (ms)(milliseconds to wait=u32 10) -> ()  [unwired: 1 out]
                      n225 = Equal?(x=w315, y=w311) -> (x = y?=w314:bool)
                      n226 = case shown="False" w314 {
                        tunnel: [TRUE FALSE] -> w313
                        frame False {
                        }
                        frame True {
                        }
                      }
                    }
                    "AMCS_Profile" <- w309
                  }
                  frame #3 {
                    # "convert time per range bin to meters\nand calculate smoothed bins using\nsmoothing range"
                    # "Plotting online cross section and smoothed online data"
                    # "Calculate the bin by bin mean of the data"
                    # "Collect 'Integration Period (Seconds)' number\nof scalar data"
                    # "Reading, processing, and plotting the online data"
                    n227 = local read "Data Reads (number of loops)"() -> (w343:i32)
                    n228 = for {
                      N: w343 -> [_]
                      tunnel: [w364] -> w355 mode=indexing
                      tunnel: [w363] -> w318 mode=indexing
                      # "Scalar Data is retrieved from Global \nVariable that scaler.vi is writing to,"
                      n229 = global read "AMCS_Data.vi" "AMCS_Data"() -> (w367:u16[][])
                      n230 = disable-structure shown="Disabled" {
                        frame Disabled {
                          n231 = global read "Scalar_Data_3.vi" "Scalar Data 3"() -> ()  [unwired: 1 out]
                          n232 = global read "Scalar_Data.vi" "Scalar Data"() -> ()  [unwired: 1 out]
                        }
                        frame Enabled {
                        }
                      }
                      n233 = Index Array(array=w367, index (row) #1=0 ("index (row)"), index (row) #2=2 ("index (row)")) -> (element #1=w364:u16[], element #2=w363:u16[])  [unwired: 2 in]
                    }
                    n234 = Transpose 2D Array(2D array=w355) -> (transposed array=w359:u16[][])
                    n235 = Transpose 2D Array(2D array=w318) -> (transposed array=w341:u16[][])
                    n236 = for {
                      tunnel: w359 -> [w369] mode=indexing
                      tunnel: [w368] -> w360 mode=indexing
                      n237 = call-poly <vilib>:"Mean.vi"("X"=w369) -> ("mean"=w368:dbl)  [unwired: 1 out]
                    }
                    n238 = for {
                      tunnel: w341 -> [w362] mode=indexing
                      tunnel: [w361] -> w342 mode=indexing
                      n239 = call-poly <vilib>:"Mean.vi"("X"=w362) -> ("mean"=w361:dbl)  [unwired: 1 out]
                    }
                    n240 = local read "bins"() -> (w335:u32)
                    n241 = Array Subset(array=w360, index=1 ("dimension size"), length=w335) -> (w347:dbl[])
                    n242 = Array Subset(array=w342, index=1 ("dimension size"), length=w335) -> (w339:dbl[])
                    n243 = local read "background length"() -> (w325:i32)
                    n244 = local read "background start"() -> (w326:u32)
                    n245 = Array Size(array=w347) -> (size(s)=w344:i32)
                    n246 = Array Size(array=w339) -> (size(s)=w336:i32)
                    n247 = Initialize Array(1.0 ("element"), w344) -> (w346:dbl[])
                    n248 = Initialize Array(1.0 ("element"), w336) -> (w338:dbl[])
                    n249 = Multiply(x=w347, y=w346) -> (x*y=w348:dbl[])
                    "On-Line Bin Readings" <- w348
                    n250 = Multiply(x=w339, y=w338) -> (x*y=w329:dbl[])
                    "On-Line Bin Readings 2" <- w329
                    n251 = local read "Total DIAL Integration Time (Minutes)"() -> (w351:i32)
                    n252 = local read "Time Resolution Per Bin(ns)"() -> (w321:u32)
                    n253 = Array Subset(array=w348, index=w326, length=w325) -> (w357:dbl[])
                    n254 = Array Subset(array=w329, index=w326, length=w325) -> (w331:dbl[])
                    n255 = call-poly <vilib>:"Mean.vi"("X"=w357) -> ("mean"=w356:dbl)  [unwired: 1 out]
                    n256 = call-poly <vilib>:"Mean.vi"("X"=w331) -> ("mean"=w332:dbl)  [unwired: 1 out]
                    n257 = Divide(x=w351, y=w343) -> (x/y=w349:dbl)
                    n258 = local read "Index"() -> (w330:i32)
                    n259 = Subtract(x=w348, y=w356) -> (x-y=w353:dbl[])
                    n260 = Subtract(x=w329, y=w332) -> (x-y=w333:dbl[])
                    n261 = To Double Precision Float(number=w321) -> (double precision float=w322:dbl)
                    n262 = Multiply(x=w349, y=60.0) -> (x*y=w327:dbl)
                    n263 = Multiply(x=w322, y=0.15) -> (x*y=w324:dbl)
                    n264 = call "Ring Buffer Online Far.vi"("Index"=w330, "Profiles to Average"=w327, "Input Array"=w353) -> ("AvgArray"=w352:dbl[])  [unwired: 7 in, 1 out]
                    n265 = call "Ring Buffer Online Near.vi"("Index"=w330, "Profiles to Average"=w327, "Input Array"=w333) -> ("AvgArray"=w334:dbl[])  [unwired: 7 in, 1 out]
                    n266 = Divide(x="Smoothing Range", y=w324) -> (x/y=w319:dbl)
                    "Smoothed Bins" <- w319
                    n267 = call "Smooth Arrray.vi"("smooth size"=w319, "Raw Array"=w352) -> ("Smoothed Array"=→"On-Line  Smoothed":dbl[])  [unwired: 9 in]
                    n268 = call "Smooth Arrray.vi"("smooth size"=w319, "Raw Array"=w334) -> ("Smoothed Array"=→"HSRL molecular Smoothed":dbl[])  [unwired: 9 in]
                    n269 = disable-structure shown="Disabled" {
                      frame Disabled {
                        n270 = script code="format long;\ncounts=sum(Online);\nif counts >=0.5e6\ntime=time;\nelse\ntime=time\nend"() -> ()  [unwired: 3 in, 2 out]
                      }
                      frame Enabled {
                      }
                    }
                  }
                  frame #4 {
                    # "Toggling the Agiltron switch to the offline DBR seed laser"
                    n271 = disable-structure shown="Disabled" {
                      frame Disabled {
                        n272 = flat-sequence {
                          frame #0 {
                            # "Second one"
                            # "Command the switch to switch to position 2\ncorresponding to the offline DBR"
                            # "Hex string command \ncorrespond to offline"
                            n273 = VISA Write(VISA resource name="Switch Comm Port", write buffer="\u0001\u0012\u0000\u0001") -> ()  [unwired: 1 in, 3 out]
                          }
                        }
                      }
                      frame Enabled {
                      }
                    }
                  }
                  frame #5 {
                    # "Save the recently collected online data if 'Save Data?' is true"
                    n274 = case shown="True" "Save Data?" {
                      frame False {
                        # "'Save Data?' is false, do nothing"
                      }
                      frame True {
                        # "'Save Data?' is true, save onfline data to the Data Disk"
                        # "Write only one copy of data at this time"
                        # "Retrieve Julian Date"
                        n275 = local read "Time Resolution Per Bin(ns)"() -> (w379:u32)
                        n276 = local read "Number of Accumulates"() -> (w377:u32)
                        n277 = local read "Number of Bins"() -> (w378:u32)
                        n278 = local read "Lambda On Read (nm)"() -> (w373:dbl)
                        n279 = local read "Lambda On DBR Current"() -> (w401:dbl)
                        n280 = local read "On-Line Bin Readings 2"() -> (w399:dbl[])
                        n281 = local read "On-Line Bin Readings"() -> (w403:dbl[])
                        n282 = local read "Online Pulse Energy"() -> (w400:dbl)
                        n283 = To Double Precision Float(number=w379) -> (double precision float=w374:dbl)
                        n284 = To Double Precision Float(number=w378) -> (double precision float=w375:dbl)
                        n285 = To Double Precision Float(number=w377) -> (double precision float=w376:dbl)
                        n286 = call "Julian_Date_2.vi"() -> ("Julian Date"=w402:dbl)  [unwired: 11 in]
                        n287 = Build Array (concatenate)(w402, w373, w401, w400, w374, w375, w376, w403) -> (w394:dbl[])
                        n288 = Build Array (concatenate)(w402, w373, w401, w400, w374, w375, w376, w399) -> (w384:dbl[])
                        n289 = local write "DataOpen"(TRUE ("DataOpen")) -> ()
                        n290 = local read "NF_On_Ref"() -> (w382:refnum<file>)
                        n291 = local read "FF_On_Ref"() -> (w398:refnum<file>)
                        n292 = local read "NF_On_Ptr"() -> (w383:i64)
                        n293 = local read "FF_On_Ptr"() -> (w397:i64)
                        n294 = Set File Position(offset (in bytes) (0)=w397, refnum=w398) -> (refnum out=w395:refnum<file>, error out=w392:errorcluster)  [unwired: 2 in]
                        n295 = Set File Position(offset (in bytes) (0)=w383, refnum=w382) -> (refnum out=w388:refnum<file>, error out=w386:errorcluster)  [unwired: 2 in]
                        n296 = Write to Binary File(file (use dialog)=w388, data=w384, error in=w386, 5:FALSE ("prepend array or string size? (T)")) -> (refnum out=w387:refnum<file>, error out=w385:errorcluster)  [unwired: 2 in, 1 out]
                        n297 = Write to Binary File(file (use dialog)=w395, data=w394, error in=w392, 5:FALSE ("prepend array or string size? (T)")) -> (refnum out=w393:refnum<file>, error out=w391:errorcluster)  [unwired: 2 in, 1 out]
                        n298 = Get File Position(4:w385, 7:w387) -> (2:w381:i64)  [unwired: 2 out]
                        n299 = Get File Position(4:w391, 7:w393) -> (2:w390:i64)  [unwired: 2 out]
                        n300 = local write "NF_On_Ptr"(w381) -> ()
                        n301 = local write "FF_On_Ptr"(w390) -> ()
                      }
                    }
                  }
                }
              }
              frame #3 {
                # "Frame 3: Read offline data, calculate aerosol data, and plot offline and normalized relative backscatter\nFrame 4:\nFrame 5: Save the offline data and related information"
                # "Frame 0: Read the offline wavelength and lock if necessary, Switch to online DBR\nFrame 1: Read the output power from the Newport power meter\nFrame 2: Wait 'Scalar Wait Time' for buffers to clear of online contiminated data"
                # "offline"
                n302 = stacked-sequence {
                  frame #0 {
                    # "Every 60 data collection cycles, read the offline DBR wavelength, and if outside of wavelength tolerance, adjust DBR current until within tolerance"
                    n303 = local read "L_Count"() -> (w405:i32)
                    n304 = Quotient & Remainder(x=w405, y=60.0) -> (x-y*floor(x/y)=w406:dbl)  [unwired: 1 out]
                    n305 = Equal To 0?(x=w406) -> (x = 0?=w404:bool)
                    n306 = case shown="True" w404 {
                      frame False {
                      }
                      frame True {
                        n307 = while {
                          i -> [w411]
                          stop <- w409 stop-if-true
                          # "If WL difference is within tolerance, stop looping, and illuminate 'Wavelength Lock Offline' indicator"
                          # "Frame 2: Decrement DBR current if above tolerance\nFrame 3: Increment DBR current if below tolerance"
                          # "Frame 0: Read the current wavelength from the wavemeter\nFrame 1: Calculate the difference between desired and actual wavelength"
                          # "Continue reading and adjusting offline DBR current until within locking tolerance"
                          n308 = stacked-sequence {
                            tunnel: w411 -> [w413 _ _ _ _]
                            tunnel: [_ _ w427 _ _] -> w408
                            frame #0 {
                              n309 = Equal To 0?(x=w413) -> (x = 0?=w412:bool)
                              n310 = case shown="True" w412 {
                                frame False {
                                }
                                frame True {
                                # "Set the TSOA switch to\namplify the non ABSORBING\nwavelength"
                                n311 = Build Array(TRUE ("Boolean")) -> (w415:bool[])
                                n312 = call-poly <vilib>:"DAQmx Write.vi"("task/channels in"=refnum<k21> "BristolWM", "data"=w415) -> ()  [unwired: 11 in, 3 out]
                                n313 = Wait (ms)(milliseconds to wait=u32 3200) -> ()  [unwired: 1 out]
                                }
                              }
                            }
                            frame #1 {
                              # "Reading the wavelength from the wavemeter"
                              n314 = flat-sequence {
                                tunnel: [w420] -> w419
                                tunnel: w419 -> [w423]
                                tunnel: [w422] -> w418
                                tunnel: w418 -> [w426]
                                frame #0 {
                                n315 = local read "Bristol In"() -> (w421:i32)
                                n316 = dll-call lib="C:/Users/H2ODial/Desktop/Shared Telescope WV DIAL Code/bristol/CLDevIface.dll" fn="CLOpenUSBSerialDevice"("commPort"=w421) -> ("return type"=w420:i32)  [unwired: 4 in, 2 out]
                                }
                                frame #1 {
                                n317 = dll-call lib="C:/Users/H2ODial/Desktop/Shared Telescope WV DIAL Code/bristol/CLDevIface.dll" fn="CLGetLambdaReading"("devHandle"=w423) -> ("return type"=→"Lambda Off Read (nm)":dbl, "devHandle"=w422:i32)  [unwired: 3 in, 2 out]
                                }
                                frame #2 {
                                n318 = dll-call lib="C:/Users/H2ODial/Desktop/Shared Telescope WV DIAL Code/bristol/CLDevIface.dll" fn="CLCloseDevice"("commPort"=w426) -> ("return type"=w425:i32)  [unwired: 4 in, 2 out]
                                n319 = local write "Bristol Out"(w425) -> ()
                                }
                              }
                            }
                            frame #2 {
                              # "Calculating the difference between the actual and desired online wavelength"
                              n320 = local read "Offline_Tol"() -> (w429:dbl)
                              n321 = local read "Lambda Off Read (nm)"() -> (w435:dbl)
                              n322 = Multiply(x=-1.0, y=w429) -> (x*y=w428:dbl)
                              n323 = Subtract(x=w435, y="Lambda Off Set (nm)") -> (x-y=w431:dbl)
                              "WL Difference off" <- w431
                              n324 = Greater?(x=w431, y=w428) -> (0:w432:bool)
                              n325 = Less?(x=w431, y=w429) -> (x < y?=w433:bool)
                              n326 = And(x=w432, y=w433) -> (x .and. y?=w427:bool)
                              "Wavelength Lock Offline" <- w427
                              n327 = case shown="True" w427 {
                                frame False {
                                }
                                frame True {
                                # "Set the TSOA switch to\namplify the ABSORBING\nwavelength"
                                n328 = Build Array(FALSE ("Boolean")) -> (w437:bool[])
                                n329 = call-poly <vilib>:"DAQmx Write.vi"("task/channels in"=refnum<k21> "BristolWM", "data"=w437) -> ()  [unwired: 11 in, 3 out]
                                n330 = Wait (ms)(milliseconds to wait=u32 3200) -> ()  [unwired: 1 out]
                                }
                              }
                            }
                            frame #3 {
                              # "If the wavelength difference is greater that 0.0002 nm, decrement the \nDBR current by 0.01 mA"
                              n331 = local read "WL Difference off"() -> (w442:dbl)
                              n332 = Greater Or Equal?(x=w442, y="Offline_Tol") -> (x >= y?=w441:bool)
                              n333 = case shown="True" w441 {
                                frame False {
                                # "Wavelength difference is not greater than 0.0002 nm, do nothing"
                                }
                                frame True {
                                # "Generating a command string\nto decrement the current"
                                n334 = local read "Settings"() -> (w449:T7)
                                n335 = Unbundle By Name(w449) -> ("OffLineTEC"=w446:dbl)
                                n336 = Subtract(x=w446, y="y") -> (x-y=w445:dbl)
                                n337 = local read "Device In"() -> (w443:refnum<visa-resource-name>)
                                n338 = Bundle By Name(cluster=w449, "OffLineTEC"=w445, "Module"=T12."Off Line TEC") -> (w450:T7)
                                n339 = call "TL_Driver.vi"("Device In"=w443, "Commands"=T9."SET", "Settings"=w450) -> ("Readings"=w451:T6)  [unwired: 9 in, 3 out]
                                n340 = local write "Settings"(w450) -> ()
                                n341 = local write "Readings"(w451) -> ()
                                }
                              }
                            }
                            frame #4 {
                              # "If WL difference is < 0.0002 nm, increment the DBR current"
                              n342 = local read "WL Difference off"() -> (w454:dbl)
                              n343 = Less Or Equal?(x=w454, y=-0.0001) -> (x <= y?=w452:bool)
                              n344 = case shown="True" w452 {
                                frame False {
                                # "WL difference is no <= to -0.0002 nm, do nothing"
                                }
                                frame True {
                                # "Generating a command string\nto decrement the current"
                                # "WL difference is less than 0.0002 nm,\nincrement the DBR current by 0.01 mA"
                                n345 = local read "Settings"() -> (w462:T7)
                                n346 = Unbundle By Name(w462) -> ("OffLineTEC"=w459:dbl)
                                n347 = local read "y"() -> (w455:dbl)
                                n348 = Add(x=w459, y=w455) -> (x+y=w458:dbl)
                                n349 = local read "Device In"() -> (w456:refnum<visa-resource-name>)
                                n350 = Bundle By Name(cluster=w462, "OffLineTEC"=w458, "Module"=T12."Off Line TEC") -> (w463:T7)
                                n351 = call "TL_Driver.vi"("Device In"=w456, "Commands"=T9."SET", "Settings"=w463) -> ("Readings"=w461:T6)  [unwired: 9 in, 3 out]
                                n352 = local write "Settings"(w463) -> ()
                                n353 = local write "Readings"(w461) -> ()
                                }
                              }
                            }
                          }
                          n354 = Or(x=w408, y="Cancel Offline") -> (x .or. y?=w409:bool)
                        }
                      }
                    }
                  }
                  frame #1 {
                    # "Reading the power meter"
                    # "Updating the pulse energy plot"
                    # "Converting to pulse energy"
                    # "Reading the offline output power, converting to pulse energy,  and updating the Pulse energy plot"
                    n355 = local read "SampleSize"() -> (w466:i32)
                    n356 = local read "Newport Device Key"() -> (w467:string)
                    n357 = local read "Online Pulse Energy"() -> (w473:dbl)
                    n358 = local read "Offline Pulse Energy"() -> (w472:dbl)
                    n359 = local read "NewportRef"() -> (w464:refnum<k24>)
                    n360 = Number To Decimal String(number=w466) -> (decimal integer string=w468:string)  [unwired: 1 in]
                    n361 = invoke class="PowerMeterCommands" method="PerformDAQ"(reference=w464, "deviceKey"=w467, "interval"="1", "sampleSize"=w468) -> ("PerformDAQ"=w469:dbl[])  [unwired: 2 in, 5 out]
                    n362 = Bundle("Online Pulse Energy"=w473, "Offline Pulse Energy"=w472) -> (w471:T15)  [unwired: 1 in]
                    n363 = local write "Pulse Energy (Micro Joule)"(w471) -> ()
                    n364 = call-poly <vilib>:"Mean.vi"("X"=w469) -> ("mean"=w465:dbl)  [unwired: 1 out]
                    n365 = Multiply(x=w465, y=1000.0) -> (x*y=w478:dbl)
                    n366 = Divide(x=w478, y=0.05) -> (x/y=w476:dbl)
                    n367 = Divide(x=w476, y=7.0) -> (x/y=→"Offline Pulse Energy":dbl)
                  }
                  frame #2 {
                    # "Added in the ability to interactively control the ThorLab  setting (just etalon temp for now)"
                    # "Wait 'Scalar Wait Time' for buffers to clear of online contiminated offline data"
                    n368 = disable-structure shown="Disabled" {
                      frame Disabled {
                        # "Wait 'Scalar Wait Time'"
                        n369 = local read "Scalar Wait Time"() -> (w488:u32)
                        n370 = Wait (ms)(milliseconds to wait=w488) -> ()  [unwired: 1 out]
                      }
                      frame Enabled {
                      }
                    }
                    n371 = event shown="[1] \"Settings.EtalonTEC\": Value Change" {
                      selector: _ -> [_ _]
                      dyn-events: _ -> [_ _]
                      timeout: 1 -> [_ _]
                      event Timeout {
                        n372 = event-data() -> ()  [unwired: 1 in, 2 out]
                      }
                      event "Settings.EtalonTEC": Value Change {
                        # "Generating a command string\nto update the etalon"
                        n373 = event-data() -> ()  [unwired: 1 in, 5 out]
                        n374 = local read "Settings"() -> (w484:T7)
                        n375 = Unbundle By Name(w484) -> ("EtalonTEC"=w487:dbl)
                        n376 = Bundle By Name(cluster=w484, "EtalonTEC"=w487, "Module"=T12."Etalon TEC") -> (w482:T7)
                        n377 = call "TL_Driver.vi"("Device In"=refnum<visa-resource-name> "Pro8000", "Commands"=T9."SET", "Settings"=w482) -> ("Readings"=w483:T6)  [unwired: 9 in, 3 out]
                        n378 = local write "Readings"(w483) -> ()
                        n379 = local write "Settings"(w482) -> ()
                      }
                    }
                  }
                  frame #3 {
                    w522 = 1 ("dimension size")
                    w526 = 1
                    # "Read in latest scalar card data from \n'Scalar Data' global variable that \nscaler.vi is writing to, then wait 1 sec\nfor next batch of data"
                    # "Plotting the normalized relative \nbackscatter"
                    # "Calculating the normalized relative backscatter"
                    # "Calculating/Plotting smoothed data,\ncross sections etc."
                    # "Pick off data with\nout header"
                    # "Calculate mean bin by bin mean"
                    # "Reading in 'Integration Period (Seconds)' of data"
                    # "Read the offline data from the scalar card, perform smoothing, calculate normalized relative backscatter, and plot"
                    # "File path in MATLAB script is of old dial is:\nF:\\Micropulse DIAL\\Micropulse DIAL Matlab\\\nFinal Overlap Function.mat')];"
                    # "Collects Data From Card,\nSends It To The Chart,\nAnd Saves A Copy As A\nFile If Option Selected On\nFront Panel"
                    n380 = for {
                      N: "Data Reads (number of loops)" -> [_]
                      tunnel: [w558] -> w490 mode=indexing
                      tunnel: [w557] -> w489 mode=indexing
                      n381 = global read "AMCS_Data.vi" "AMCS_Data"() -> (w559:u16[][])
                      n382 = disable-structure shown="Disabled" {
                        frame Disabled {
                          n383 = global read "Scalar_Data_4.vi" "Scalar Data 4"() -> ()  [unwired: 1 out]
                          n384 = global read "Scalar_Data_2.vi" "Scalar Data 2"() -> ()  [unwired: 1 out]
                        }
                        frame Enabled {
                        }
                      }
                      n385 = Index Array(array=w559, index (row) #1=1 ("index (row)"), index (row) #2=3 ("index (row)")) -> (element #1=w558:u16[], element #2=w557:u16[])  [unwired: 2 in]
                    }
                    n386 = local read "Total DIAL Integration Time (Minutes)"() -> (w547:i32)
                    n387 = Divide(x=w547, y="Data Reads (number of loops)") -> (x/y=w545:dbl)
                    n388 = local read "Total Aerosol Integration Time (Minutes)"() -> (w549:dbl)
                    n389 = local read "background length"() -> (w494:i32)
                    n390 = Multiply(x=w545, y=60.0) -> (x*y=w532:dbl)
                    n391 = local read "background start"() -> (w495:u32)
                    n392 = Transpose 2D Array(2D array=w490) -> (transposed array=w555:u16[][])
                    n393 = Transpose 2D Array(2D array=w489) -> (transposed array=w538:u16[][])
                    n394 = Divide(x=w549, y="Data Reads (number of loops)") -> (x/y=w550:dbl)
                    n395 = for {
                      tunnel: w555 -> [w565] mode=indexing
                      tunnel: [w564] -> w556 mode=indexing
                      tunnel: w538 -> [w563] mode=indexing
                      tunnel: [w562] -> _ mode=indexing
                      tunnel: [w562] -> w535 mode=indexing
                      n396 = call-poly <vilib>:"Mean.vi"("X"=w565) -> ("mean"=w564:dbl)  [unwired: 1 out]
                      n397 = call-poly <vilib>:"Mean.vi"("X"=w563) -> ("mean"=w562:dbl)  [unwired: 1 out]
                    }
                    n398 = local read "bins"() -> (w523:u32)
                    n399 = Multiply(x=w550, y=60.0) -> (x*y=w513:dbl)
                    n400 = Array Subset(array=w535, index=w522, length=w523) -> (w536:dbl[])
                    "Off-Line Bin Readings 2" <- w536
                    n401 = Array Subset(array=w556, index=w522, length=w523) -> (w534:dbl[])
                    "Off-Line  Bin Readings" <- w534
                    n402 = Array Subset(array=w536, index=w495, length=w494) -> (w537:dbl[])
                    n403 = Array Subset(array=w534, index=w495, length=w494) -> (w554:dbl[])
                    n404 = local read "Smoothed Bins"() -> (w491:dbl)
                    n405 = call-poly <vilib>:"Mean.vi"("X"=w537) -> ("mean"=w501:dbl)  [unwired: 1 out]
                    n406 = call-poly <vilib>:"Mean.vi"("X"=w554) -> ("mean"=w502:dbl)  [unwired: 1 out]
                    n407 = local read "Index"() -> (w512:i32)
                    n408 = Subtract(x=w536, y=w501) -> (x-y=w514:dbl[])
                    n409 = Subtract(x=w534, y=w502) -> (x-y=w530:dbl[])
                    n410 = call "Ring Buffer Offline Far.vi"("Index"=w512, "Profiles to Average"=w532, "Input Array"=w530) -> ("AvgArray"=w552:dbl[], "RingBufferOut"=→"RingBuffer offline far":dbl[][])  [unwired: 7 in]
                    n411 = call "Ring Buffer Aerosol Far.vi"("Index"=w512, "Profiles to Average"=w513, "Input Array"=w530) -> ("AvgArray"=w548:dbl[], "RingBufferOut"=→"RingBuffer aerosol far":dbl[][])  [unwired: 7 in]
                    n412 = call "Ring Buffer Offline Near.vi"("Index"=w512, "Profiles to Average"=w532, "Input Array"=w514) -> ("AvgArray"=w533:dbl[], "RingBufferOut"=→"RingBuffer offline near":dbl[][])  [unwired: 7 in]
                    n413 = call "Ring Buffer Aerosol Near.vi"("Index"=w512, "Profiles to Average"=w513, "Input Array"=w514) -> ("AvgArray"=w510:dbl[], "RingBufferOut"=→"RingBuffer aerosol near":dbl[][])  [unwired: 7 in]
                    n414 = Reshape Array(w530, w522, w523) -> (→"raw counts":dbl[][])
                    n415 = Reshape Array(w514, w522, w523) -> (→"raw counts near":dbl[][])
                    n416 = call "Smooth Arrray.vi"("smooth size"=w491, "Raw Array"=w552) -> ("Smoothed Array"=→"Off-Line Smoothed":dbl[])  [unwired: 9 in]
                    n417 = call "Smooth Arrray.vi"("smooth size"=w491, "Raw Array"=w548) -> ("Smoothed Array"=w521:dbl[])  [unwired: 9 in]
                    "Aerosol Smoothed" <- w521
                    n418 = call "Smooth Arrray.vi"("smooth size"=w491, "Raw Array"=w533) -> ("Smoothed Array"=→"HSRL combined":dbl[])  [unwired: 9 in]
                    n419 = call "Smooth Arrray.vi"("smooth size"=w491, "Raw Array"=w510) -> ("Smoothed Array"=w493:dbl[])  [unwired: 9 in]
                    "HSRL combined Smoothed" <- w493
                    n420 = local read "Number of Accumulates"() -> (w497:u32)
                    n421 = local read "Temperature (C)"() -> (w544:dbl)
                    n422 = local read "Pressure (mb)"() -> (w543:dbl)
                    n423 = script code="%accum_num=10000;     % scaler card setting number of accumulations\nt_bin = 500e-9                 % scaler card setting time per bin\n%t_d = 37.3e-9;                % APD dead time from spec sheet\n\n% conversion from accumulated counts to count rate  (c/s)\nc_convert = 1./t_bin./accum_num;\nCR_far = p_raw_far.*c_convert;\nCR_near = p_raw_near.*c_convert;\nCR_total_far = (p_raw_far+b_far).*c_convert;\nCR_total_near = (p_raw_near+b_near).*c_convert;\nb_CR_far =b_far.*c_convert;\nb_CR_near =b_near.*c_convert;\n\n% create a range array\nsize_p =  size(p_raw_far,2);\nr = (75:75:size_p*75)./1e3; \n    \n%APD correction factor\n D_far = 1./(1-(t_d*CR_total_far));\n D_near = 1./(1-(t_d*CR_total_near));\n\n %Calculating normalize relative backscatter profile\n nrb_far = CR_far.*D_far.*r.^2.*1e-6;\n nrb_near = CR_near.*D_near.*r.^2.*1e-6;"("E"=6.0 ("Real"), "temp"=w544, "press"=w543, "p_raw_far"=w521, "b_far"=w502, "b_near"=w501, "p_raw_near"=w493, "accum_num"=w497, "t_d"="dead time") -> ("nrb_far"=w516:cdb[], "D_far"=w507:dbl[], "nrb_near"=w515:cdb[], "D_near"=w506:dbl[], "b_CR_far"=w499:dbl, "b_CR_near"=w498:dbl)  [unwired: 1 in, 1 out]
                    n424 = local read "bins"() -> (w525:u32)
                    n425 = local read "Altitude Array (km)"() -> (w518:dbl[])
                    n426 = Bundle(w499, w498) -> (→"?":cluster{dbl, dbl})  [unwired: 1 in]
                    n427 = Build Array(w516, w515) -> (w520:cdb[][])
                    n428 = Build Array(w507, w506) -> (w505:dbl[][])
                    n429 = Reshape Array(w515, w526, w525) -> (→"NRB 2":cdb[][])
                    n430 = Reshape Array(w516, w526, w525) -> (→"NRB":cdb[][])
                    n431 = Build Array(w518, w518) -> (w517:dbl[][])
                    n432 = call "Convert to Dynamic Data7"("2D Array"=w505) -> ("Dynamic Data Type"=w504:dynamicdata)  [unwired: 3 in]
                    n433 = call "Convert to Dynamic Data3"("2D Array"=w520) -> ("Dynamic Data Type"=w519:dynamicdata)  [unwired: 3 in]
                    n434 = call "Convert to Dynamic Data4"("2D Array"=w517) -> ("Dynamic Data Type"=w508:dynamicdata)  [unwired: 3 in]
                    n435 = call "Build XY Graph2"("Y Input"=w508, "X Input"=w519) -> ("XY Graph"=→"NRB plot":cluster{"Y":dbl[], "Y":dbl[]}[])  [unwired: 3 in, 6 out]
                    n436 = call "Build XY Graph4"("Y Input"=w508, "X Input"=w504) -> ("XY Graph"=→"Correction":cluster{"Y":dbl[], "Y":dbl[]}[])  [unwired: 3 in, 6 out]
                  }
                  frame #4 {
                    # "REPLACE WITH NEW AGILTRON TASK!"
                    # "Toggle Agiltron switch to online DBR"
                    n437 = disable-structure shown="Disabled" {
                      frame Disabled {
                        # "ABSORBING"
                        n438 = flat-sequence {
                          frame #0 {
                            # "Third one"
                            # "Command the switch to switch to position 1\ncorresponding to the online DBR"
                            # "Hex string command \ncorrespond to online"
                            n439 = local read "Switch Comm Port"() -> (w569:refnum<visa-resource-name>)
                            n440 = VISA Write(VISA resource name=w569, write buffer="\u0001\u0012\u0000\u0002") -> ()  [unwired: 1 in, 3 out]
                          }
                        }
                        n441 = Build Array(FALSE ("Boolean")) -> (w568:bool[])
                        n442 = call-poly <vilib>:"DAQmx Write.vi"("task/channels in"=refnum<k21> "AgiltronSwitch", "data"=w568) -> ()  [unwired: 11 in, 3 out]
                      }
                      frame Enabled {
                      }
                    }
                  }
                  frame #5 {
                    # "If 'Save Data?' is true, save all relavant offline info"
                    n443 = local read "Save Data?"() -> (w571:bool)
                    n444 = case shown="True" w571 {
                      frame False {
                        # "'Save Data?' is false, do nothing"
                      }
                      frame True {
                        # "Write only one data file at this time"
                        # "Retrive Julian Date"
                        # "'Save Data?' is true, save offline data to the Data Disk"
                        n445 = local read "Lambda Off DBR Current"() -> (w593:dbl)
                        n446 = local read "Off-Line Bin Readings 2"() -> (w590:dbl[])
                        n447 = local read "Lambda Off Read (nm)"() -> (w592:dbl)
                        n448 = local read "Off-Line  Bin Readings"() -> (w598:dbl[])
                        n449 = local read "Relative Humdity (%)"() -> (w597:dbl)
                        n450 = local read "Offline Pulse Energy"() -> (w594:dbl)
                        n451 = local read "Temperature (C)"() -> (w595:dbl)
                        n452 = local read "Pressure (mb)"() -> (w596:dbl)
                        n453 = call "Julian_Date_2.vi"() -> ("Julian Date"=w591:dbl)  [unwired: 11 in]
                        n454 = Build Array (concatenate)(w591, w592, w593, w594, w595, w596, w597, w598) -> (w576:dbl[])
                        n455 = Build Array (concatenate)(w591, w592, w593, w594, w595, w596, w597, w590) -> (w573:dbl[])
                        n456 = local read "FF_Off_Ref"() -> (w578:refnum<file>)
                        n457 = local read "NF_Off_Ref"() -> (w575:refnum<file>)
                        n458 = local read "FF_Off_Ptr"() -> (w577:i64)
                        n459 = local read "NF_Off_Ptr"() -> (w574:i64)
                        n460 = Set File Position(offset (in bytes) (0)=w577, refnum=w578) -> (refnum out=w589:refnum<file>, error out=w587:errorcluster)  [unwired: 2 in]
                        n461 = Set File Position(offset (in bytes) (0)=w574, refnum=w575) -> (refnum out=w585:refnum<file>, error out=w583:errorcluster)  [unwired: 2 in]
                        n462 = Write to Binary File(file (use dialog)=w589, data=w576, error in=w587, 5:FALSE ("prepend array or string size? (T)")) -> (refnum out=w588:refnum<file>, error out=w586:errorcluster)  [unwired: 2 in, 1 out]
                        n463 = Write to Binary File(file (use dialog)=w585, data=w573, error in=w583, 5:FALSE ("prepend array or string size? (T)")) -> (refnum out=w584:refnum<file>, error out=w582:errorcluster)  [unwired: 2 in, 1 out]
                        n464 = Get File Position(4:w586, 7:w588) -> (2:w579:i64)  [unwired: 2 out]
                        n465 = Get File Position(4:w582, 7:w584) -> (2:w572:i64)  [unwired: 2 out]
                        n466 = local write "FF_Off_Ptr"(w579) -> ()
                        n467 = local write "NF_Off_Ptr"(w572) -> ()
                      }
                    }
                  }
                }
              }
              frame #4 {
                n468 = First Call?() -> (First Call?: T/F=w601:bool)
                n469 = Or(x="calculate absorption cross sections", y=w601) -> (x .or. y?=w599:bool)
                n470 = case shown="True" w599 {
                  frame False {
                  }
                  frame True {
                    # "calculate absorption cross sections from HITRAN data base"
                    n471 = local read "Off-Line Smoothed"() -> (w602:dbl[])
                    n472 = local read "Lambda On Read (nm)"() -> (w605:dbl)
                    n473 = local read "Lambda Off Set (nm)"() -> (w608:dbl)
                    n474 = local read "Temperature (C)"() -> (w606:dbl)
                    n475 = local read "Pressure (mb)"() -> (w607:dbl)
                    n476 = script code="hitran = dlmread('C:\\Users\\H2ODial\\Desktop\\Shared Telescope WV DIAL Code\\Libraries and VIs\\815nm_841nm_HITRAN_2008.csv', ',',[1 1 1676 8]);\n%hitran = dlmread('C:\\Users\\H2ODial\\Desktop\\Shared Telescope WV DIAL Code\\Libraries and VIs\\824nm_841nm_H2O.csv', ',',[0 1 352 7]);\n%hitran = dlmread('C:\\Users\\H2ODial\\Desktop\\Shared Telescope WV DIAL Code\\Libraries and VIs\\824nm_841nm_H2O_Spectral_Calc.csv', ',',[1 1 1209 7]);\n\n%Range vector in meters\nrange = ([75:75:size(Online,2)*75]);\n\nif lambda< 828\nlambda=828.195;\nelse\nlambda=lambda;\nend;\n\n%%\n\n%Voigt profile calculation\nWNmin = 1/(828+4)*1e7;  % 832.0 nm converted to wavenumber\nWNmax = 1/(828-4)*1e7;  % 824.0 nm converted to wavenumber\n\n%Find lines from WNmin to WNmax to calculate voigt profile\nline_indices = hitran(1:size(hitran,1),1)>WNmin & hitran(1:size(hitran,1),1)<WNmax;\n\nline = double(hitran(line_indices, 1:size(hitran,2)));\n\n%Calculate temperature and pressure profile\nT0 = 273+25; % surface temperature\nT0 = 273+T0_C;\nT = T0-0.0065.*range; % set to match the sounding\n\n% pressure in atmospheres\nP0  = 0.83; % surface pressure\nP0  = P0_mb/1000*0.986; %pressure in mb converted to atm\nP = P0.*(T0./T).^-5.5;   % set this value to match sounding\n\nT00 = 296;              % HITRAN reference temperature [K]\nP00 = 1;                % HITRAN reference pressure [atm]\nnu0_0 = line(:,1);      % absorption line center wavenumber from HITRAN [cm^-1]\nS0 = line(:,2);         % initial linestrength from HITRAN [cm^-1/(mol*cm^-2)]   \ngammal0 = line(:,4);    % air-broadened halfwidth at T_ref and P_ref from HITRAN [cm^-1/atm]\ngamma_s = line(:,5);    % self-broadened halfwidth at T_ref and P_ref from HITRAN [cm^-1/atm]\nE = line(:,6);          % ground state transition energy from HITRAN [cm^-1]  \nalpha = line(:,7);      % linewidth temperature dependence factor from HITRAN\ndelta = line(:,8);      % pressure shift from HiTRAN [cm^-1 atm^-1]\n\nnu_on = 1/(lambda)*1e7;\nnu_off = 1/(lambda_off)*1e7;\n\nfor i = 1:size(Online,2); % calculate the absorption cross section at each range\n  \n    nu0 = nu0_0+delta.*(P(i)./P00); % unclear if it should be Pi/P00  \n    gammal = gammal0.*(P(i)./P00).*((T00./T(i)).^alpha);    %Calculate Lorentz lineweidth at P(i) and T(i)\n\n    const.m = 18.015E-3./6.022E23; % mass of a single water molecule\n    const.k_B = 1.3806488e-23; % (J/K)\n    const.c = 299792458; % (m/s) (exact)\n \n    gammad = (nu0).*((2.0.*const.k_B.*T(i).*log(2.0))./(const.m.*const.c^2)).^(0.5);  %Calculate HWHM Doppler linewidth at T(i)\n     \n    % term 1 in the Voigt profile\n    y = (gammal./gammad).*((log(2.0)).^(0.5));\n    \n    % term 2 in the Voigt profile\n    x_on = ((nu_on-nu0)./gammad).*(log(2.0)).^(0.5);\n    x_off = ((nu_off-nu0)./gammad).*(log(2.0)).^(0.5);\n    \n    %setting up Voigt convolution\n    t = (-(size(line,1))/2:1:size(line,1)/2-1); %set up the integration spectral step size\n    t = repmat(t',1,length(x_on))';\n    x_on = repmat(x_on,1,length(t));\n    x_off = repmat(x_off,1,length(t));\n    y = repmat(y,1,length(t));\n    f_on = (exp(-t.^2.0))./(y.^2.0+(x_on-t).^2.0);  % combined Voigt term 1 and 2\n    f_off = (exp(-t.^2.0))./(y.^2.0+(x_off-t).^2.0);\n    %Voigt integration over all of the lines at the on and offline locations\n    z_on = trapz(t(1,:),f_on,2);\n    z_off =  trapz(t(1,:),f_off,2);\n    integral_on = z_on;\n    integral_off = z_off;\n    %Calculate linestrength at temperature T\n    S = S0.*((T00./T(i)).^(1.5)).*exp(1.439.*E.*((1./T00)-(1./T(i))));\n \n    %Calculate the Voigt profile\n    K_on = (y(:,1)./pi).*integral_on;\n    K_off = (y(:,1)./pi).*integral_off;\n    \n    %Calculate the Voigt profile absorption cross section [cm^2]\n    sigmav_on = S.*(1./gammad).*(((log(2.0))./pi).^(0.5)).*K_on; %.*far_wing_on;\n    sigmav_off = S.*(1./gammad).*(((log(2.0))./pi).^(0.5)).*K_off; %.*far_wing_off;\n    \n    %Sum contributions from all of the surrounding lines\n    sigma_on_total(i) = sum(sigmav_on);\n    sigma_off_total(i) = sum(sigmav_off);\n    \nend;"("lambda"=w605, "lambda_off"=w608, "P0_mb"=w607, "T0_C"=w606, "Online"=w602) -> ("sigma_on_total"=→"sigma_on_total":dbl[], "sigma_off_total"=→"sigma_off_total":dbl[])  [unwired: 1 in, 1 out]
                  }
                }
              }
              frame #5 {
                w619 = 1
                # "normalization factor\nfrom 300 to 450m"
                # "OPTICAL DEPTH PLOT"
                # "new rainbow color bar display"
                # "Data Processing Far Channel"
                # "new rainbow color bar display"
                # "Calculating the range resolved water vapor number density and plotting"
                n477 = local read "sigma_off_total"() -> (w642:dbl[])
                n478 = local read "sigma_on_total"() -> (w639:dbl[])
                n479 = local read "HSRL molecular Smoothed"() -> (w641:dbl[])
                n480 = local read "On-Line  Smoothed"() -> (w617:dbl[])
                n481 = local read "Off-Line Smoothed"() -> (w616:dbl[])
                n482 = local read "HSRL combined"() -> (w640:dbl[])
                n483 = script code="%Time averaging in seconds.  600 Seconds =10 minutes\ntemporal_average = 600;\n\n%Spatial averaging in bins.  2 bins = 150 meters\nspatial_average = 2;\n\n%Creating r and r+deltar vectors..this can also be acsomplished using the\n%diff command\np_oni = Online(:,1:size(Online,2)-1);\n\np_onii = Online(:,2:size(Online,2));\n\np_offi = Offline(:,1:size(Offline,2)-1);\n\np_offii = Offline(:,2:size(Offline,2));\n\nInside = (p_oni.*p_offii)./(p_onii.*p_offi);\n\ndel_cross = 1./(2.*(sigma_on_total(1:size(Online,2)-1)-sigma_off_total(1:size(Offline,2)-1)).*75*100);\n\ndel_cross(isinf(del_cross)) = 0;\n\n%Calculating Number density\nN = del_cross.*log(Inside);\n\n%Spatial smoothing of the profiles\nfilter1 = ones(1,2)./2;\n\nN_1 = N;\n\nN_1_avg = filter2(filter1,N_1);\n\nfilter1 = ones(1,10)./10;\n\nN_2 = N;\n\nN_2_avg = filter2(filter1,N_2);\n\nN_new = zeros(size(N,1),size(N,2));\n \n%Using different averaging windows for different altitudes \nN_avg=[N_1_avg(:,1:40)';N_2_avg(:,41:size(N,2))']';\n\n\nw = N_avg.*1e6.*18.015./6.022e23"("Online"=w641, "Offline"=w640, "sigma_on_total"=w639, "sigma_off_total"=w642) -> ("N_avg"=w643:cdb[], "w"=w652:cdb[])  [unwired: 1 in, 1 out]
                n484 = script code="%Time averaging in seconds.  600 Seconds = 10 minutes\ntemporal_average = 600;\n\n%Spatial averaging in bins.  2 bins = 150 meters\nspatial_average = 2;\n\n%Creating r and r+deltar vectors..this can also be acsomplished using the\n%diff command\np_oni = Online(:,1:size(Online,2)-1);\n\np_onii = Online(:,2:size(Online,2));\n\np_offi = Offline(:,1:size(Offline,2)-1);\n\np_offii = Offline(:,2:size(Offline,2));\n\nInside = (p_oni.*p_offii)./(p_onii.*p_offi);\n\ndel_cross = 1./(2.*(sigma_on_total(1:size(Online,2)-1)-sigma_off_total(1:size(Offline,2)-1)).*75*100);\n\ndel_cross(isinf(del_cross)) = 0;\n\n%Calculating Number density\nN = del_cross.*log(Inside);\n\n%Spatial smoothing of the profiles\nfilter1 = ones(1,2)./2;\n\nN_1 = N;\n\nN_1_avg = filter2(filter1,N_1);\n\nfilter1 = ones(1,10)./10;\n\nN_2 = N;\n\nN_2_avg = filter2(filter1,N_2);\n\nN_new = zeros(size(N,1),size(N,2));\n \n%Using different averaging windows for different altitudes \nN_avg=[N_1_avg(:,1:40)';N_2_avg(:,41:size(N,2))']';\n\n \nw = N_avg.*1e6.*18.015./6.022e23"("Online"=w617, "Offline"=w616, "sigma_on_total"=w639, "sigma_off_total"=w642) -> ("N_avg"=w648:cdb[], "w"=w649:cdb[])  [unwired: 1 in, 1 out]
                n485 = local read "Time Resolution Per Bin(ns)"() -> (w618:u32)
                n486 = local read "bins"() -> (w644:u32)
                n487 = local read "Altitude Array (km)"() -> (w614:dbl[])
                n488 = Build Array(w649, w652) -> (w655:cdb[][])
                n489 = To Double Precision Float(number=w618) -> (double precision float=w637:dbl)
                n490 = Reshape Array(w648, w619, w644) -> (w659:cdb[][])
                n491 = Reshape Array(w643, w619, w644) -> (w646:cdb[][])
                n492 = Multiply(x=0.15, y=w637) -> (x*y=w635:dbl)
                n493 = Build Array(w648, w643) -> (w653:cdb[][])
                n494 = Divide(x=300.0, y=w635) -> (x/y=w632:dbl)
                n495 = Divide(x=450.0, y=w635) -> (x/y=w631:dbl)
                n496 = Build Array(w614, w614) -> (w638:dbl[][])
                n497 = call "Convert to Dynamic Data5"("2D Array"=w655) -> ("Dynamic Data Type"=w654:dynamicdata)  [unwired: 3 in]
                n498 = call "Convert to Dynamic Data2"("2D Array"=w653) -> ("Dynamic Data Type"=w650:dynamicdata)  [unwired: 3 in]
                n499 = Divide(x=w659, y=1e+17) -> (x/y=→"Water Vapor Number Density":cdb[][])
                n500 = Divide(x=w646, y=1e+17) -> (x/y=→"Water Vapor Number Density 2":cdb[][])
                n501 = call "Convert to Dynamic Data6"("Array"=w614) -> ("Dynamic Data Type"=w615:dynamicdata)  [unwired: 3 in]
                n502 = To Long Integer(number=w632) -> (32bit integer=w630:i32)
                n503 = To Long Integer(number=w631) -> (32bit integer=w629:i32)
                n504 = call "Convert to Dynamic Data"("2D Array"=w638) -> ("Dynamic Data Type"=w651:dynamicdata)  [unwired: 3 in]
                n505 = call "Convert to Dynamic Data8"("2D Array"=w638) -> ("Dynamic Data Type"=w656:dynamicdata)  [unwired: 3 in]
                n506 = Decrement(x=w630) -> (x-1=w627:i32)
                n507 = Decrement(x=w629) -> (x-1=w628:i32)
                n508 = call "Build XY Graph"("Y Input"=w651, "X Input"=w650) -> ("XY Graph"=→"Water Vapor Number Density  2":cluster{"Y":dbl[], "Y":dbl[]}[])  [unwired: 3 in, 6 out]
                n509 = call "Build XY Graph3"("Y Input"=w656, "X Input"=w654) -> ("XY Graph"=→"Absolute Humidity":cluster{"Y":dbl[], "Y":dbl[]}[])  [unwired: 3 in, 6 out]
                n510 = Array Subset(array=w617, index=w627, length=w628) -> (w626:dbl[])
                n511 = Array Subset(array=w616, index=w627, length=w628) -> (w625:dbl[])
                n512 = call-poly <vilib>:"Mean.vi"("X"=w626) -> ("mean"=w624:dbl)  [unwired: 1 out]
                n513 = call-poly <vilib>:"Mean.vi"("X"=w625) -> ("mean"=w623:dbl)  [unwired: 1 out]
                n514 = Divide(x=w624, y=w623) -> (x/y=w622:dbl)
                n515 = Multiply(x=w616, y=w622) -> (x*y=w621:dbl[])
                n516 = Divide(x=w617, y=w621) -> (x/y=w620:dbl[])
                n517 = Natural Logarithm(1:w620) -> (0:w611:dbl[])
                n518 = Multiply(x=-1.0, y=w611) -> (x*y=w610:dbl[])
                n519 = call "Convert to Dynamic Data9"("Array"=w610) -> ("Dynamic Data Type"=w613:dynamicdata)  [unwired: 3 in]
                n520 = call "Build OD Plot"("Y Input"=w615, "X Input"=w613) -> ("XY Graph"=→"Optical Depth":cluster{"Y":dbl[], "Y":dbl[]}[])  [unwired: 3 in, 6 out]
              }
            }
          }
        }
        "L_Count" <- w128
      }
    }
  }
  n521 = case shown="True" w3 {
    frame False {
    }
    frame True {
      # "close data files"
      n522 = local read "NF_Off_Ref"() -> (w663:refnum<file>)
      n523 = local read "NF_On_Ref"() -> (w664:refnum<file>)
      n524 = local read "FF_Off_Ref"() -> (w665:refnum<file>)
      n525 = local read "FF_On_Ref"() -> (w666:refnum<file>)
      n526 = local read "WS_On/Off"() -> (w662:bool)
      n527 = case shown="True" w662 {
        frame False {
        }
        frame True {
          n528 = local read "WS visa"() -> (w667:refnum<visa-resource-name>)
          n529 = call "T_RH_P.vi"("VISA in"=w667, "WS_Commands"=enum16{"OpenWS", "ReadTRHP", "CloseWS"}."CloseWS") -> ()  [unwired: 11 in, 3 out]
        }
      }
      n530 = Close File(refnum=w666) -> ()  [unwired: 1 in, 2 out]
      n531 = Close File(refnum=w665) -> ()  [unwired: 1 in, 2 out]
      n532 = Close File(refnum=w664) -> ()  [unwired: 1 in, 2 out]
      n533 = Close File(refnum=w663) -> ()  [unwired: 1 in, 2 out]
    }
  }
  "FileHour" <- -1 ("FileHour")
  "DataOpen" <- FALSE
